vi "TopLevel_Process.vi"(7 "rendezvous ref":T11, 8 "error in":errorcluster, 9 "Str Refnum":refnum<vi>, 10 "LaunchData":refnum<user-event>, 11 "TopLevel in":refnum<class "TopLevel.lvclass">) -> (3 "TopLevel out":refnum<class "TopLevel.lvclass">)   [LabVIEW 2022 SP3, in "TopLevel.lvclass"]
uses:
  TopLevel.lvclass
  DAQWFE/LV_Source/DataTypes/TD LaunchData--cluster.ctl
  DAQWFE/LV_Source/DataTypes/TD LaunchState--enum.ctl
  Common/Controls/TD MasterConfiguration DLPC2--cluster.ctl
  Common/Controls/DLPC2_Path--Cluster.ctl
  Common/Controls/TD HeadColorPaneMappingAll--cluster.ctl
  Common/Controls/TD HeadColorPaneMapping--cluster.ctl
  Typedefs/SpitVoltages--Cluster.ctl
  Typedefs/PrimingMode APIData.ctl
  Typedefs/PurgeMode--Enum.ctl
  Typedefs/PrinterHeads--Enum.ctl
  Common/Controls/DLP_MaterialToHeadMapping--Cluster.ctl
  DLP2/DataTypes/DLP2_PrinterMaterialProperties.ctl
  Typedefs/API Event Data.ctl
  Typedefs/API Task State.ctl
  Typedefs/API Command Cluster.ctl
  Typedefs/API Command Enum.ctl
  Typedefs/Digilens Config Cluster.ctl
  Typedefs/Motor Controller Config Data.ctl
  IO/Typedefs/IO Config Data.ctl
  IO/Typedefs/DCON_DeviceConfig--Cluster.ctl
  IO/Typedefs/Channel Data.ctl
  GIS Printer/Typedefs/PrinterConfiguration--Cluster.ctl
  DAQWFE/LV_Source/Subsystems/DAQ/DataTypes/TD DAQ Settings--cluster.ctl
  DAQWFE/LV_Source/Subsystems/DAQ/DataTypes/TD DI Instrument Settings--cluster.ctl
  DAQWFE/LV_Source/Subsystems/DAQ/DataTypes/TD AI Instrument Settings--cluster.ctl
  DAQWFE/LV_Source/Subsystems/DAQ/DataTypes/TD AI InstSettings--cluster.ctl
  DAQWFE/LV_Source/Subsystems/DAQ/Process/ProcessSupport/TD SimAI Ranges--cluster.ctl
  IO/IO.lvclass
  GIS Printer/GIS Printer.lvclass
  Motor Controller/Motor Controller.lvclass
  Typedefs/Pre Purge API Data.ctl
  IO/Typedefs/ICP1-D0 Channel Names.ctl
  Typedefs/PrepurgeScanTracking--Cluster.ctl
  Database/Database.lvclass
  DLP2/DLP2.lvclass
  DAQWFE/LV_Source/Subsystems/DAQ/DataTypes/TD IO Node Definition--cluster.ctl
  DAQWFE/LV_Source/Subsystems/DAQ/DataTypes/TD DI Config--cluster.ctl
  DAQWFE/LV_Source/Subsystems/DAQ/DataTypes/TD DI Task--cluster.ctl
  DAQWFE/LV_Source/Subsystems/DAQ/DataTypes/TD DI Channel--cluster.ctl
  DAQWFE/LV_Source/Subsystems/DAQ/DataTypes/TD DO Config--cluster.ctl
  DAQWFE/LV_Source/Subsystems/DAQ/DataTypes/TD DO Channel--cluster.ctl
  DAQWFE/LV_Source/Subsystems/DAQ/DataTypes/TD AI Config--cluster.ctl
  DAQWFE/LV_Source/Subsystems/DAQ/DataTypes/TD AI Task--cluster.ctl
  DAQWFE/LV_Source/Subsystems/DAQ/DataTypes/TD AI Channel--cluster.ctl
  DAQWFE/LV_Source/Subsystems/DAQ/DataTypes/TD DataValueConversion--cluster.ctl
  DAQWFE/LV_Source/Subsystems/DAQ/DataTypes/TD AI DAQ Type--enum.ctl
  DAQWFE/LV_Source/Subsystems/DAQ/DataTypes/TD AI Force Bridge--cluster.ctl
  DAQWFE/LV_Source/Subsystems/DAQ/DataTypes/TD AO Config--cluster.ctl
  DAQWFE/LV_Source/Subsystems/DAQ/DataTypes/TD AO Channel--cluster.ctl
  DAQWFE/LV_Source/Subsystems/DAQ/DAQ.lvclass
  Common/Controls/DLPConfig_Initialization.ctl
  DLP2/DataTypes/DLP2_PrinterCompensationProperties.ctl
  DLP2/DataTypes/DLP2_PrinterHeadProperties.ctl
  Common/Controls/DLPConfig)Init_HeadPropertyAttr--Cluster.ctl
  Common/Controls/HeadHeaterTemperatureSet--Cluster.ctl
  Common/Controls/HeadHeaterTemperatureEnable--Cluster.ctl
  GIS Printer/Typedefs/PrintCmdParameters--Cluster.ctl
  GIS Printer/Typedefs/IdlePrintCmdParameters--Cluster.ctl
  Typedefs/HeadPrintData--Cluster.ctl
  IO/Typedefs/ICP2-DO Channel Names.ctl
  IO/Typedefs/ICP1-AO Channel Names.ctl
  DAQWFE/LV_Source/Support/DataQueues/DataQueues.lvclass
  <vilib>/Utility/error.llb/Trim Whitespace One-Sided.vi
  <vilib>/Utility/config.llb/Read Key (Path).vi
  Digilens DLP Gen2 UI .vi
  <userlib>/_OpenG.lib/array/array.llb/Filter 1D Array with Scalar (String)__ogtk.vi
  <vilib>/Utility/config.llb/NI_LVConfig.lvlib
panel:
  out "InkType Directory":T1[](array[typedef])
  out "data":T3={"Paths"={"DigiBit WG Design Folder"=path "", "Compensated GS Image Folder"=path "", "Nozzle GS Files Head 1"=path "", "Nozzle GS Files Head 2"=path "", "Nozzle GS Files Head 3"=path "", "Nozzle GS Files Head 4"=path "", "Nozzle GS Files Head 5"=path "", "Nozzle GS Files Head 6"=path ""}, "ColorPaneMapping"={"Head 1"={"Material"="", "ColorPane"=""}, "Head 2"={"Material"="", "ColorPane"=""}, "Head 3"={"Material"="", "ColorPane"=""}, "Head 4"={"Material"="", "ColorPane"=""}, "Head 5"={"Material"="", "ColorPane"=""}, "Head 6"={"Material"="", "ColorPane"=""}}, "Materials"=[], "ColorPlanes"=[], "SpitVoltages_Half"={"1"=0.0, "2"=0.0, "3"=0.0, "4"=0.0, "5"=0.0, "6"=0.0}, "SpitVoltages_Full"={"1"=0.0, "2"=0.0, "3"=0.0, "4"=0.0, "5"=0.0, "6"=0.0}, "SystemMode"=[], "PrimeModeConfig"=[], "Running Average Duration_s"=5.0}
  out "TO 3":bool[](array[boolean])
  out "TO 2":bool[](array[boolean])
  out "appended array":bool[](array[boolean])
  out "TO":bool[](array[boolean])
  out "error out":errorcluster
  in  "OK":bool
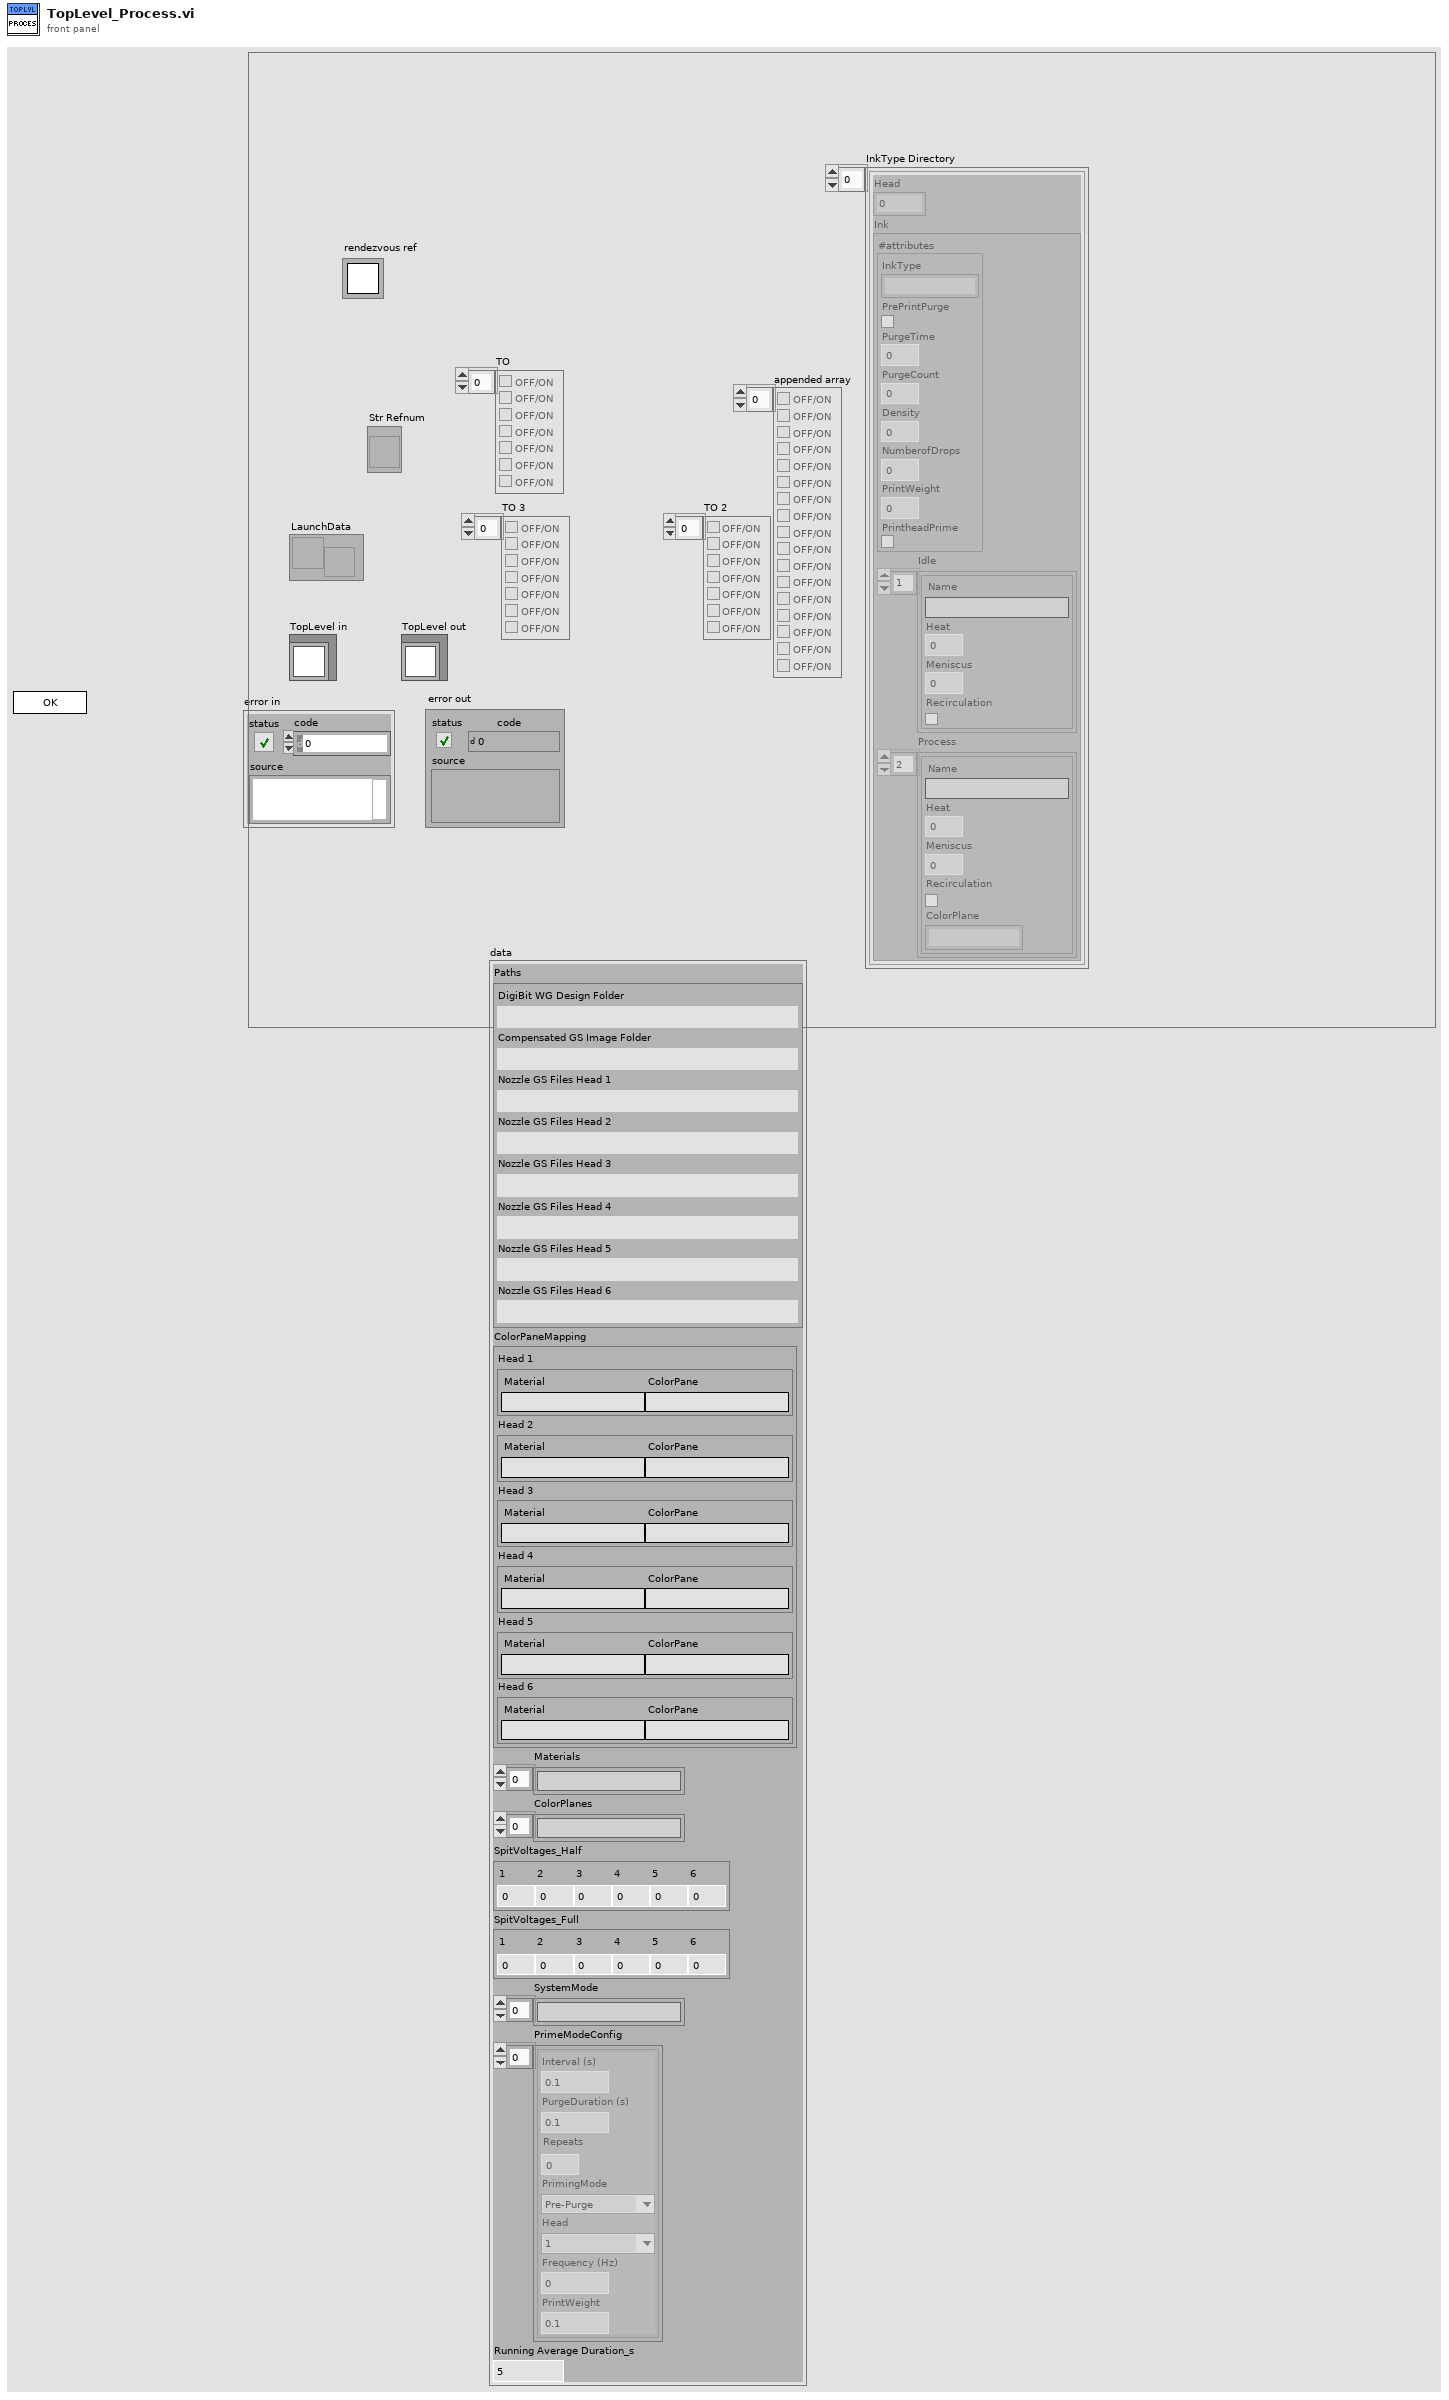
[diagram p1: front panel]
types:
  T1 = typedef "DLP_MaterialToHeadMapping--Cluster.ctl" = cluster{"Head":u8, "Ink":T2}
  T2 = typedef "DLP2_PrinterMaterialProperties.ctl" = cluster{"#attributes":cluster{"InkType":string, "PrePrintPurge":bool, "PurgeTime":dbl, "PurgeCount":i32, "Density":dbl, "NumberofDrops":i32, "PrintWeight":dbl, "PrintheadPrime":bool}, "Idle":cluster{"Name":string, "Heat":dbl, "Meniscus":dbl, "Recirculation":bool}[], "Process":cluster{"Name":string, "Heat":dbl, "Meniscus":dbl, "Recirculation":bool, "ColorPlane":string}[]}
  T3 = typedef "TD MasterConfiguration DLPC2--cluster.ctl" = cluster{"Paths":T4, "ColorPaneMapping":T5, "Materials":string[], "ColorPlanes":string[], "SpitVoltages_Half":T7, "SpitVoltages_Full":T7, "SystemMode":string[], "PrimeModeConfig":T8[], "Running Average Duration_s":dbl}
  T4 = typedef "DLPC2_Path--Cluster.ctl" = cluster{"DigiBit WG Design Folder":path, "Compensated GS Image Folder":path, "Nozzle GS Files Head 1":path, "Nozzle GS Files Head 2":path, "Nozzle GS Files Head 3":path, "Nozzle GS Files Head 4":path, "Nozzle GS Files Head 5":path, "Nozzle GS Files Head 6":path}
  T5 = typedef "TD HeadColorPaneMappingAll--cluster.ctl" = cluster{"Head 1":T6, "Head 2":T6, "Head 3":T6, "Head 4":T6, "Head 5":T6, "Head 6":T6}
  T6 = typedef "TD HeadColorPaneMapping--cluster.ctl" = cluster{"Material":string, "ColorPane":string}
  T7 = typedef "SpitVoltages--Cluster.ctl" = cluster{"1":dbl, "2":dbl, "3":dbl, "4":dbl, "5":dbl, "6":dbl}
  T8 = typedef "TopLevel.lvclass/PrimingMode APIData.ctl" = cluster{"Interval (s)":dbl, "PurgeDuration (s)":dbl, "Repeats":u8, "PrimingMode":T9, "Head":T10, "Frequency (Hz)":i32, "PrintWeight":dbl}
  T9 = typedef "PurgeMode--Enum.ctl" = enum16{"Pre-Purge", "Purge", "Spit", "Shake"}
  T10 = typedef "PrinterHeads--Enum.ctl" = enum16{"-1", "1", "2", "3", "4", "5", "6"}
  T11 = typedef "Rendezvous RefNum" = refnum<k1>
  T12 = cluster{"Initialized":bool, "LogFileFolder":path, "LogFile":path}
  T13 = typedef "TopLevel.lvclass/API Command Cluster.ctl" = cluster{"Command":T14, "Arguments":string, "Data":variant}
  T14 = typedef "TopLevel.lvclass/API Command Enum.ctl" = enum16{"Execute Printer Commands", "Pre Purge", "Enable Ink Ch-1", "Enable Ink Ch-2", "Enable Ink Ch-3", "Enable Ink Ch-4", "Enable Ink Ch-5", "Enable Ink Ch-6", "Disable Ink Ch-1", "Disable Ink Ch-2", "Disable Ink Ch-3", "Disable Ink Ch-4", "Disable Ink Ch-5", "Disable Ink Ch-6", "ExecuteIdlePrintCycle", "StopIdlePrintCycle", "Abort", "LoadDLP2GUIConfig", "SaveDLP2GUIConfig", "PrimingMode", "SetHeadTemperature", "EnableHead", "EnableHeadHeat", "SetSystemMode", "HeadPrint", "AbortAll", "Send Printer String", "WriteInitXML"}
  T15 = typedef "TopLevel.lvclass/API Event Data.ctl" = cluster{"Task":cluster{"Time Stamp":timestamp, "Timeout (ms)":u32, "Task State":T16, "Task Error":errorcluster, "Task ID":string}, "Command":variant, "Return Value":variant}
  T16 = typedef "TopLevel.lvclass/API Task State.ctl" = enum16{"Completed", "Errored", "Pending"}
  T17 = enum32{"invalid app kind", "Development System", "Run Time System", "Student Edition", "Embedded LabVIEW", "Evaluation", "Custom"}
  T18 = typedef "DLPConfig_Initialization.ctl" = cluster{"PrinterInitialization":cluster{"Printer":cluster{"#attributes":cluster{"Name":string}}, "VacPumpSet":cluster{"#attributes":cluster{"VacPumpEnable":bool, "VacPumpSpeed":dbl}}, "HIBEnable":cluster{"#attributes":cluster{"HIB1Enable":bool, "HIB2Enable":bool, "HIB3Enable":bool, "HIB4Enable":bool, "HIB5Enable":bool, "HIB6Enable":bool}}, "PrinterCompensation":T19}, "HeadSet":cluster{"HeadProperties":T20[]}, "InkSet":cluster{"Ink":T2[]}, "Troubleshooting":cluster{"PMBLogging":cluster{"#attributes":cluster{"PMBMonitorDuringPrint":bool, "PMBMonitorDuringIdle":bool, "LogSwatheInputData":bool, "LogSwatheOutputData":bool, "LogPrintheadColourPlanes":bool, "LogPMBCommunication":bool, "LogSimulatedOutput":bool, "LogAllPMBCommunicationData":bool, "LogPMBSpace":bool, "ExtendedPMBSpaceLogging":bool, "LogPMBWriteSpeed":bool, "LogUsbRetries":bool}}, "HIBLogging":cluster{"#attributes":cluster{"HIBMonitoringDuringPrint":bool, "HIBMonitoringLog":bool}}}}
  T19 = typedef "DLP2_PrinterCompensationProperties.ctl" = cluster{"#attributes":cluster{"AppName":string, "PrintWeightMultiplier":dbl, "Rotation":bool, "Driver":string, "Server":string, "Database":string, "User":string, "Password":string}}
  T20 = typedef "DLP2_PrinterHeadProperties.ctl" = cluster{"#attributes":T21}
  T21 = typedef "DLPConfig)Init_HeadPropertyAttr--Cluster.ctl" = cluster{"HeadNumber":u8, "Material":string, "HeadLocalX":dbl, "HeadLocalY":dbl, "HeadRotationAngle":dbl, "VH2L_Hi":dbl, "VH2R_Hi":dbl, "VH1LA_Hi":dbl, "VH1LB_Hi":dbl, "VH1RA_Hi":dbl, "VH1RB_Hi":dbl, "VH2L_Lo":dbl, "VH2R_Lo":dbl, "VH1LA_Lo":dbl, "VH1LB_Lo":dbl, "VH1RA_Lo":dbl, "VH1RB_Lo":dbl}
  T22 = typedef "DAQ.lvclass/TD IO Node Definition--cluster.ctl" = cluster{"DI Config":T23, "DO Config":T26, "AI Config":T28, "AO Config":T34}
  T23 = typedef "DAQ.lvclass/TD DI Config--cluster.ctl" = cluster{"DI Tasks":T24[]}
  T24 = typedef "DAQ.lvclass/TD DI Task--cluster.ctl" = cluster{"DI TaskName":string, "DI Channels":T25[]}
  T25 = typedef "DAQ.lvclass/TD DI Channel--cluster.ctl" = cluster{"DevName":string, "IOName":string, "IOPath":string, "SchemName":string, "logic":enum16{"Lo", "Hi"}, "Index":i32}
  T26 = typedef "DAQ.lvclass/TD DO Config--cluster.ctl" = cluster{"DO Channels":T27[]}
  T27 = typedef "DAQ.lvclass/TD DO Channel--cluster.ctl" = cluster{"DevName":string, "IOName":string, "IOPath":string, "SchemName":string, "logic":enum16{"Lo", "Hi"}, "DAQmx Task":refnum<k21>}
  T28 = typedef "DAQ.lvclass/TD AI Config--cluster.ctl" = cluster{"AI Tasks":T29[]}
  T29 = typedef "DAQ.lvclass/TD AI Task--cluster.ctl" = cluster{"AI TaskName":string, "AI Channels":T30[]}
  T30 = typedef "DAQ.lvclass/TD AI Channel--cluster.ctl" = cluster{"DevName":string, "IOName":string, "IOPath":string, "SchemName":string, "MinValue":dbl, "MaxValue":dbl, "Terminal Configuration":i32, "Index":i32, "Conversion":T31, "AIType":T32, "Force Bridge":T33}
  T31 = typedef "DAQ.lvclass/TD DataValueConversion--cluster.ctl" = cluster{"MaxSignal":dbl, "MinSignal":dbl, "MaxEngUnit":dbl, "MinEngUnit":dbl, "ScaleOffset":dbl, "negate":bool}
  T32 = typedef "DAQ.lvclass/TD AI DAQ Type--enum.ctl" = enum16{"Voltage", "Current", "Strain Gage", "Force Bridge"}
  T33 = typedef "DAQ.lvclass/TD AI Force Bridge--cluster.ctl" = cluster{"bridge information":cluster{"bridge configuration":i32, "voltage excitation source":i32, "voltage excitation value":dbl, "nominal bridge resistance":dbl}, "scaling information":cluster{"first electrical value":dbl, "second electrical value":dbl, "electrical units":i32, "first physical value":dbl, "second physical value":dbl, "physical units":i32}}
  T34 = typedef "DAQ.lvclass/TD AO Config--cluster.ctl" = cluster{"AO Channels":T35[]}
  T35 = typedef "DAQ.lvclass/TD AO Channel--cluster.ctl" = cluster{"DevName":string, "IOName":string, "IOPath":string, "SchemName":string, "Vmin":dbl, "Vmax":dbl, "Conversion":T31, "DAQmx Task":refnum<k21>}
  T36 = typedef "TopLevel.lvclass/Pre Purge API Data.ctl" = cluster{"Purge Channel Name":T37, "GIS File Path":path, "Duration (s)":dbl, "PurgeDuration (s)":dbl, "Repeats":u8}
  T37 = typedef "IO.lvclass/ICP1-D0 Channel Names.ctl" = enum16{"None", "Meniscus Pressure Reg PWR - R1", "Meniscus Pressure Reg PWR - R2", "Meniscus Pressure Reg PWR - R3", "Meniscus Pressure Reg PWR - R4", "Meniscus Pressure Reg PWR - R5", "Meniscus Pressure Reg PWR - R6", "Clear Stage Alarm", "Servo ON", "Purge Valve Open - R1", "Purge Valve Open - R2", "Purge Valve Open - R3", "Purge Valve Open - R4", "Purge Valve Open - R5", "Purge Valve Open - R6"}
  T38 = typedef "TopLevel.lvclass/Digilens Config Cluster.ctl" = cluster{"Motion Controller":T39, "IO Config":T40, "PrinterConfiguration":T43, "DAQ Settings":T44}
  T39 = typedef "Motor Controller.lvclass/Motor Controller Config Data.ctl" = cluster{"Motor IP Addresss":string, "Current Position":i32, "Pulse_Per_mm":i32, "PrePrint":dbl[], "Load Position_mm":i32, "Laminate Position_mm":i32}
  T40 = typedef "IO.lvclass/IO Config Data.ctl" = cluster{"DAQDevices":T41[], "DI Channels":T42[], "DO Channels":T42[], "Material Names":string[], "AI Channels":T42[], "AO Channels":T42[]}
  T41 = typedef "IO.lvclass/DCON_DeviceConfig--Cluster.ctl" = cluster{"COM":string, "DeviceName":string, "BaudRate":u32, "Number of Channels":i32, "DeviceAddress":i32, "Enable":bool}
  T42 = typedef "IO.lvclass/Channel Data.ctl" = cluster{"Channel Name":string, "Device Name":string, "Channel No":string}
  T43 = typedef "GIS Printer.lvclass/PrinterConfiguration--Cluster.ctl" = cluster{"IPAddress":string, "Move Stage on RTP Command?":bool, "Stage Move Position":string, "PH1-Prime Path":path, "PH2-Prime Path":path, "PH3-Prime Path":path, "PH4-Prime Path":path, "PH5-Prime Path":path, "PH6-Prime Path":path, "PrintScriptsFolder":path, "PurgeScriptsFolder":path, "StageScriptsFolder":path, "PH1-HeatOn Path":path, "PH2-HeatOn Path":path, "PH3-HeatOn Path":path, "PH4-HeatOn Path":path, "PH5-HeatOn Path":path, "PH6-HeatOn Path":path, "PH1-HeatOff Path":path, "PH2-HeatOff Path":path, "PH3-HeatOff Path":path, "PH4-HeatOff Path":path, "PH5-HeatOff Path":path, "PH6-HeatOff Path":path}
  T44 = typedef "DAQ.lvclass/TD DAQ Settings--cluster.ctl" = cluster{"Simulate DAQ":bool, "DI Settings":T45[], "AI Settings":T46[], "Relay IONames":string[], "AO IONames":string[], "AO NChan SingleTask":bool}
  T45 = typedef "DAQ.lvclass/TD DI Instrument Settings--cluster.ctl" = cluster{"Disable":bool, "DI TaskName":string, "DI RefreshIntv":i32}
  T46 = typedef "DAQ.lvclass/TD AI Instrument Settings--cluster.ctl" = cluster{"Disable":bool, "AI TaskName":string, "AI InstSettings":T47, "SimAI Ranges":T48}
  T47 = typedef "DAQ.lvclass/TD AI InstSettings--cluster.ctl" = cluster{"DaqRate":dbl, "NumSamples":i32}
  T48 = typedef "DAQ.lvclass/TD SimAI Ranges--cluster.ctl" = cluster{"lo":dbl, "hi":dbl}
  T49 = enum32{"Invalid", "Standard", "Closed", "Hidden", "Minimized", "Maximized"}
  T50 = typedef "HeadHeaterTemperatureSet--Cluster.ctl" = cluster{"Head":T10, "SetPoint":dbl}
  T51 = typedef "HeadHeaterTemperatureEnable--Cluster.ctl" = cluster{"Head":T10, "Enable":bool}
  T52 = typedef "PrintCmdParameters--Cluster.ctl" = cluster{"Command File Path":path, "No. of Print Repeats":i32, "HomeOnComplete":bool}
  T53 = typedef "IdlePrintCmdParameters--Cluster.ctl" = cluster{"Command File Path":path, "IdleMode":bool, "IdleCycleInterval(s)":dbl}
  T54 = typedef "TopLevel.lvclass/HeadPrintData--Cluster.ctl" = cluster{"PrintImageFile":string, "PrintPass":u8, "EncoderSource":string, "PrintGoSource":string, "Head":T10}
  T55 = typedef "IO.lvclass/ICP1-AO Channel Names.ctl" = enum16{"None", "Meniscus Pressure Set - R1", "Meniscus Pressure Set - R2", "Meniscus Pressure Set - R3", "Meniscus Pressure Set - R4", "Meniscus Pressure Set - R5", "Meniscus Pressure Set - R6", "Meniscus Vac Pump Speed"}
  T56 = typedef "IO.lvclass/ICP2-DO Channel Names.ctl" = enum16{"None", "Meniscus Valve Open - R1", "Meniscus Valve Open - R2", "Meniscus Valve Open - R3", "Meniscus Valve Open - R4", "Meniscus Valve Open - R5", "Meniscus Valve Open - R6", "Ink Flow Valve Open - R1", "Ink Flow Valve Open - R2", "Ink Flow Valve Open - R3", "Ink Flow Valve Open - R4", "Ink Flow Valve Open - R5", "Ink Flow Valve Open - R6", "SW_LED - Ink Valve - R1", "SW_LED - Ink Valve - R2", "SW_LED - Ink Valve - R3", "Recirc Pump On - R1", "Recirc Pump On - R2", "Recirc Pump On - R3", "Recirc Pump On - R4", "Recirc Pump On - R5", "Recirc Pump On - R6", "SW_LED - Ink Valve - R4", "SW_LED - Ink Valve - R5", "SW_LED - Ink Valve - R6"}
  T57 = typedef "TD LaunchData--cluster.ctl" = cluster{"Time Stamp":timestamp, "LaunchState":T58, "Error":errorcluster}
  T58 = typedef "TD LaunchState--enum.ctl" = enum16{"Started", "Stopped"}
  T59 = cluster{"Time Stamp":timestamp, "Timeout (ms)":u32, "Task State":T16, "Task Error":errorcluster, "Task ID":string}
  T60 = typedef "PrepurgeScanTracking--Cluster.ctl" = cluster{"TotalRepeats":i32, "CurrentScan":i32}
  T61 = cluster{"Core":cluster{"Current VI Reference":refnum<vi>, "Close Panel on Exit?":bool}, "TopLevel in":refnum<class "TopLevel.lvclass">, "Tasks":T15[], "TO":i32, "API Executed Event":refnum<user-event>, "API Return Event":refnum<user-event>, "Task Start ms":u32, "Current Task. Return Value":variant, "StartupPath":path, "Digilens IPLC Config":T38, "Current Task":T13, "IO":refnum<class "IO.lvclass">, "GIS Printer":refnum<class "GIS Printer.lvclass">, "Motor Controller":refnum<class "Motor Controller.lvclass">, "Printer Command File Path":path, "Pre Purge API Data":T36, "PPScanTrk":T60, "PrintScanTrk":T60, "IdleTimer":dbl, "Idle Mode":bool, "HomeOnComplete":bool, "Database":refnum<class "Database.lvclass">, "DLP2":refnum<class "DLP2.lvclass">, "MasterConfigurationDLPC2":T3, "Digilens Config File Path":path, "DLP2 ConfigPath":path, "GIS Commands":string[], "PrinterModeAPI Data":T8, "LaunchData":refnum<user-event>, "DAQConfigPath":path, "IO Nodes":T22, "DAQ":refnum<class "DAQ.lvclass">, "PMScanTrk":T60, "DLP":T18, "Str Refnum":refnum<vi>}
  T62 = typedef "NI_LVConfig.lvlib/Config Data RefNum.ctl" = refnum<k1>
  T63 = cluster{"Current VI Reference":refnum<vi>, "Close Panel on Exit?":bool}
  T64 = typedef "TD Pathnames--cluster.ctl" = cluster{"RunTimeSys?":bool, "AppFolder":path, "ExecutablePath":path, "ConfigFolder":path, "DataLogFolder":path, "SystemLogFolder":path, "SeqFolder":path, "MainStartupPathname":path, "MainUIPathname":path, "SystemEventsFile":path, "SeqEventsFile":path, "Config SettingsFile":path, "DAQ IOConfigFile":path, "SystemSimulation":bool, "DLPUIConfigFile":path, "PrinterInitXMLFile":path, "PersistentXMLFile":path, "Error Log Folder":path, "RecipeXMLFolder":path, "CalibrationRecipeXMLFolder":path}
  T65 = typedef "PersistentData--Cluster.ctl" = cluster{"ToolIdle":bool, "Meniscus Vac Pump Speed":dbl, "InkChEnable":cluster{"Enable Ink Ch-1":bool, "Enable Ink Ch-2":bool, "Enable Ink Ch-3":bool, "Enable Ink Ch-4":bool, "Enable Ink Ch-5":bool, "Enable Ink Ch-6":bool}, "HeatEnable":cluster{"Heater-1 Off":bool, "Heater-2 Off":bool, "Heater-3 Off":bool, "Heater-4 Off":bool, "Heater-5 Off":bool, "Heater-6 Off":bool}, "MiniscusPressure":cluster{"Meniscus Pressure Set - R1":dbl, "Meniscus Pressure Set - R2":dbl, "Meniscus Pressure Set - R3":dbl, "Meniscus Pressure Set - R4":dbl, "Meniscus Pressure Set - R5":dbl, "Meniscus Pressure Set - R6":dbl}, "RecircPumpFlow":cluster{"Recirc Pump Flow Set - R1":dbl, "Recirc Pump Flow Set - R2":dbl, "Recirc Pump Flow Set - R3":dbl, "Recirc Pump Flow Set - R4":dbl, "Recirc Pump Flow Set - R5":dbl, "Recirc Pump Flow Set - R6":dbl}}
  T66 = typedef "DAQ.lvclass/TD PublicEvents--cluster.ctl" = cluster{"DaqOutputCmd Ev":refnum<user-event>, "stop process":refnum<user-event>, "DAQ.AsyncCmd Event":refnum<user-event>, "DAQStateChanged Event":refnum<user-event>, "DAQ.AsyncMsg Event":refnum<user-event>, "DAQ_DO_StatusEvent":refnum<user-event>, "DIStateChangeEv":refnum<user-event>, "UI StateChanged":refnum<user-event>, "PurgeTimerEvent":refnum<user-event>}
  T67 = typedef "TopLevel.lvclass/UserEvents.ctl" = cluster{"API Incoming Event":refnum<user-event>, "API Executed Event":refnum<user-event>, "API Return Event":refnum<user-event>, "Exit Event":refnum<user-event>, "StatusChanged":refnum<user-event>, "DLP GUI Config Changed":refnum<user-event>, "AppEvent":refnum<user-event>, "Login Event":refnum<user-event>, "HeadPrimeStatusEvent":refnum<user-event>}
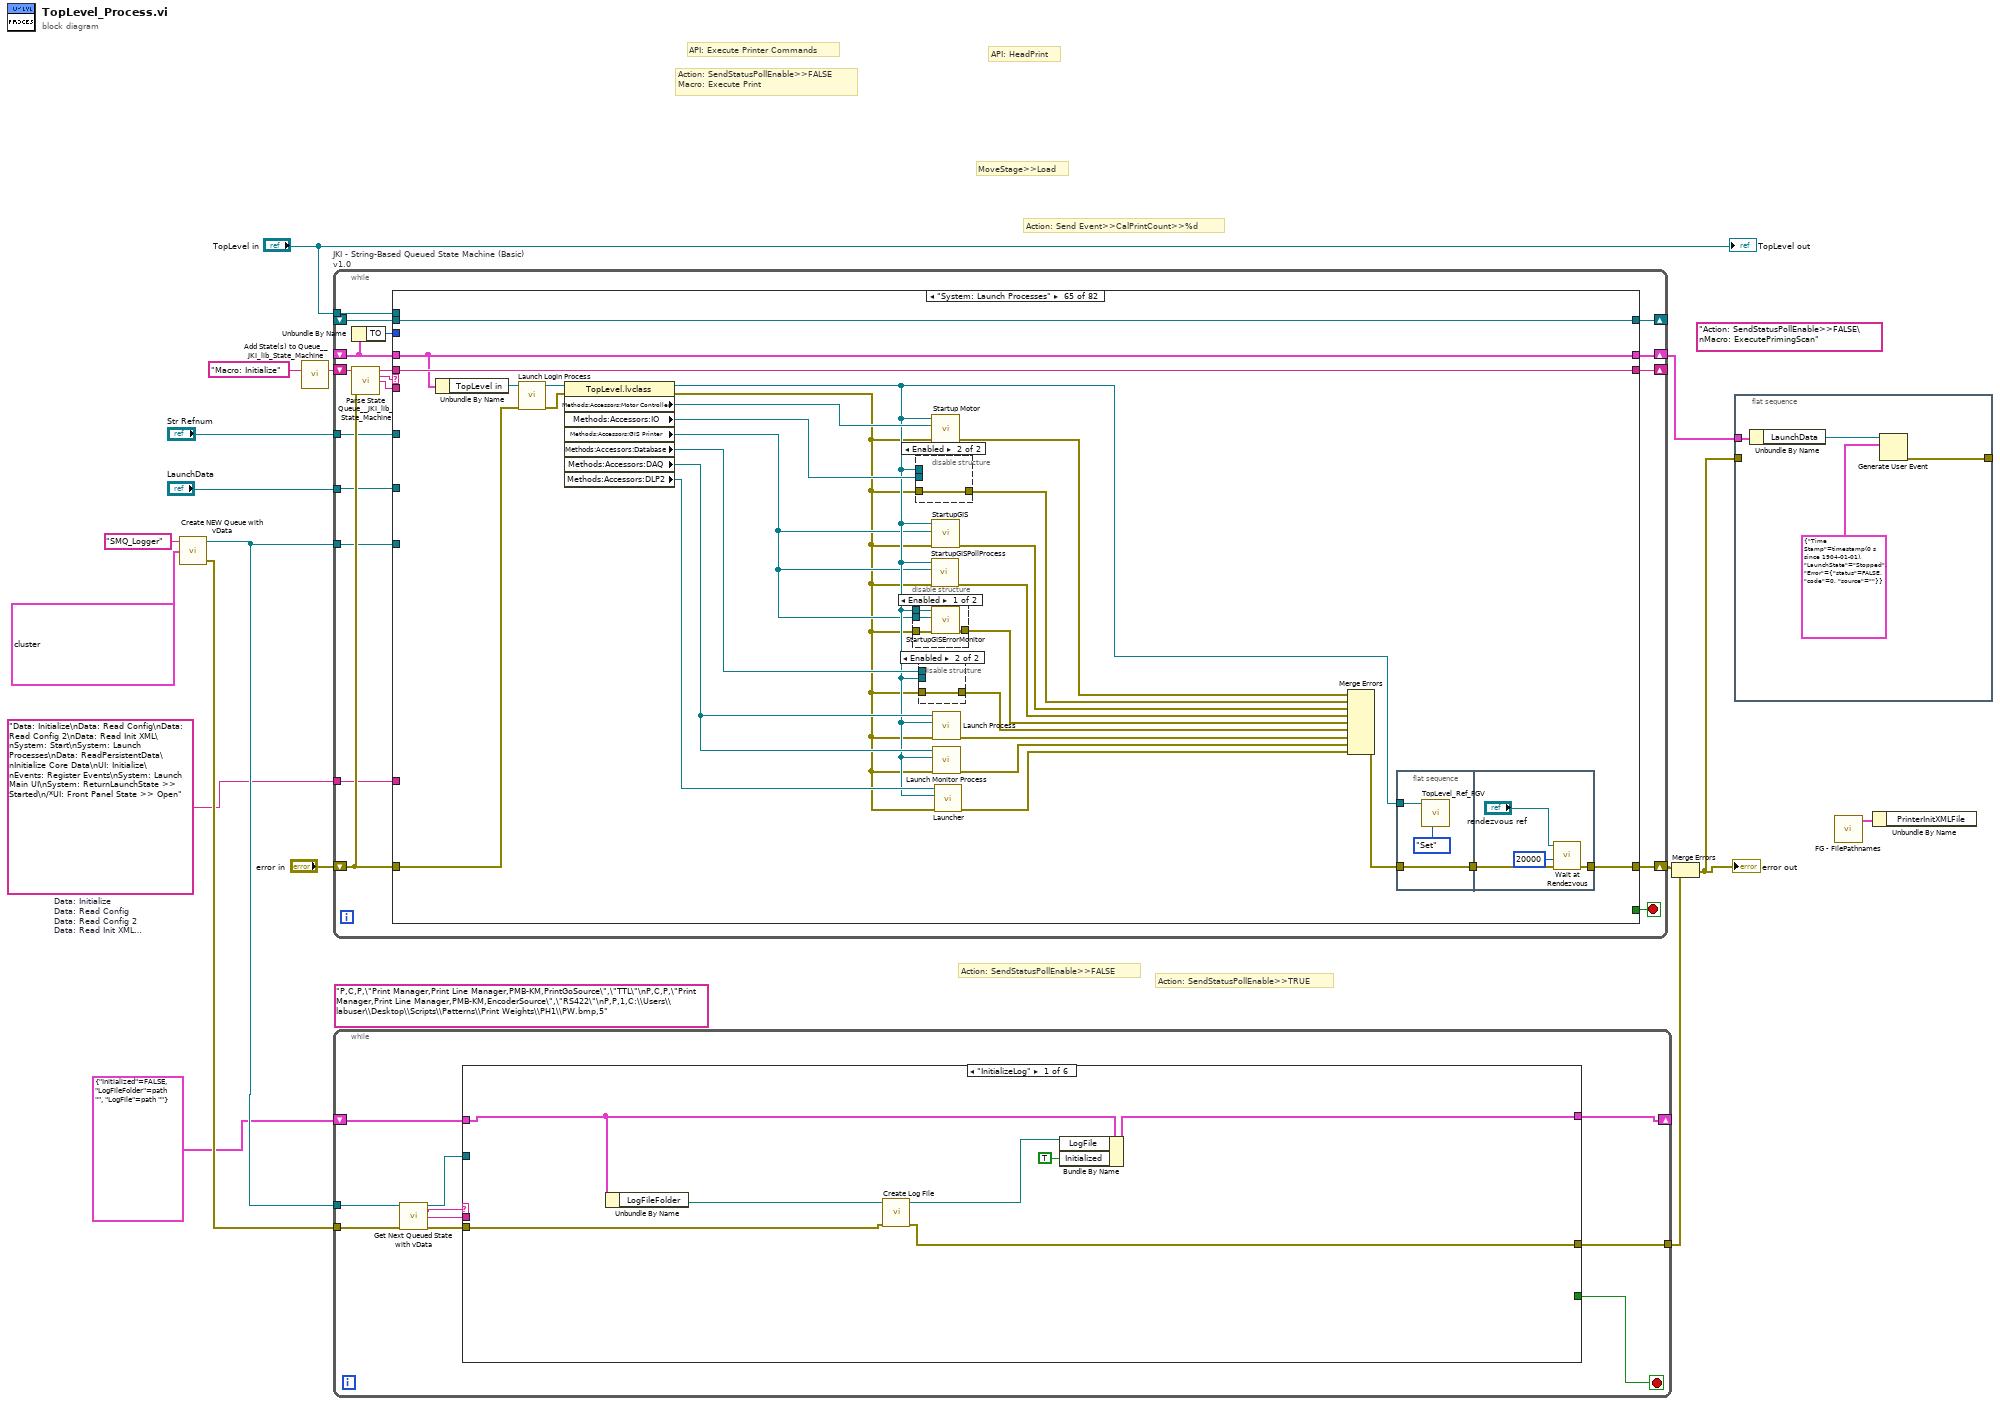
[diagram p0: block diagram]
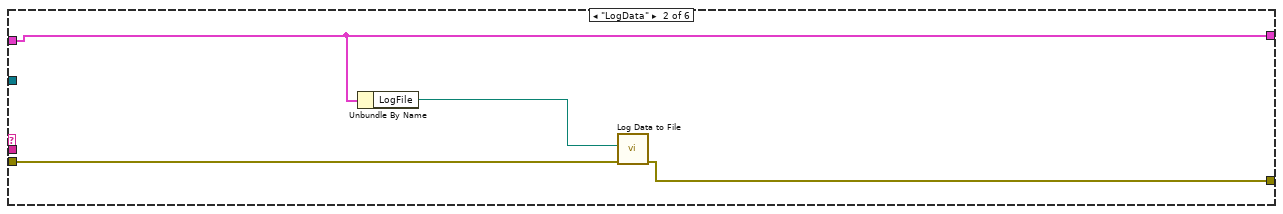
[diagram p2: hidden frame]
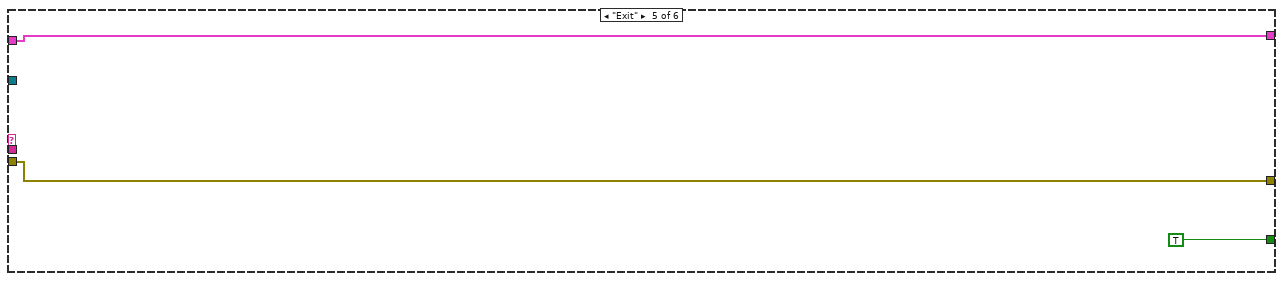
[diagram p5: hidden frame]
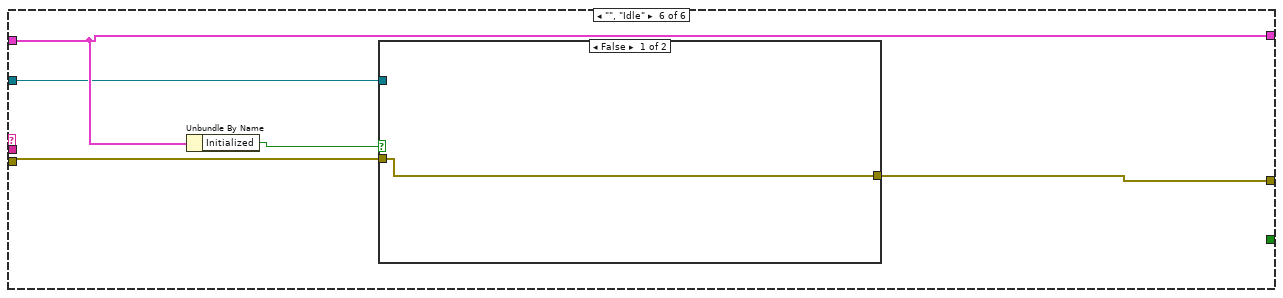
[diagram p6: hidden frame]
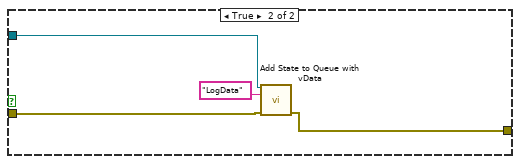
[diagram p7: hidden frame]
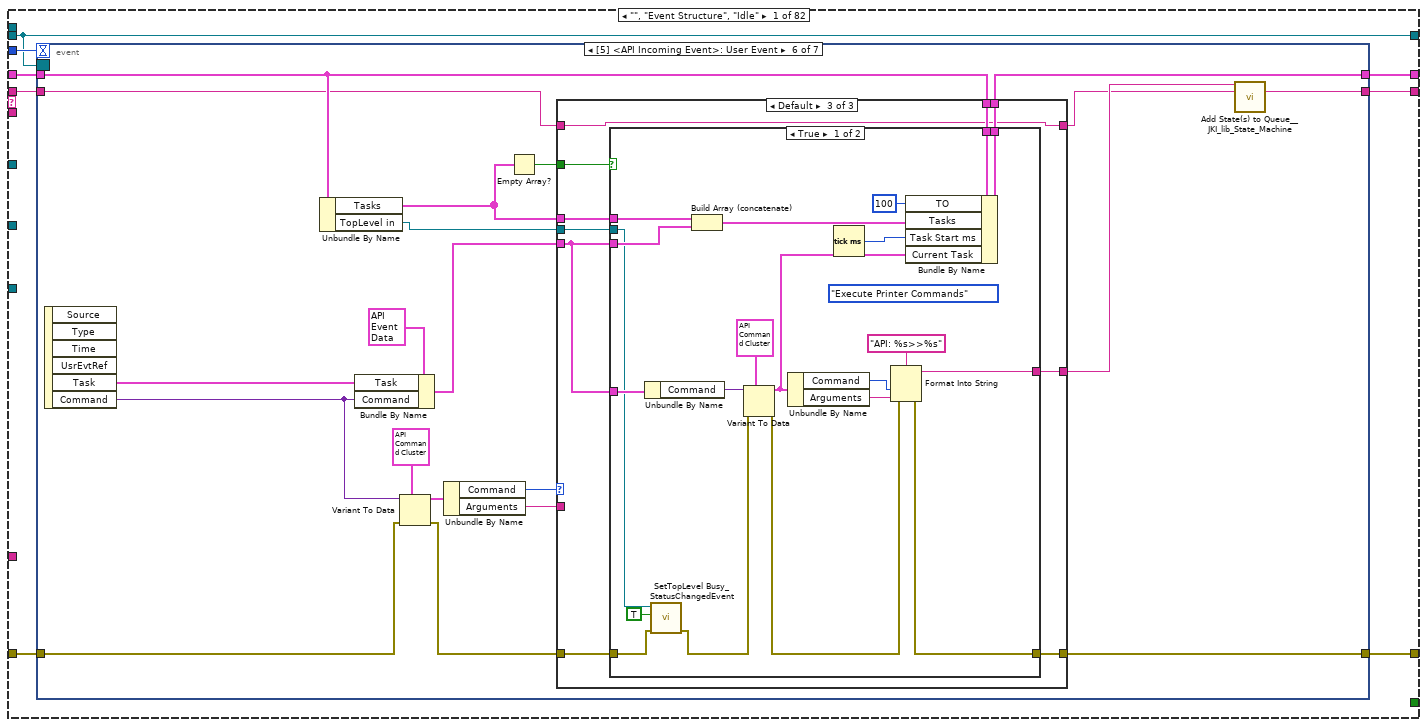
[diagram p8: hidden frame]
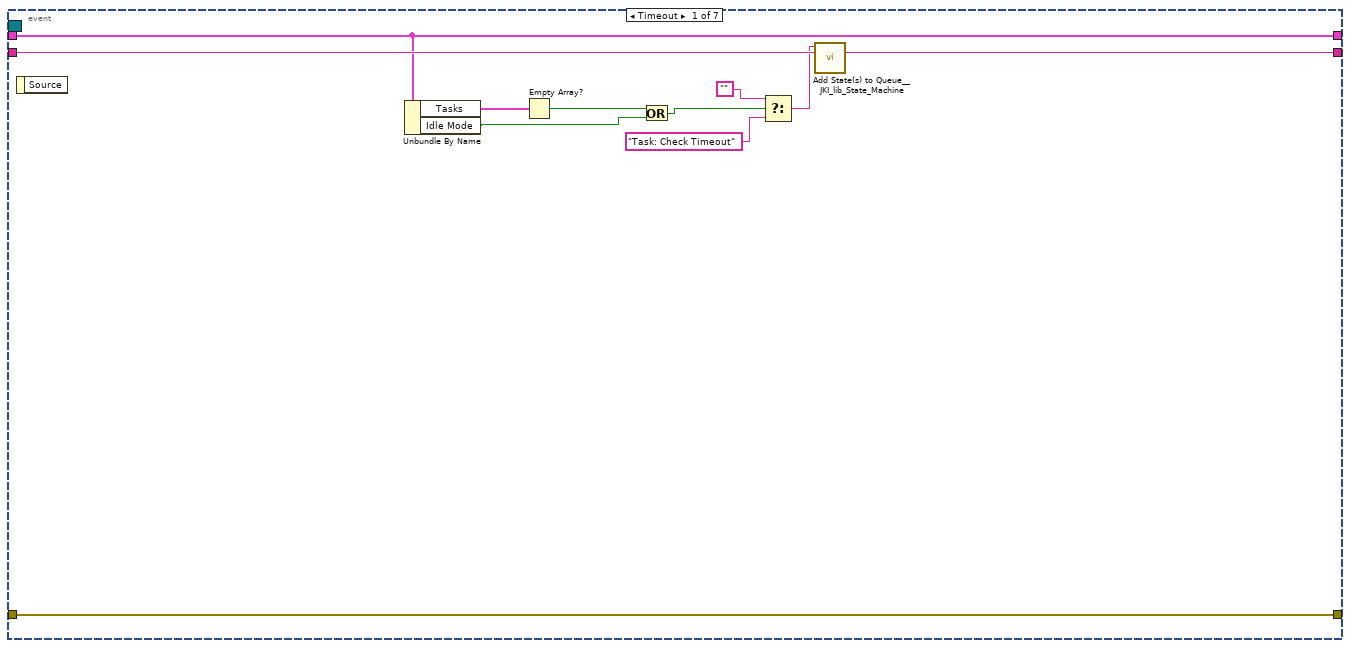
[diagram p9: hidden frame]
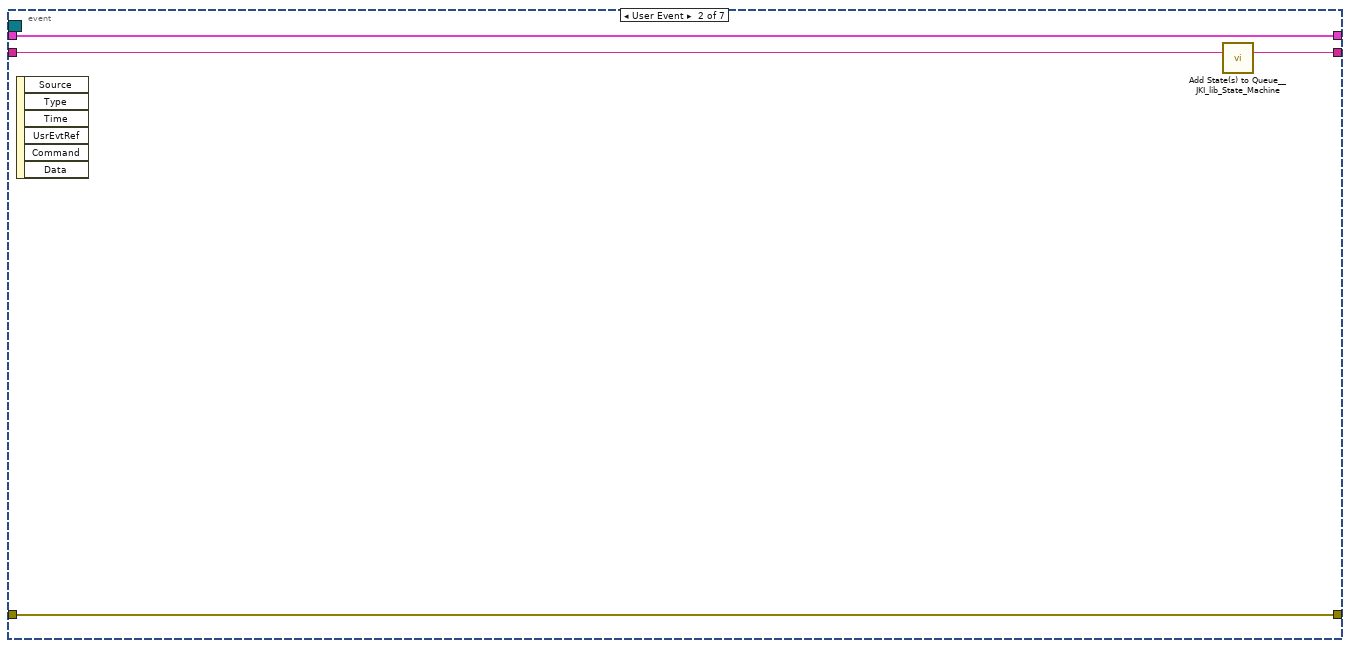
[diagram p10: hidden frame]
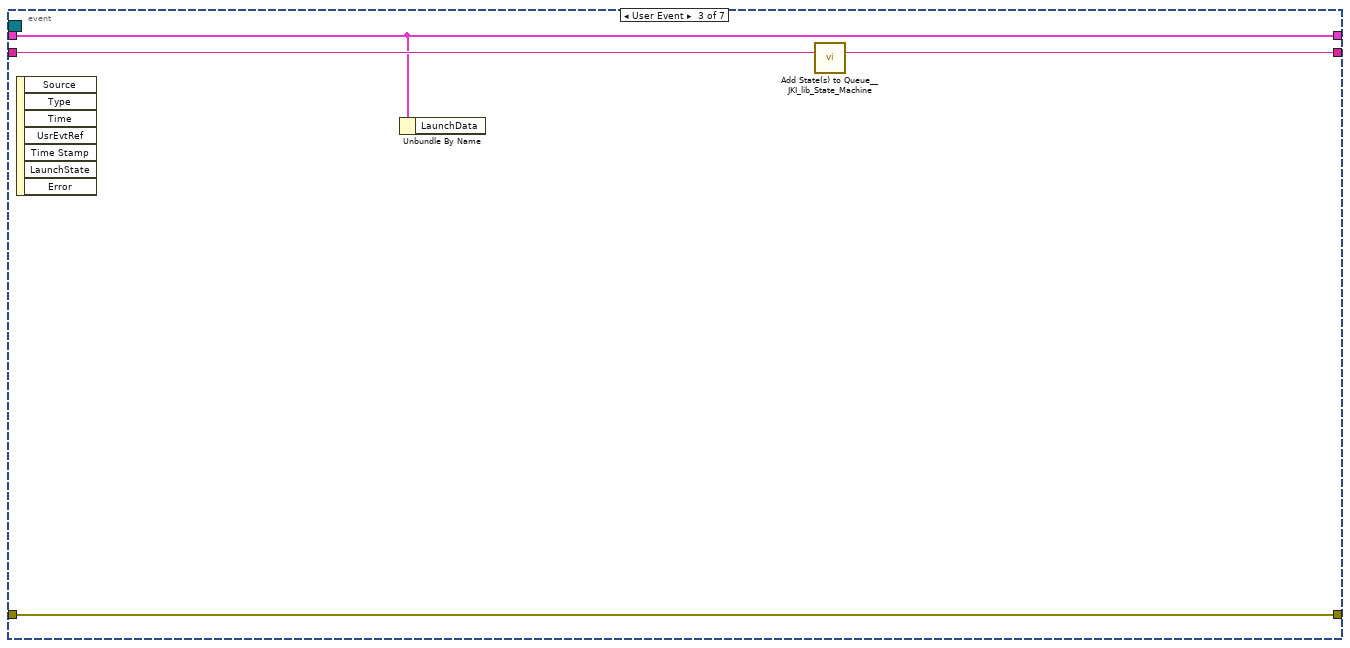
[diagram p11: hidden frame]
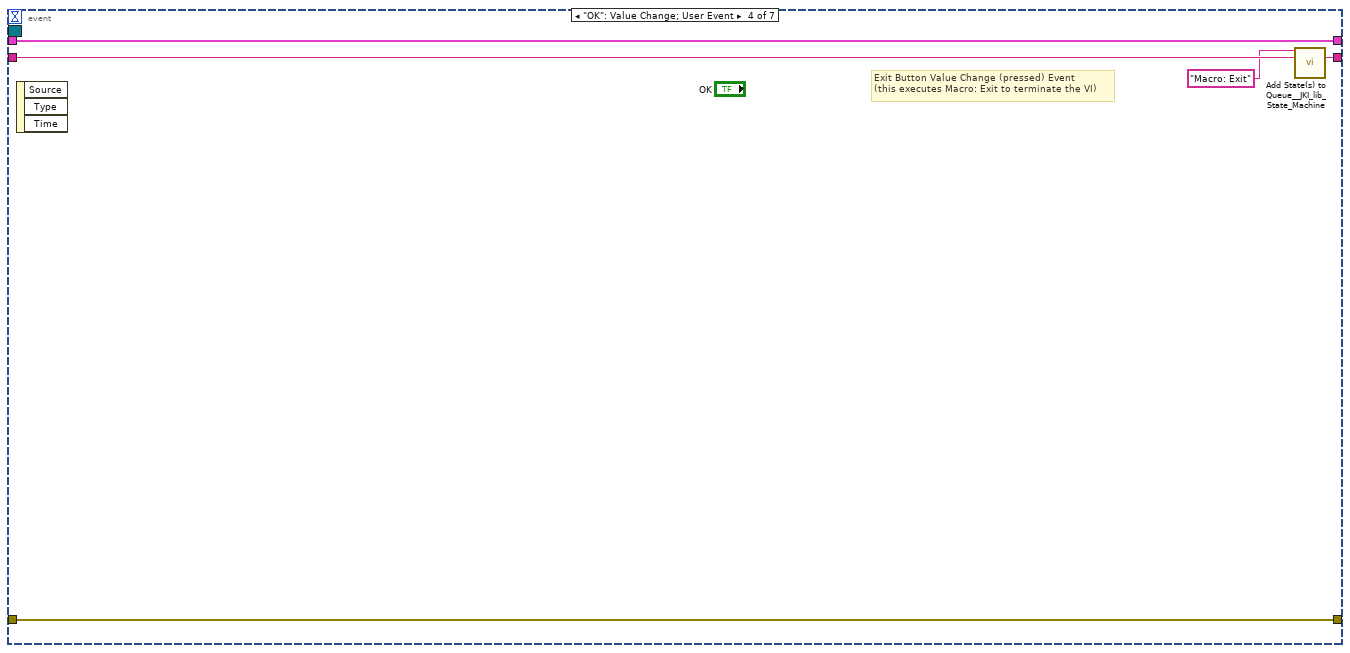
[diagram p12: hidden frame]
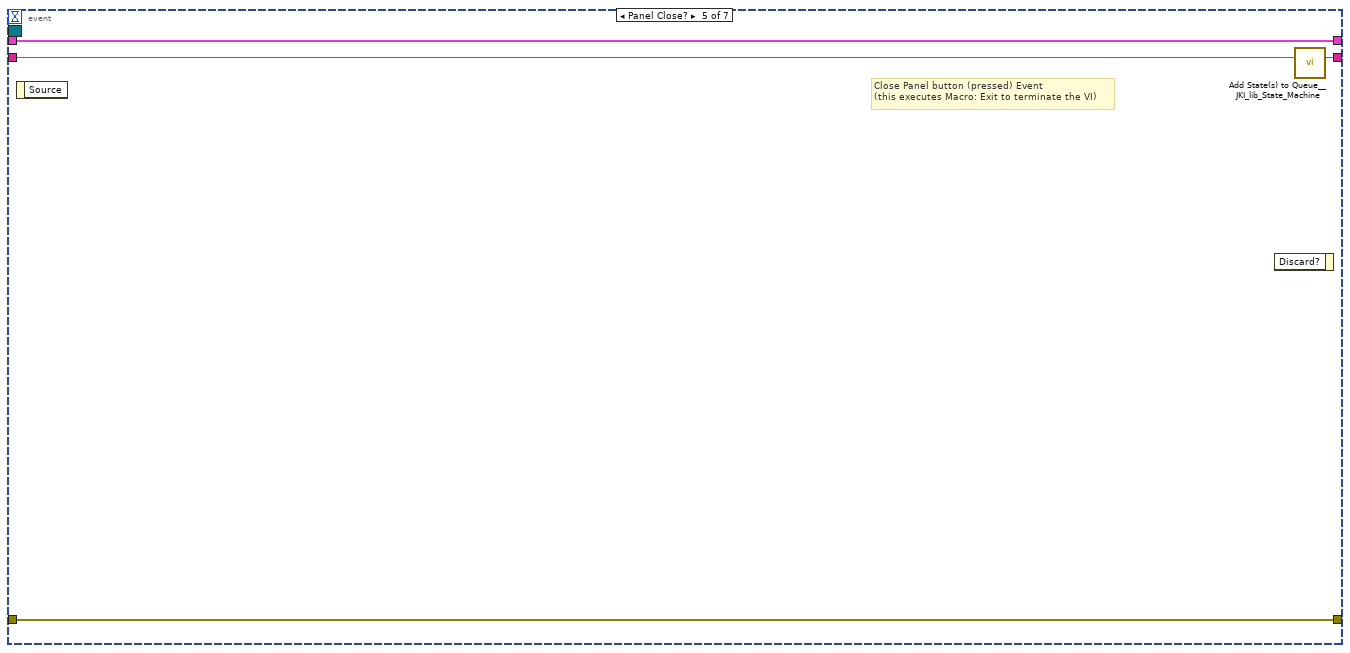
[diagram p13: hidden frame]
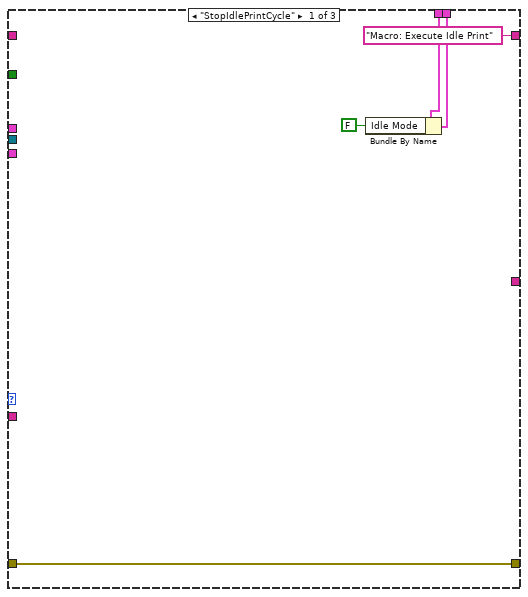
[diagram p14: hidden frame]
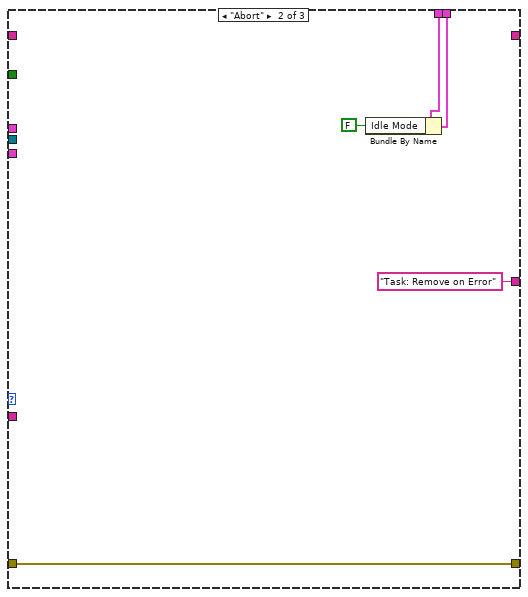
[diagram p15: hidden frame]
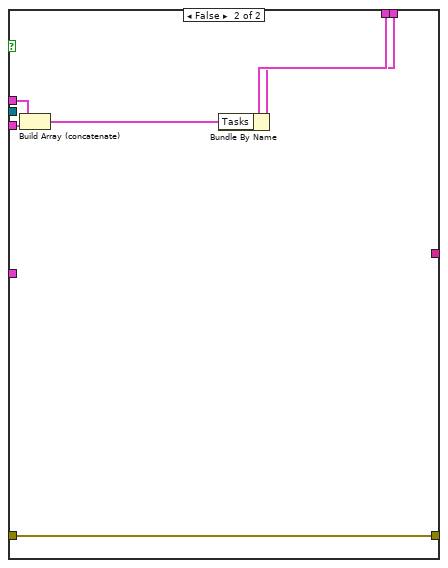
[diagram p16: hidden frame]
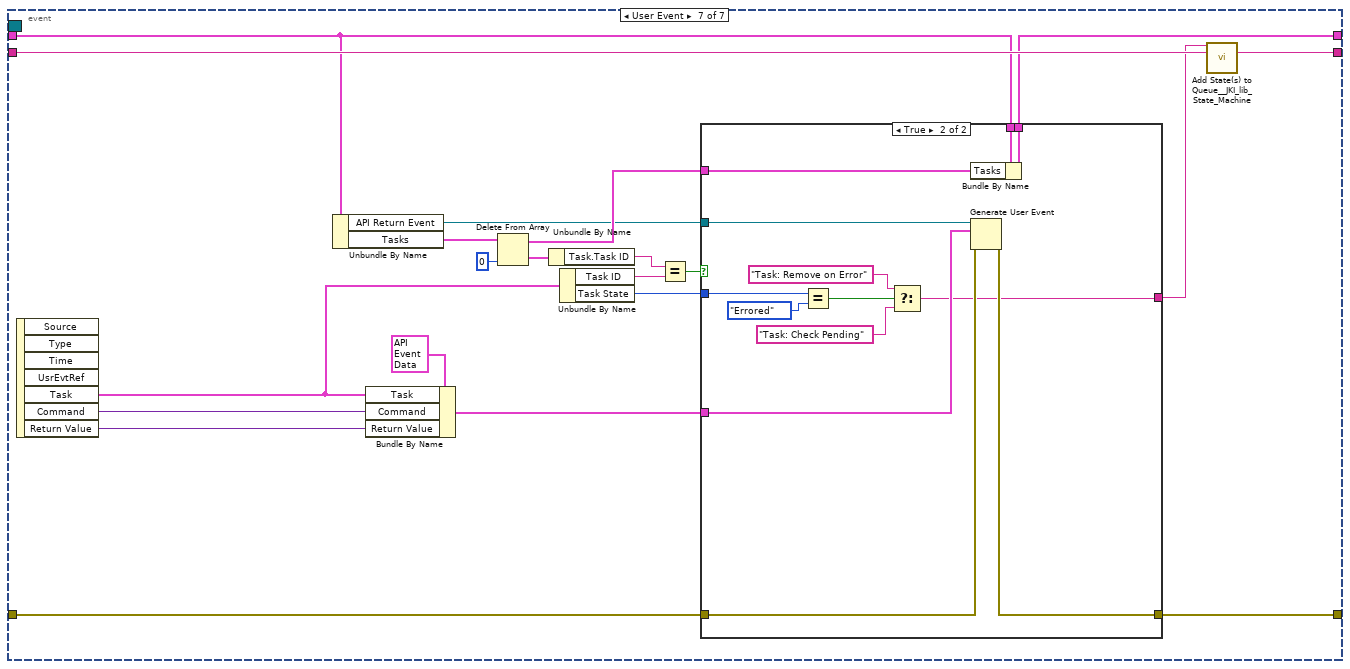
[diagram p17: hidden frame]
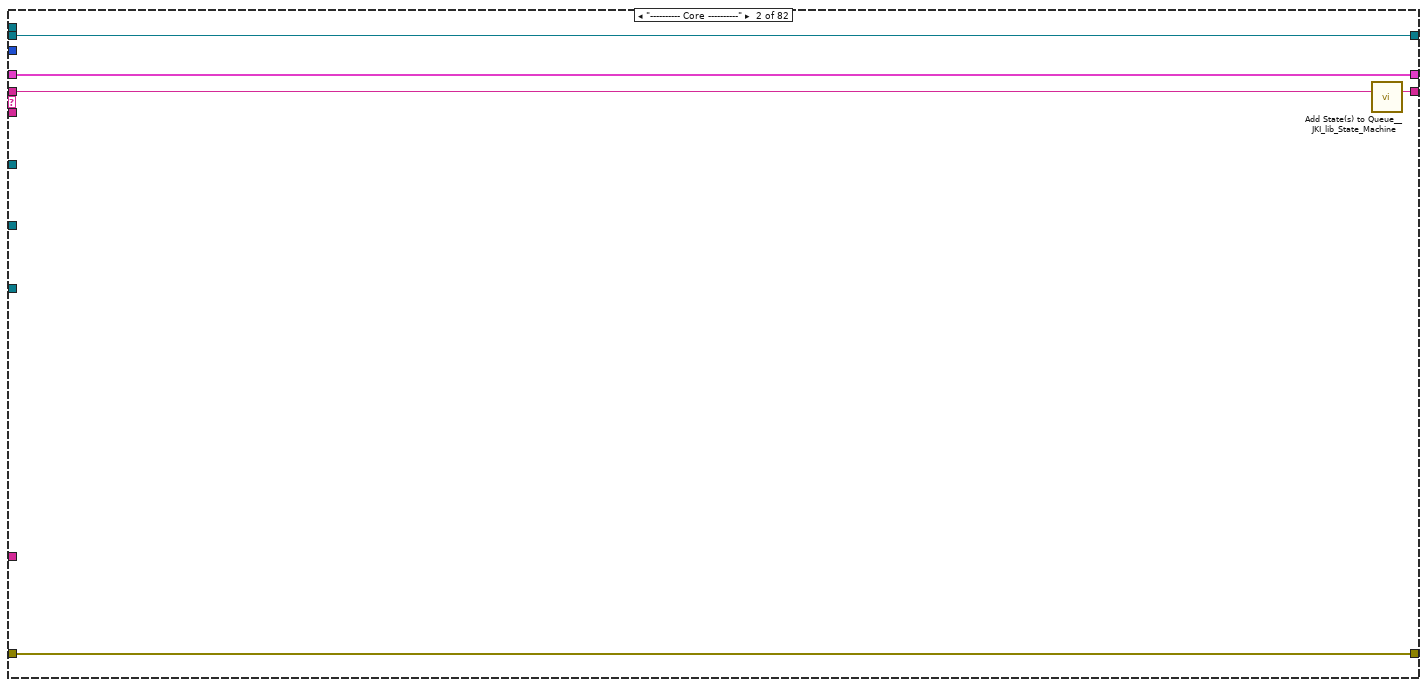
[diagram p19: hidden frame]
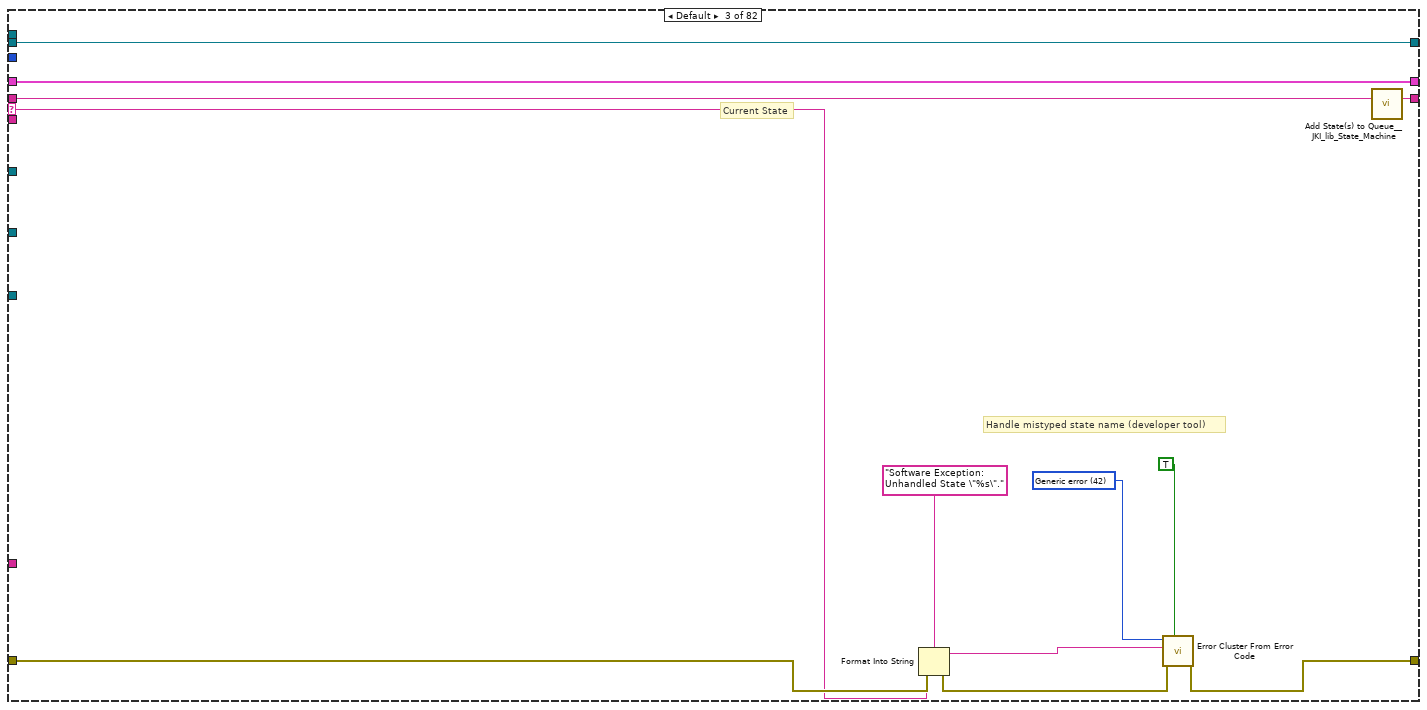
[diagram p20: hidden frame]
diagram:
  (unwired) "P,C,P,\"Print Manager,Print Line Manager,PMB-KM,PrintGoSource\",\"TTL\"\nP,C,P,\"Print Manager,Print Line Manager,PMB-KM,EncoderSource\",\"RS422\"\nP,P,1,C:\\Users\\labuser\\Desktop\\Scripts\\Patterns\\Print Weights\\PH1\\PW.bmp,5"
  (unwired) "Action: SendStatusPollEnable>>FALSE\nMacro: ExecutePrimingScan" ("State(s) in Front (\"\")")
  w3 = "Data: Initialize\nData: Read Config\nData: Read Config 2\nData: Read Init XML\nSystem: Start\nSystem: Launch Processes\nData: ReadPersistentData\nInitialize Core Data\nUI: Initialize\nEvents: Register Events\nSystem: Launch Main UI\nSystem: ReturnLaunchState >> Started\n/*UI: Front Panel State >> Open"  # Data: Initialize Data: Read Config Data: Read Config 2 Data: Read Init XML System: Start System: Launch Processes Data: ReadPersistentData Initialize Core Data UI: Initialize Events: Register Events System: Launch Main UI System: ReturnLaunchState >> Started /*UI: Front Panel State >> Open
  # "Action: Send Event>>CalPrintCount>>%d"
  # "MoveStage>>Load"
  # "Action: SendStatusPollEnable>>FALSE\nMacro: Execute Print"
  # "API: HeadPrint"
  # "API: Execute Printer Commands"
  # "Action: SendStatusPollEnable>>TRUE"
  # "Action: SendStatusPollEnable>>FALSE"
  n1 = call <vilib>:"Create NEW Queue with vData.vi"("Initial States"=cluster{"state":string, "vData":variant}[] [{"state"="Initialize", "vData"=variant}, {"state"="Idle", "vData"=variant}], "Name (SMQ)"="SMQ_Logger") -> ("error out"=w11:errorcluster, "queue out"=w12:refnum<queue>)  [unwired: 2 in]
  n2 = call <vilib>:"Add State(s) to Queue__JKI_lib_State_Machine.vi"("State(s) in (\"\")"="Macro: Initialize") -> ("States Out"=w17:string)  [unwired: 14 in]
  n3 = while "JKI - String-Based Queued State Machine (Basic) v1.0" {
    shift-right: [w28] -> w7
    shift-left: _ -> [w22]
    shift-right: [w31] -> w6
    shift-left: "error in" -> [w27]
    shift-right: [w30] -> _
    shift-left: w17 -> [w32]
    tunnel: "TopLevel in" -> [w26]
    shift-right: [w25] -> _
    shift-left: _ -> [w24]
    tunnel: w12 -> [w21]
    tunnel: "LaunchData" -> [w20]
    tunnel: w3 -> [w19]
    tunnel: "Str Refnum" -> [w18]
    stop <- w29 stop-if-true
    n4 = Unbundle By Name(w22) -> ("TO"=w23:i32)
    n5 = call <vilib>:"Parse State Queue__JKI_lib_State_Machine.vi"("State Queue"=w32, "Error In (no error)"=w27) -> ("Remaining States"=w34:string, "Current State"=w35:string, "Arguments"=w33:string)  [unwired: 11 in]
    n6 = case shown="\"System: Launch Processes\"" w35 {
      selector: w35 -> [_ _ w181 _ _ _ _ _ _ _ _ _ _ _ _ _ _ _ _ _ _ _ _ _ _ _ _ _ _ _ _ _ _ _ _ _ _ _ _ _ _ _ _ _ _ _ _ _ _ _ _ _ _ _ _ _ _ _ _ _ _ _ _ _ _ _ _ _ _ _ _ _ _ _ _ _ _ _ _ _ _ _]
      tunnel: w34 -> [w43 w179 w185 w204 w211 w217 w222 w247 w290 w303 w309 w334 w347 w359 w366 w371 w377 w384 w396 w423 w438 w460 w503 w520 _ w539 w543 w562 w565 w568 w582 w586 w606 w614 w633 w648 w666 w695 w710 w724 w739 w772 w833 w908 w985 w1062 w1139 w1216 w1260 w1338 w1416 w1494 w1572 w1650 w1718 w1730 w1752 w1773 w1811 w1823 w1837 w1845 w1862 w1907 w1936 w1961 w1972 w1994 w2032 w2068 w2101 w2116 w2127 w2134 w2143 w2151 w2155 w2165 w2180 w2195 w2217 w2231]
      tunnel: w33 -> [_ _ _ _ _ _ _ _ _ _ _ _ _ _ _ _ _ w379 w390 _ _ _ _ _ _ _ _ _ _ _ _ _ _ _ _ _ _ _ _ _ _ _ _ _ _ _ _ _ _ _ _ _ _ _ _ _ _ _ _ _ _ w1838 _ _ _ _ w1975 w1990 _ w2048 w2081 _ _ _ w2137 _ _ w2162 w2178 w2181 _ _]
      tunnel: w22 -> [w41 w176 w183 w195 w208 w215 w219 w244 _ w297 w306 w327 w341 w353 w361 w368 w375 w382 w392 w420 w435 w457 w500 w516 w523 w537 w541 w560 w564 w569 w580 w595 w611 w624 w639 w656 w664 w699 w714 w728 w743 w776 w827 w903 w979 w1055 w1133 w1210 w1253 w1330 w1409 w1488 w1566 w1644 w1719 w1728 w1750 w1770 w1808 w1822 w1835 w1841 w1851 w1891 w1934 w1960 w1968 w1992 w2019 w2057 w2090 w2115 w2125 w2131 w2140 w2148 w2154 w2160 w2173 w2193 w2202 w2230]
      tunnel: [w40 w177 w187 w201 errorcluster {"status"=FALSE, "code"=0, "source"=""} ("error out") w214 w220 w234 w268 w293 w304 w324 w339 w348 w362 w369 w372 w380 w393 w421 w425 w449 w479 w518 w525 w527 w542 w558 w566 w567 w571 w597 w601 w625 w640 w657 w662 w694 w709 w722 w731 w753 w825 w901 w978 w1058 w1131 w1209 w1255 w1333 w1412 w1487 w1565 w1643 w1717 w1724 w1747 w1778 w1801 w1824 w1832 w1846 w1852 w1878 w1926 w1962 w1978 w1989 w2020 w2058 w2091 w2117 w2121 w2132 w2141 w2149 w2156 w2158 w2175 w2182 w2204 w2226] -> w31
      tunnel: w27 -> [w39 w177 w186 w201 w207 w214 w220 w233 w268 w298 w307 w328 w338 w354 w363 w369 w373 w381 w394 w421 w424 w448 w479 w518 w525 w526 w542 w545 w566 w567 w579 w590 w610 w619 w637 w653 w663 w697 w712 w726 w741 w774 w831 w907 w983 w1061 w1138 w1215 w1259 w1336 w1415 w1493 w1571 w1649 w1717 w1723 w1746 w1777 w1807 w1824 w1826 w1846 w1852 w1895 w1913 w1962 w1978 w1988 w2012 w2052 w2085 w2117 w2120 w2135 w2144 w2152 w2156 w2157 w2174 w2190 w2203 w2225]
      tunnel: [w42 w178 w184 w203 w210 w216 w221 w246 w290 w303 w309 w334 w347 w359 w365 w370 w376 w383 w395 w422 w437 w459 w502 w519 w524 w538 w543 w561 w565 w568 w582 w587 w607 w615 w634 w649 w667 w696 w711 w725 w740 w773 w834 w909 w986 w1063 w1140 w1217 w1261 w1339 w1417 w1495 w1573 w1651 w1718 w1730 w1752 w1774 w1812 w1823 w1837 w1845 w1862 w1907 w1936 w1961 w1976 w1994 w2032 w2068 w2101 w2116 w2127 w2134 w2143 w2151 w2155 w2165 w2180 w2195 w2217 w2231] -> w30
      tunnel: [_ _ _ _ _ TRUE _ _ _ _ _ _ _ _ _ _ _ _ _ _ _ _ _ _ _ _ _ _ _ _ _ _ _ _ _ _ _ _ _ _ _ _ _ _ _ _ _ _ _ _ _ _ _ _ _ _ _ _ _ _ _ _ _ _ _ _ _ _ _ _ _ _ _ _ _ _ _ _ _ _ _ _] -> w29
      tunnel: [w38 w176 w183 w202 w208 w215 w219 w232 w289 w295 w305 w326 w337 w356 w361 w368 w375 w382 w392 w420 w432 w455 w499 w515 w523 w537 w541 w555 w564 w569 w580 w600 w612 w628 w643 w660 w665 w693 w708 w721 w737 w771 w828 w904 w980 w1056 w1134 w1211 w1254 w1331 w1410 w1489 w1567 w1645 w1719 w1728 w1750 w1771 w1806 w1822 w1835 w1841 w1851 w1904 w1934 w1960 w1968 w1992 w2019 w2057 w2090 w2115 w2125 w2131 w2140 w2148 w2154 w2160 w2173 w2193 w2202 w2230] -> w28
      tunnel: w23 -> [w37 _ _ _ _ _ _ _ _ _ _ _ _ _ _ _ _ _ _ _ _ _ _ _ _ _ _ _ _ _ _ _ _ _ _ _ _ _ _ _ _ _ _ _ _ _ _ _ _ _ _ _ _ _ _ _ _ _ _ _ _ _ _ _ _ _ _ _ _ _ _ _ _ _ _ _ _ _ _ _ _ _]
      tunnel: w26 -> [_ _ _ _ _ _ _ _ w274 _ _ _ _ _ _ _ _ _ _ _ _ _ _ _ _ _ _ _ _ _ _ _ _ _ _ _ _ _ _ _ _ _ _ _ _ _ _ _ _ _ _ _ _ _ _ _ _ _ _ _ _ _ _ _ _ _ _ _ _ _ _ _ _ _ _ _ _ _ _ _ _ _]
      tunnel: [w36 w175 w180 w192 w205 w212 w218 w245 w287 w302 w308 w333 w346 w358 w360 w367 w374 w378 w389 w419 w436 w458 w501 w517 w522 w530 w540 w550 w563 w570 w583 w585 w605 w629 w644 w661 w669 w700 w715 w729 w744 w777 w835 w910 w987 w1064 w1141 w1218 w1262 w1340 w1418 w1496 w1574 w1652 w1720 w1729 w1751 w1781 w1813 w1821 w1836 w1844 w1861 w1906 w1935 w1959 w1977 w1993 w2031 w2067 w2100 w2114 w2126 w2133 w2142 w2150 w2153 w2164 w2179 w2194 w2216 w2229] -> w25
      tunnel: w24 -> [w36 w175 w180 w192 w205 w212 w218 w245 w287 w302 w308 w333 w346 w358 w360 w367 w374 w378 w389 w419 w436 w458 w501 w517 w522 w530 w540 _ w563 w570 w583 w585 w605 w629 w644 w661 w669 w700 w715 w729 w744 w777 w835 w910 w987 w1064 w1141 w1218 w1262 w1340 w1418 w1496 w1574 w1652 w1720 w1729 w1751 w1781 w1813 w1821 w1836 w1844 w1861 w1906 w1935 w1959 w1977 w1993 w2031 w2067 w2100 w2114 w2126 w2133 w2142 w2150 w2153 w2164 w2179 w2194 w2216 w2229]
      tunnel: w21 -> [_ _ _ _ _ _ _ _ _ _ _ _ _ _ _ _ _ _ _ _ _ _ _ _ _ w529 _ _ _ _ _ _ _ _ _ _ _ _ _ _ _ _ _ _ _ _ _ _ _ _ _ _ _ _ _ _ _ _ _ _ _ _ _ _ _ _ _ _ _ _ _ _ _ _ _ _ _ _ _ _ _ w2228]
      tunnel: w20 -> [_ _ _ _ _ _ _ _ w255 _ _ _ _ _ _ _ _ _ _ _ _ _ _ _ _ _ _ _ _ _ _ _ _ _ _ _ _ _ _ _ _ _ _ _ _ _ _ _ _ _ _ _ _ _ _ _ _ _ _ _ _ _ _ _ _ _ _ _ _ _ _ _ _ _ _ _ _ _ _ _ _ _]
      tunnel: w19 -> [_ _ _ _ _ _ _ _ _ _ _ _ _ _ _ _ _ _ _ _ _ _ _ _ w521 _ _ _ _ _ _ _ _ _ _ _ _ _ _ _ _ _ _ _ _ _ _ _ _ _ _ _ _ _ _ _ _ _ _ _ _ _ _ _ _ _ _ _ _ _ _ _ _ _ _ _ _ _ _ _ _ _]
      tunnel: w18 -> [_ _ _ _ _ _ _ _ w248 _ _ _ _ _ _ _ _ _ _ _ _ _ _ _ _ _ _ _ _ _ _ _ _ _ _ _ _ _ _ _ _ _ _ _ _ _ _ _ _ _ _ _ _ _ _ _ _ _ _ _ _ _ _ _ _ _ _ _ _ _ _ _ _ _ _ _ _ _ _ _ _ _]
      frame "", "Event Structure", "Idle" {
        n7 = event shown="[5] <API Incoming Event>: User Event" {
          selector: w36 -> [_ _ _ _ _ _ _]
          dyn-events: _ -> [_ _ _ _ _ _ _]
          timeout: w37 -> [_ _ _ _ _ _ _]
          tunnel: w43 -> [w54 w58 w62 w67 w71 w74 w158]
          tunnel: [w53 w57 w61 w66 w70 w83 w159] -> w42
          tunnel: w41 -> [w51 w55 w59 w64 w68 w86 w157]
          tunnel: [w52 w56 w60 w65 w69 w84 w151] -> w40
          tunnel: w39 -> [w52 w56 w60 w65 w69 w75 w152]
          tunnel: [w51 w55 w59 w64 w68 w87 w154] -> w38
          event Timeout {
            n8 = event-data() -> ()  [unwired: 1 in, 1 out]
            n9 = Unbundle By Name(w51) -> ("Tasks"=w50:T15[], "Idle Mode"=w44:bool)
            n10 = Empty Array?(array=w50) -> (empty?=w49:bool)
            n11 = Or(x=w49, y=w44) -> (x .or. y?=w45:bool)
            n12 = Select(t="", s=w45, f="Task: Check Timeout") -> (s? t:f=w46:string)
            n13 = call <vilib>:"Add State(s) to Queue__JKI_lib_State_Machine.vi"("State(s) in Front (\"\")"=w46, "State(s) in (\"\")"=w54) -> ("States Out"=w53:string)  [unwired: 13 in]
          }
          event User Event {
            n14 = event-data() -> ()  [unwired: 1 in, 6 out]
            n15 = call <vilib>:"Add State(s) to Queue__JKI_lib_State_Machine.vi"("State(s) in (\"\")"=w58) -> ("States Out"=w57:string)  [unwired: 14 in]
          }
          event User Event {
            n16 = event-data() -> ()  [unwired: 1 in, 7 out]
            n17 = Unbundle By Name(w59) -> ()  [unwired: 1 out]
            n18 = call <vilib>:"Add State(s) to Queue__JKI_lib_State_Machine.vi"("State(s) in (\"\")"=w62) -> ("States Out"=w61:string)  [unwired: 14 in]
          }
          event "OK": Value Change; User Event {
            # "Exit Button Value Change (pressed) Event\n(this executes Macro: Exit to terminate the VI)"
            n19 = event-data() -> ()  [unwired: 1 in, 3 out]
            n20 = call <vilib>:"Add State(s) to Queue__JKI_lib_State_Machine.vi"("State(s) in Front (\"\")"="Macro: Exit", "State(s) in (\"\")"=w67) -> ("States Out"=w66:string)  [unwired: 13 in]
          }
          event Panel Close? {
            # "Close Panel button (pressed) Event\n(this executes Macro: Exit to terminate the VI)"
            n21 = event-data() -> ()  [unwired: 1 in, 1 out]
            n22 = event-data() -> ()  [unwired: 2 in, 1 out]
            n23 = call <vilib>:"Add State(s) to Queue__JKI_lib_State_Machine.vi"("State(s) in (\"\")"=w71) -> ("States Out"=w70:string)  [unwired: 14 in]
          }
          event User Event {
            n24 = event-data() -> ("Task"=w90:T59, "Command"=w79:variant)  [unwired: 1 in, 4 out]
            n25 = Unbundle By Name(w86) -> ("Tasks"=w88:T15[], "TopLevel in"=w72:refnum<class "TopLevel.lvclass">)
            n26 = Bundle By Name(cluster=T15 {"Task"={"Time Stamp"=timestamp(0 s since 1904-01-01), "Timeout (ms)"=0, "Task State"=enum."Completed", "Task Error"={"status"=FALSE, "code"=0, "source"=""}, "Task ID"=""}, "Command"=variant, "Return Value"=variant} ("API Event Data"), "Task"=w90, "Command"=w79) -> (w85:T15)
            n27 = Variant To Data(error in=w75, type=T13 {"Command"=enum."Execute Printer Commands", "Arguments"="", "Data"=variant} ("API Command Cluster"), Variant=w79) -> (data=w81:T13, error out=w76:errorcluster)
            n28 = Unbundle By Name(w81) -> ("Command"=w78:T14, "Arguments"=w77:string)
            n29 = Empty Array?(array=w88) -> (empty?=w89:bool)
            n30 = case shown="Default" w78 {
              tunnel: w89 -> [_ _ w111]
              tunnel: w88 -> [_ _ w110]
              tunnel: [w94 w99 w109] -> w87
              tunnel: w86 -> [w95 w100 w108]
              tunnel: w85 -> [_ _ w107]
              tunnel: [w93 w98 w106] -> w84
              tunnel: w76 -> [w93 w98 w105]
              tunnel: [_ "Task: Remove on Error" w104] -> w82
              tunnel: w77 -> [_ _ _]
              tunnel: w74 -> [_ _ w103]
              tunnel: ["Macro: Execute Idle Print" ("Remaining States") _ w103] -> w73
              tunnel: w72 -> [_ _ w102]
              frame "StopIdlePrintCycle" {
                n31 = Bundle By Name(cluster=w95, "Idle Mode"=FALSE) -> (w94:T61)
              }
              frame "Abort" {
                n32 = Bundle By Name(cluster=w100, "Idle Mode"=FALSE) -> (w99:T61)
              }
              frame Default {
                n33 = case shown="True" w111 {
                  tunnel: w110 -> [w132 w138]
                  tunnel: w107 -> [w131 w137]
                  tunnel: w108 -> [w130 w136]
                  tunnel: [w129 w134] -> w109
                  tunnel: w107 -> [w128 _]
                  tunnel: w105 -> [w113 w133]
                  tunnel: [w124 w133] -> w106
                  tunnel: [w122 _] -> w104
                  tunnel: w102 -> [w115 _]
                  frame True {
                    (unwired) API_Command_Enum."Execute Printer Commands" ("Command")
                    n34 = Unbundle By Name(w128) -> ("Command"=w127:variant)
                    n35 = call-dynamic "SetTopLevel Busy_StatusChangedEvent.vi"("error in (no error)"=w113, "Status.Busy"=TRUE, "TopLevel in"=w115) -> ("error out"=w114:errorcluster)  [unwired: 7 in, 1 out]
                    n36 = Build Array (concatenate)(w132, w131) -> (w119:T15[])
                    n37 = Variant To Data(error in=w114, type=T13 {"Command"=enum."Execute Printer Commands", "Arguments"="", "Data"=variant} ("API Command Cluster"), Variant=w127) -> (data=w120:T13, error out=w125:errorcluster)
                    n38 = Unbundle By Name(w120) -> ("Command"=w123:T14, "Arguments"=w121:string)
                    n39 = Tick Count (ms)() -> (millisecond timer value=w117:u32)
                    n40 = Format Into String(format string="API: %s>>%s", error in=w125, w123, w121) -> (resulting string=w122:string, error out=w124:errorcluster)  [unwired: 1 in]
                    n41 = Bundle By Name(cluster=w130, "TO"=100, "Tasks"=w119, "Task Start ms"=w117, "Current Task"=w120) -> (w129:T61)
                  }
                  frame False {
                    n42 = Build Array (concatenate)(w138, w137) -> (w135:T15[])
                    n43 = Bundle By Name(cluster=w136, "Tasks"=w135) -> (w134:T61)
                  }
                }
              }
            }
            n44 = call <vilib>:"Add State(s) to Queue__JKI_lib_State_Machine.vi"("State(s) in Front (\"\")"=w82, "State(s) in (\"\")"=w73) -> ("States Out"=w83:string)  [unwired: 13 in]
          }
          event User Event {
            n45 = event-data() -> ("Task"=w145:T59, "Command"=w149:variant, "Return Value"=w148:variant)  [unwired: 1 in, 4 out]
            n46 = Unbundle By Name(w157) -> ("API Return Event"=w142:refnum<user-event>, "Tasks"=w156:T15[])
            n47 = Bundle By Name(cluster=T15 {"Task"={"Time Stamp"=timestamp(0 s since 1904-01-01), "Timeout (ms)"=0, "Task State"=enum."Completed", "Task Error"={"status"=FALSE, "code"=0, "source"=""}, "Task ID"=""}, "Command"=variant, "Return Value"=variant} ("API Event Data"), "Task"=w145, "Command"=w149, "Return Value"=w148) -> (w147:T15)
            n48 = Delete From Array(array=w156, index=0) -> (deleted portion=w146:T15, array with subset deleted=w153:T15[])  [unwired: 1 in]
            n49 = Unbundle By Name(w146) -> ("Task.Task ID"=w144:string)
            n50 = Unbundle By Name(w145) -> ("Task ID"=w143:string, "Task State"=w140:T16)
            n51 = Equal?(x=w144, y=w143) -> (x = y?=w141:bool)
            n52 = case shown="True" w141 {
              tunnel: w157 -> [w161 w174]
              tunnel: [w161 w173] -> w154
              tunnel: w153 -> [_ w172]
              tunnel: w142 -> [_ w171]
              tunnel: w152 -> [w160 w168]
              tunnel: [w160 w169] -> w151
              tunnel: w147 -> [_ w170]
              tunnel: w140 -> [_ w167]
              tunnel: [_ w162] -> w139
              frame False {
              }
              frame True {
                n53 = Equal?(x=w167, y=API_Task_State."Errored") -> (x = y?=w165:bool)
                n54 = Select(t="Task: Remove on Error", s=w165, f="Task: Check Pending") -> (s? t:f=w162:string)
                n55 = Bundle By Name(cluster=w174, "Tasks"=w172) -> (w173:T61)
                n56 = Generate User Event(user event=w171, event data cluster=w170, error in=w168) -> (error out=w169:errorcluster)  [unwired: 1 in, 1 out]
              }
            }
            n57 = call <vilib>:"Add State(s) to Queue__JKI_lib_State_Machine.vi"("State(s) in Front (\"\")"=w139, "State(s) in (\"\")"=w158) -> ("States Out"=w159:string)  [unwired: 13 in]
          }
        }
      }
      frame "---------- Core ----------" {
        n58 = call <vilib>:"Add State(s) to Queue__JKI_lib_State_Machine.vi"("State(s) in (\"\")"=w179) -> ("States Out"=w178:string)  [unwired: 14 in]
      }
      frame Default {
        w190 = 42 items=["No error", "Argument error", "Memory is full", "Out of zone", "End of file", "File already open", "Generic file I/O error", "File not found", "File permission error", "Disk is full", "Duplicate path", "Too many files open", "System feature not enabled", "Resource file not found", "Cannot add resource", "Resource not found", "Image not found", "Image memory error", "Pen does not exist", "Config type invalid", "Config token not found", "Config parse error", "Config memory error", "Bad external code format", "Bad external code offset", "External code not present", "Null window", "Destroy window error", "Null menu", "Print aborted", "Bad print record", "Print driver error", "Windows error during printing", "Memory error during printing", "Print dialog error", "Generic print error", "Invalid device refnum", "Device not found", "Device parameter error", "Device unit error", "Cannot open device", "Device call aborted", "Generic error", "Cancelled by user", "Object ID too low", "Object ID too high", "Object not in heap", "Unknown heap", "Unknown object (invalid DefProc)", "Unknown object (DefProc not in table)", "Message out of range", "Invalid (null) method", "Unknown message", "Manager call not supported", "Bad address", "Network operation in progress", "Network operation timed out", "Connection is busy", "Network attribute not supported", "Network error", "Address in use", "System out of memory", "Connection aborted", "Connection refused", "Not connected", "Already connected", "Connection closed", "Initialization error (interapplication manager)", "Bad occurrence", "Wait on unbound occurrence handler", "Occurrence queue overflow", "Datalog type conflict", "Unused", "Unrecognized type (interapplication manager)", "Memory corrupt", "Failed to make temporary DLL", "Old CIN version", "Drag socket not found", "Failed to load drop-object", "Failed to register OLE object", "Failed to release OLE object", "Format specifier type mismatch", "Unknown format specifier", "Too few format specifiers", "Too many format specifiers", "Scan failed", "Newer CIN version", "Error converting to variant", "Runtime menu error", "Password tampered", "Variant attribute not found", "Incompatible variant data type", "Event data is not available", "Event Store is not present", "Occurrence is not found", "Event Queue is not created", "Event info is not available", "Refnum passed is NULL", "Error retrieving Class GUID", "Error retrieving CoClass GUID", "Error retrieving TypeLib GUID.", "Bad built application magic bytes.", "Specific driver is different from the specific driver associated with the Logical Name.", "There is no session opened to the class driver.", "Max Error", "MAX - Error with config objects", "MAX - Error loading configuration", "MAX - Group not supported"]
        # "Current State"
        # "Handle mistyped state name (developer tool)"
        n59 = Format Into String(format string="Software Exception: Unhandled State \"%s\"." ("message"), error in=w186, w181) -> (resulting string=w189:string, error out=w188:errorcluster)  [unwired: 1 in]
        n60 = call <vilib>:"Error Cluster From Error Code.vi"("show call chain? (False)"=TRUE, "error in (no error)"=w188, "error message (\"\")"=w189, "error code (0)"=w190) -> ("error out"=w187:errorcluster)  [unwired: 5 in]
        n61 = call <vilib>:"Add State(s) to Queue__JKI_lib_State_Machine.vi"("State(s) in (\"\")"=w185) -> ("States Out"=w184:string)  [unwired: 14 in]
      }
      frame "Initialize Core Data" {
        # "originally closed?"
        # "exe?"
        # "If panel starts closed or is an EXE, then close it when we exit"
        n62 = property class="VI"() -> ("Front Panel.Open"=w200:bool)  [unwired: 2 in, 2 out]
        n63 = property class="App"() -> ("App.Kind"=w199:T17)  [unwired: 2 in, 2 out]
        n64 = control-ref of="Current VI Reference"() -> (w193:refnum<vi>)
        n65 = Not(x=w200) -> (.not. x?=w197:bool)
        n66 = Equal?(x=w199, y=T17."Run Time System" ("Application:Kind")) -> (x = y?=w196:bool)
        n67 = Or(x=w197, y=w196) -> (x .or. y?=w194:bool)
        n68 = Bundle By Name(cluster=w195, "Core.Current VI Reference"=w193, "Core.Close Panel on Exit?"=w194) -> (w202:T61)
        n69 = call <vilib>:"Add State(s) to Queue__JKI_lib_State_Machine.vi"("State(s) in (\"\")"=w204) -> ("States Out"=w203:string)  [unwired: 14 in]
      }
      frame "Error Handler" {
        # "#TODO handle errors"
        # "Unhandled Error -- Display it"
        # "Clear error"
        n70 = call <vilib>:"General Error Handler.vi"("error in (no error)"=w207) -> ()  [unwired: 10 in, 5 out]
        n71 = call <vilib>:"Add State(s) to Queue__JKI_lib_State_Machine.vi"("State(s) in Front (\"\")"="/* Post Error States", "State(s) in (\"\")"=w211) -> ("States Out"=w210:string)  [unwired: 13 in]
      }
      frame "Exit" {
        n72 = call <vilib>:"Add State(s) to Queue__JKI_lib_State_Machine.vi"("State(s) in (\"\")"=w217) -> ("States Out"=w216:string)  [unwired: 14 in]
      }
      frame "---------- Data ----------" {
        n73 = call <vilib>:"Add State(s) to Queue__JKI_lib_State_Machine.vi"("State(s) in (\"\")"=w222) -> ("States Out"=w221:string)  [unwired: 14 in]
      }
      frame "Data: ReadStartup" {
        n74 = Unbundle By Name(w244) -> ("StartupPath"=w243:path)
        n75 = call <vilib>:"Open Config Data.vi"("error in (no error)"=w233, "configuration file path"=w243) -> ("error out"=w235:errorcluster, "refnum"=w242:T62)  [unwired: 7 in, 1 out]
        n76 = call-poly <vilib>:"Read Key.vi"("section"="General", "error in (no error)"=w235, "key"="MasterConfiguration", "refnum"=w242) -> ("error out"=w236:errorcluster, "value"=w231:path, "refnum out"=w237:T62)  [unwired: 4 in, 1 out]
        n77 = call-poly <vilib>:"Read Key.vi"("section"="General", "error in (no error)"=w236, "key"="DLP2Config", "refnum"=w237) -> ("error out"=w225:errorcluster, "value"=w230:path, "refnum out"=w227:T62)  [unwired: 4 in, 1 out]
        n78 = call-poly <vilib>:"Read Key.vi"("section"="General", "error in (no error)"=w225, "key"="DAQConfig", "refnum"=w227) -> ("error out"=w224:errorcluster, "value"=w223:path, "refnum out"=w226:T62)  [unwired: 4 in, 1 out]
        n79 = Bundle By Name(cluster=w244, "Digilens Config File Path"=w231, "DLP2 ConfigPath"=w230, "DAQConfigPath"=w223) -> (w232:T61)
        n80 = call <vilib>:"Close Config Data.vi"("error in (no error)"=w224, "refnum"=w226) -> ("error out"=w234:errorcluster)  [unwired: 8 in, 1 out]
        n81 = call <vilib>:"Add State(s) to Queue__JKI_lib_State_Machine.vi"("State(s) in (\"\")"=w247) -> ("States Out"=w246:string)  [unwired: 14 in]
      }
      frame "Data: Initialize" {
        w250 = string[] []  # GIS Commands
        w251 = T60 {"TotalRepeats"=0, "CurrentScan"=0}  # PMScanTrk
        w252 = refnum<class "DAQ.lvclass"> refnum  # DAQ
        w254 = path ""  # DAQConfigPath
        w256 = T8 {"Interval (s)"=0.1, "PurgeDuration (s)"=0.1, "Repeats"=0, "PrimingMode"=enum."Pre-Purge", "Head"=enum."1", "Frequency (Hz)"=0, "PrintWeight"=0.1}  # PrinterModeAPI Data
        w257 = path ""  # DLP2 ConfigPath
        w258 = path ""  # Digilens Config File Path
        w262 = refnum<class "DLP2.lvclass"> refnum  # DLP2
        w263 = refnum<class "Database.lvclass"> refnum  # Database
        w264 = FALSE  # HomeOnComplete
        w267 = FALSE  # Idle Mode
        w269 = 0.0  # IdleTimer
        w270 = T60 {"TotalRepeats"=0, "CurrentScan"=0}  # PrintScanTrk
        w271 = T60 {"TotalRepeats"=0, "CurrentScan"=0}  # PPScanTrk
        w273 = path ""  # Printer Command File Path
        w265 = refnum<class "Motor Controller.lvclass"> refnum  # Motor Controller
        w266 = refnum<class "GIS Printer.lvclass"> refnum  # GIS Printer
        w261 = refnum<class "IO.lvclass"> refnum  # IO
        w275 = T13 {"Command"=enum."Execute Printer Commands", "Arguments"="", "Data"=variant}  # Current Task
        w276 = T38 {"Motion Controller"={"Motor IP Addresss"="", "Current Position"=0, "Pulse_Per_mm"=0, "PrePrint"=[], "Load Position_mm"=0, "Laminate Position_mm"=0}, "IO Config"={"DAQDevices"=[], "DI Channels"=[], "DO Channels"=[], "Material Names"=[], "AI Channels"=[], "AO Channels"=[]}, "PrinterConfiguration"={"IPAddress"="", "Move Stage on RTP Command?"=FALSE, "Stage Move Position"="", "PH1-Prime Path"=path "", "PH2-Prime Path"=path "", "PH3-Prime Path"=path "", "PH4-Prime Path"=path "", "PH5-Prime Path"=path "", "PH6-Prime Path"=path "", "PrintScriptsFolder"=path "", "PurgeScriptsFolder"=path "", "StageScriptsFolder"=path "", "PH1-HeatOn Path"=path "", "PH2-HeatOn Path"=path "", "PH3-HeatOn Path"=path "", "PH4-HeatOn Path"=path "", "PH5-HeatOn Path"=path "", "PH6-HeatOn Path"=path "", "PH1-HeatOff Path"=path "", "PH2-HeatOff Path"=path "", "PH3-HeatOff Path"=path "", "PH4-HeatOff Path"=path "", "PH5-HeatOff Path"=path "", "PH6-HeatOff Path"=path ""}, "DAQ Settings"={"Simulate DAQ"=FALSE, "DI Settings"=[], "AI Settings"=[], "Relay IONames"=[], "AO IONames"=[], "AO NChan SingleTask"=FALSE}}  # Digilens IPLC Config
        w278 = path ""  # StartupPath
        w281 = variant  # Current Task. Return Value
        w282 = refnum<user-event> refnum  # API Return Event
        w283 = refnum<user-event> refnum  # API Executed Event
        w284 = u32 0  # Task Start ms
        w285 = -1  # TO
        w286 = T15[] []  # Tasks
        w288 = T63 {"Current VI Reference"=refnum, "Close Panel on Exit?"=FALSE}  # Core
        n82 = call <vilib>:"Application Directory.vi"() -> ("Application Directory"=w259:path)
        n83 = Build Path(base path=w259, name or relative path="Startup.ini") -> (appended path=w279:path)
        n84 = Coerce To Type(0:w279, 1:w278) -> (2:w277:path)
        n85 = Bundle("Core"=w288, "TopLevel in"=w274, "Tasks"=w286, "TO"=w285, "API Executed Event"=w283, "API Return Event"=w282, "Task Start ms"=w284, "Current Task. Return Value"=w281, "StartupPath"=w277, "Digilens IPLC Config"=w276, "Current Task"=w275, "IO"=w261, "GIS Printer"=w266, "Motor Controller"=w265, "Printer Command File Path"=w273, "Pre Purge API Data"=T36 {"Purge Channel Name"=enum."Purge Valve Open - R1", "GIS File Path"=path "", "Duration (s)"=0.1, "PurgeDuration (s)"=0.1, "Repeats"=0}, "PPScanTrk"=w271, "PrintScanTrk"=w270, "IdleTimer"=w269, "Idle Mode"=w267, "HomeOnComplete"=w264, "Database"=w263, "DLP2"=w262, "MasterConfigurationDLPC2"=T3 {"Paths"={"DigiBit WG Design Folder"=path "", "Compensated GS Image Folder"=path "", "Nozzle GS Files Head 1"=path "", "Nozzle GS Files Head 2"=path "", "Nozzle GS Files Head 3"=path "", "Nozzle GS Files Head 4"=path "", "Nozzle GS Files Head 5"=path "", "Nozzle GS Files Head 6"=path ""}, "ColorPaneMapping"={"Head 1"={"Material"="", "ColorPane"=""}, "Head 2"={"Material"="", "ColorPane"=""}, "Head 3"={"Material"="", "ColorPane"=""}, "Head 4"={"Material"="", "ColorPane"=""}, "Head 5"={"Material"="", "ColorPane"=""}, "Head 6"={"Material"="", "ColorPane"=""}}, "Materials"=[], "ColorPlanes"=[], "SpitVoltages_Half"={"1"=0.0, "2"=0.0, "3"=0.0, "4"=0.0, "5"=0.0, "6"=0.0}, "SpitVoltages_Full"={"1"=0.0, "2"=0.0, "3"=0.0, "4"=0.0, "5"=0.0, "6"=0.0}, "SystemMode"=[], "PrimeModeConfig"=[], "Running Average Duration_s"=5.0}, "Digilens Config File Path"=w258, "DLP2 ConfigPath"=w257, "GIS Commands"=w250, "PrinterModeAPI Data"=w256, "LaunchData"=w255, "DAQConfigPath"=w254, "IO Nodes"=T22 {"DI Config"={"DI Tasks"=[]}, "DO Config"={"DO Channels"=[]}, "AI Config"={"AI Tasks"=[]}, "AO Config"={"AO Channels"=[]}}, "DAQ"=w252, "PMScanTrk"=w251, "DLP"=T18 {"PrinterInitialization"={"Printer"={"#attributes"={"Name"=""}}, "VacPumpSet"={"#attributes"={"VacPumpEnable"=FALSE, "VacPumpSpeed"=0.0}}, "HIBEnable"={"#attributes"={"HIB1Enable"=FALSE, "HIB2Enable"=FALSE, "HIB3Enable"=FALSE, "HIB4Enable"=FALSE, "HIB5Enable"=FALSE, "HIB6Enable"=FALSE}}, "PrinterCompensation"={"#attributes"={"AppName"="", "PrintWeightMultiplier"=0.0, "Rotation"=FALSE, "Driver"="", "Server"="", "Database"="", "User"="", "Password"=""}}}, "HeadSet"={"HeadProperties"=[]}, "InkSet"={"Ink"=[]}, "Troubleshooting"={"PMBLogging"={"#attributes"={"PMBMonitorDuringPrint"=FALSE, "PMBMonitorDuringIdle"=FALSE, "LogSwatheInputData"=FALSE, "LogSwatheOutputData"=FALSE, "LogPrintheadColourPlanes"=FALSE, "LogPMBCommunication"=FALSE, "LogSimulatedOutput"=FALSE, "LogAllPMBCommunicationData"=FALSE, "LogPMBSpace"=FALSE, "ExtendedPMBSpaceLogging"=FALSE, "LogPMBWriteSpeed"=FALSE, "LogUsbRetries"=FALSE}}, "HIBLogging"={"#attributes"={"HIBMonitoringDuringPrint"=FALSE, "HIBMonitoringLog"=FALSE}}}}, "Str Refnum"=w248) -> (w289:T61)  [unwired: 1 in]
      }
      frame "Data: Read Config" {
        n86 = call "FG - FilePathnames.vi"() -> ("FilePaths out"=w292:T64)  [unwired: 4 in, 1 out]
        n87 = Unbundle By Name(w297) -> ("Digilens IPLC Config"=w301:T38)
        n88 = Unbundle By Name(w292) -> ("Config SettingsFile"=w291:path)
        n89 = call <vilib>:"Easy Read XML File__JKI EasyXML.vi"("error in (no error)"=w298, "LabVIEW Data (Type)"=w301, "XML File Path"=w291) -> ("error out"=w299:errorcluster, "LabVIEW Data"=w300:variant)  [unwired: 6 in, 1 out]
        n90 = Variant To Data(error in=w299, type=T38 {"Motion Controller"={"Motor IP Addresss"="", "Current Position"=0, "Pulse_Per_mm"=0, "PrePrint"=[], "Load Position_mm"=0, "Laminate Position_mm"=0}, "IO Config"={"DAQDevices"=[], "DI Channels"=[], "DO Channels"=[], "Material Names"=[], "AI Channels"=[], "AO Channels"=[]}, "PrinterConfiguration"={"IPAddress"="", "Move Stage on RTP Command?"=FALSE, "Stage Move Position"="", "PH1-Prime Path"=path "", "PH2-Prime Path"=path "", "PH3-Prime Path"=path "", "PH4-Prime Path"=path "", "PH5-Prime Path"=path "", "PH6-Prime Path"=path "", "PrintScriptsFolder"=path "", "PurgeScriptsFolder"=path "", "StageScriptsFolder"=path "", "PH1-HeatOn Path"=path "", "PH2-HeatOn Path"=path "", "PH3-HeatOn Path"=path "", "PH4-HeatOn Path"=path "", "PH5-HeatOn Path"=path "", "PH6-HeatOn Path"=path "", "PH1-HeatOff Path"=path "", "PH2-HeatOff Path"=path "", "PH3-HeatOff Path"=path "", "PH4-HeatOff Path"=path "", "PH5-HeatOff Path"=path "", "PH6-HeatOff Path"=path ""}, "DAQ Settings"={"Simulate DAQ"=FALSE, "DI Settings"=[], "AI Settings"=[], "Relay IONames"=[], "AO IONames"=[], "AO NChan SingleTask"=FALSE}} ("Digilens IPLC Config"), Variant=w300) -> (data=w294:T38, error out=w293:errorcluster)
        n91 = Bundle By Name(cluster=w297, "Digilens IPLC Config"=w294) -> (w295:T61)
      }
      frame "Data: Read Config 2" {
        n92 = disable-structure shown="Enabled" {
          disable-tunnel: w307 -> [w317 w321]
          disable-tunnel: w306 -> [w316 w322]
          disable-tunnel: [w315 w322] -> w305
          disable-tunnel: [w310 w321] -> w304
          frame Enabled {
            n93 = Unbundle By Name(w316) -> ("MasterConfigurationDLPC2"=w320:T3)
            n94 = call "FG - FilePathnames.vi"() -> ("FilePaths out"=w313:T64)  [unwired: 4 in, 1 out]
            n95 = Unbundle By Name(w313) -> ("DLPUIConfigFile"=w312:path)
            n96 = call <vilib>:"Easy Read XML File__JKI EasyXML.vi"("error in (no error)"=w317, "LabVIEW Data (Type)"=w320, "XML File Path"=w312) -> ("error out"=w318:errorcluster, "LabVIEW Data"=w319:variant)  [unwired: 6 in, 1 out]
            n97 = Variant To Data(error in=w318, type=T3 {"Paths"={"DigiBit WG Design Folder"=path "", "Compensated GS Image Folder"=path "", "Nozzle GS Files Head 1"=path "", "Nozzle GS Files Head 2"=path "", "Nozzle GS Files Head 3"=path "", "Nozzle GS Files Head 4"=path "", "Nozzle GS Files Head 5"=path "", "Nozzle GS Files Head 6"=path ""}, "ColorPaneMapping"={"Head 1"={"Material"="", "ColorPane"=""}, "Head 2"={"Material"="", "ColorPane"=""}, "Head 3"={"Material"="", "ColorPane"=""}, "Head 4"={"Material"="", "ColorPane"=""}, "Head 5"={"Material"="", "ColorPane"=""}, "Head 6"={"Material"="", "ColorPane"=""}}, "Materials"=[], "ColorPlanes"=[], "SpitVoltages_Half"={"1"=0.0, "2"=0.0, "3"=0.0, "4"=0.0, "5"=0.0, "6"=0.0}, "SpitVoltages_Full"={"1"=0.0, "2"=0.0, "3"=0.0, "4"=0.0, "5"=0.0, "6"=0.0}, "SystemMode"=[], "PrimeModeConfig"=[], "Running Average Duration_s"=5.0} ("MasterConfigurationDLPC2"), Variant=w319) -> (data=w311:T3, error out=w310:errorcluster)
            "data" <- w311
            n98 = Bundle By Name(cluster=w316, "MasterConfigurationDLPC2"=w311) -> (w315:T61)
          }
          frame Disabled {
          }
        }
      }
      frame "Data: Read DAQ Config" {
        n99 = Unbundle By Name(w327) -> ("DAQConfigPath"=w332:path, "IO Nodes"=w331:T22)
        n100 = call <vilib>:"Easy Read XML File__JKI EasyXML.vi"("error in (no error)"=w328, "LabVIEW Data (Type)"=w331, "XML File Path"=w332) -> ("error out"=w329:errorcluster, "LabVIEW Data"=w330:variant)  [unwired: 6 in, 1 out]
        n101 = Variant To Data(error in=w329, type=T22 {"DI Config"={"DI Tasks"=[]}, "DO Config"={"DO Channels"=[]}, "AI Config"={"AI Tasks"=[]}, "AO Config"={"AO Channels"=[]}} ("IO Nodes"), Variant=w330) -> (data=w325:T22, error out=w324:errorcluster)
        n102 = Bundle By Name(cluster=w327, "IO Nodes"=w325) -> (w326:T61)
      }
      frame "Data: Read Init XML" {
        # "Init XML File"
        n103 = call "FG - FilePathnames.vi"() -> ("FilePaths out"=w343:T64)  [unwired: 4 in, 1 out]
        n104 = Unbundle By Name(w343) -> ("PrinterInitXMLFile"=w342:path)
        n105 = Unbundle By Name(w341) -> ("DLP"=w345:T18)
        n106 = call <vilib>:"Easy Read XML File__JKI EasyXML.vi"("error in (no error)"=w338, "LabVIEW Data (Type)"=w345, "XML File Path"=w342) -> ("error out"=w340:errorcluster, "LabVIEW Data"=w344:variant)  [unwired: 6 in, 1 out]
        n107 = Variant To Data(error in=w340, type=T18 {"PrinterInitialization"={"Printer"={"#attributes"={"Name"=""}}, "VacPumpSet"={"#attributes"={"VacPumpEnable"=FALSE, "VacPumpSpeed"=0.0}}, "HIBEnable"={"#attributes"={"HIB1Enable"=FALSE, "HIB2Enable"=FALSE, "HIB3Enable"=FALSE, "HIB4Enable"=FALSE, "HIB5Enable"=FALSE, "HIB6Enable"=FALSE}}, "PrinterCompensation"={"#attributes"={"AppName"="", "PrintWeightMultiplier"=0.0, "Rotation"=FALSE, "Driver"="", "Server"="", "Database"="", "User"="", "Password"=""}}}, "HeadSet"={"HeadProperties"=[]}, "InkSet"={"Ink"=[]}, "Troubleshooting"={"PMBLogging"={"#attributes"={"PMBMonitorDuringPrint"=FALSE, "PMBMonitorDuringIdle"=FALSE, "LogSwatheInputData"=FALSE, "LogSwatheOutputData"=FALSE, "LogPrintheadColourPlanes"=FALSE, "LogPMBCommunication"=FALSE, "LogSimulatedOutput"=FALSE, "LogAllPMBCommunicationData"=FALSE, "LogPMBSpace"=FALSE, "ExtendedPMBSpaceLogging"=FALSE, "LogPMBWriteSpeed"=FALSE, "LogUsbRetries"=FALSE}}, "HIBLogging"={"#attributes"={"HIBMonitoringDuringPrint"=FALSE, "HIBMonitoringLog"=FALSE}}}} ("DLP"), Variant=w344) -> (data=w336:T18, error out=w339:errorcluster)
        n108 = Bundle By Name(cluster=w341, "DLP"=w336) -> (w337:T61)
      }
      frame "Data: ReadPersistentData" {
        n109 = call "FG - FilePathnames.vi"() -> ("FilePaths out"=w357:T64)  [unwired: 4 in, 1 out]
        n110 = Unbundle By Name(w357) -> ("PersistentXMLFile"=w355:path)
        n111 = Unbundle By Name(w353) -> ("TopLevel in"=w350:refnum<class "TopLevel.lvclass">)
        n112 = call "Persistent_XML_Read.vi"("error in (no error)"=w354, "Persistent XML File Path"=w355) -> ("error out"=w349:errorcluster, "PersistentData"=w351:T65)  [unwired: 8 in]
        n113 = call-dynamic "Write PersistentXML.vi"("error in (no error)"=w349, "PersistentData"=w351, "TopLevel in"=w350) -> ("error out"=w348:errorcluster, "TopLevel out"=w352:refnum<class "TopLevel.lvclass">)  [unwired: 7 in]
        n114 = Bundle By Name(cluster=w353, "TopLevel in"=w352) -> (w356:T61)
      }
      frame "Data: Cleanup" {
        n115 = Unbundle By Name(w361) -> ("Core.Current VI Reference"=w364:refnum<vi>)
        n116 = Close Reference(reference=w364, error in (no error)=w363) -> (error out=w362:errorcluster)
        n117 = call <vilib>:"Add State(s) to Queue__JKI_lib_State_Machine.vi"("State(s) in (\"\")"=w366) -> ("States Out"=w365:string)  [unwired: 14 in]
      }
      frame "---------- UI ----------" {
        n118 = call <vilib>:"Add State(s) to Queue__JKI_lib_State_Machine.vi"("State(s) in (\"\")"=w371) -> ("States Out"=w370:string)  [unwired: 14 in]
      }
      frame "UI: Initialize" {
        n119 = call <userlib>:"Fit VI window to Largest Dec__ogtk.vi"("error in (no error)"=w373) -> ("error out"=w372:errorcluster)  [unwired: 5 in, 1 out]
        n120 = call <vilib>:"Add State(s) to Queue__JKI_lib_State_Machine.vi"("State(s) in (\"\")"=w377) -> ("States Out"=w376:string)  [unwired: 14 in]
      }
      frame "UI: Cursor Set" {
        # "Argument"
        n121 = case shown="\"Idle\", Default" w379 {
          tunnel: w381 -> [w386 w388]
          tunnel: [w385 w387] -> w380
          frame "Idle", Default {
            n122 = call <vilib>:"Unset Busy.vi"("error in (no error)"=w386) -> ("error out"=w385:errorcluster)  [unwired: 10 in]
          }
          frame "Busy" {
            n123 = call <vilib>:"Set Busy.vi"("error in (no error)"=w388) -> ("error out"=w387:errorcluster)  [unwired: 9 in, 1 out]
          }
        }
        n124 = call <vilib>:"Add State(s) to Queue__JKI_lib_State_Machine.vi"("State(s) in (\"\")"=w384) -> ("States Out"=w383:string)  [unwired: 14 in]
      }
      frame "UI: Front Panel State" {
        # "Argument"
        n125 = Unbundle By Name(w392) -> ("Core.Current VI Reference"=w391:refnum<vi>)
        n126 = case shown="\"Open\", Default" w390 {
          tunnel: w394 -> [w400 w413]
          tunnel: [w402 w414] -> w393
          tunnel: w391 -> [w401 w411]
          frame "Open", Default {
            n127 = property class="VI"(reference=w401, error in=w400) -> (reference out=w398:refnum<vi>, error out=w399:errorcluster, "Front Panel.Open"=w397:bool)
            n128 = case shown="False" w397 {
              tunnel: [w405 w408] -> w402
              tunnel: w399 -> [w404 w408]
              tunnel: w398 -> [w403 _]
              frame False {
                n129 = invoke class="VI" method="FP.Open"(reference=w403, error in=w404, "Activate"=TRUE, "State"=T49."Standard") -> (error out=w405:errorcluster)  [unwired: 1 in, 4 out]
              }
              frame True {
              }
            }
          }
          frame "Close" {
            n130 = property class="VI"(reference=w411, error in=w413) -> (reference out=w410:refnum<vi>, error out=w412:errorcluster, "Front Panel.Open"=w409:bool)
            n131 = case shown="True" w409 {
              tunnel: [w415 w418] -> w414
              tunnel: w412 -> [w415 w417]
              tunnel: w410 -> [_ w416]
              frame False {
              }
              frame True {
                n132 = invoke class="VI" method="FP.Close"(reference=w416, error in=w417) -> (error out=w418:errorcluster)  [unwired: 1 in, 2 out]
              }
            }
          }
        }
        n133 = call <vilib>:"Add State(s) to Queue__JKI_lib_State_Machine.vi"("State(s) in (\"\")"=w396) -> ("States Out"=w395:string)  [unwired: 14 in]
      }
      frame "---------- Macro ----------" {
        n134 = call <vilib>:"Add State(s) to Queue__JKI_lib_State_Machine.vi"("State(s) in (\"\")"=w423) -> ("States Out"=w422:string)  [unwired: 14 in]
      }
      frame "Macro: Execute PrePurgeGIS" {
        # "GIS: Execute Command\nPre Purge: Wait\nCheckIfPrePurgeRepeatsDone\nTask: Completed"
        n135 = Unbundle By Name(w435) -> ("PPScanTrk.TotalRepeats"=w433:i32, "PPScanTrk.CurrentScan"=w434:i32, "TopLevel in"=w428:refnum<class "TopLevel.lvclass">)
        n136 = Increment(x=w434) -> (x+1=w427:i32)
        n137 = Greater?(x=w427, y=w433) -> (0:w426:bool)
        n138 = Bundle By Name(cluster=w435, "PPScanTrk.CurrentScan"=w427) -> (w432:T61)
        n139 = case shown="False" w426 {
          tunnel: w428 -> [w442 _]
          tunnel: w427 -> [w441 _]
          tunnel: w424 -> [w440 w443]
          tunnel: [w439 w443] -> w425
          frame False {
            n140 = call-dynamic "Set PrePurgePrintCount_StatusChangedEvent.vi"("error in (no error)"=w440, "Status.PrePurgePrintNo"=w441, "TopLevel in"=w442) -> ("error out"=w439:errorcluster)  [unwired: 7 in, 1 out]
          }
          frame True {
          }
        }
        n141 = Select(t="Task: Completed" ("State(s) in Front (\"\")"), s=w426, f="GIS: Execute Command\nPre Purge: Wait\nMacro: Execute PrePurgeGIS" ("State(s) in Front (\"\")")) -> (s? t:f=w429:string)
        n142 = call <vilib>:"Add State(s) to Queue__JKI_lib_State_Machine.vi"("State(s) in Front (\"\")"=w429, "State(s) in (\"\")"=w438) -> ("States Out"=w437:string)  [unwired: 13 in]
      }
      frame "Macro: ExecutePrimingScan" {
        # "Prime Wait is actually theinterval. the duration is sent through a command"
        # "#TODO rename pre purge:wait frame"
        # "GIS: Execute Command\nPre Purge: Wait\nCheckIfPrePurgeRepeatsDone\nTask: Completed"
        n143 = Unbundle By Name(w457) -> ("PMScanTrk.CurrentScan"=w456:i32, "PMScanTrk.TotalRepeats"=w446:i32, "TopLevel in"=w452:refnum<class "TopLevel.lvclass">, "PrinterModeAPI Data.PrimingMode"=w445:T9, "PrinterModeAPI Data"=w444:T8)
        n144 = Increment(x=w456) -> (x+1=w451:i32)
        n145 = Bundle By Name(cluster=w457, "PMScanTrk.CurrentScan"=w451) -> (w455:T61)
        n146 = Greater?(x=w451, y=w446) -> (0:w450:bool)
        n147 = case shown="False" w450 {
          tunnel: w452 -> [w477 _]
          tunnel: w451 -> [w476 _]
          tunnel: w448 -> [w475 w478]
          tunnel: [w474 w478] -> w449
          frame False {
            n148 = call-dynamic "Set PrePurgePrintCount_StatusChangedEvent.vi"("error in (no error)"=w475, "Status.PrePurgePrintNo"=w476, "TopLevel in"=w477) -> ("error out"=w474:errorcluster)  [unwired: 7 in, 1 out]
          }
          frame True {
          }
        }
        n149 = case shown="\"Purge\"" w445 {
          tunnel: ["GIS: Send and Execute Command\nPrime: Wait\nMacro: ExecutePrimingScan" ("State(s) in Front (\"\")") w462 "Action: Purge\nPrime: Wait\nMacro: ExecutePrimingScan" ("State(s) in Front (\"\")")] -> w447
          tunnel: w444 -> [_ w466 _]
          frame "Spit", "Shake", Default {
          }
          frame "Pre-Purge" {
            n150 = Unbundle By Name(w466) -> ("Head"=w465:T10)
            n151 = case shown="\"6\"" w465 {
              tunnel: [ICP1-D0_Channel_Names."Purge Valve Open - R1" ("Purge Channel Name") ICP1-D0_Channel_Names."Purge Valve Open - R2" ("Purge Channel Name") ICP1-D0_Channel_Names."Purge Valve Open - R3" ("Purge Channel Name") ICP1-D0_Channel_Names."Purge Valve Open - R4" ("Purge Channel Name") ICP1-D0_Channel_Names."Purge Valve Open - R5" ("Purge Channel Name") ICP1-D0_Channel_Names."Purge Valve Open - R6" ("Purge Channel Name")] -> w464
              frame "1", Default {
              }
              frame "2" {
              }
              frame "3" {
              }
              frame "4" {
              }
              frame "5" {
              }
              frame "6" {
              }
            }
            n152 = Format Into String(format string="GIS: Send and Execute Command>>0\nAction: SyncWait>>2\nPurge: Set DOChannel>>%s\nGIS: Send and Execute Command>>1\nPrime: Wait\nMacro: ExecutePrimingScan", w464) -> (resulting string=w462:string)  [unwired: 2 in, 1 out]
          }
          frame "Purge" {
          }
        }
        n153 = Select(t="Action: SendStatusPollEnable>>TRUE\nTask: Completed" ("State(s) in Front (\"\")"), s=w450, f=w447) -> (s? t:f=w453:string)
        n154 = call <vilib>:"Add State(s) to Queue__JKI_lib_State_Machine.vi"("State(s) in Front (\"\")"=w453, "State(s) in (\"\")"=w460) -> ("States Out"=w459:string)  [unwired: 13 in]
      }
      frame "Macro: Execute Print" {
        # "End Routine with Home"
        # "Start the routine with a Home Move\nAll subsequent moves are back to 0"
        n155 = Unbundle By Name(w500) -> ("HomeOnComplete"=w485:bool, "PrintScanTrk.TotalRepeats"=w495:i32, "PrintScanTrk.CurrentScan"=w492:i32)  [unwired: 1 out]
        n156 = Equal To 0?(x=w492) -> (x = 0?=w491:bool)
        n157 = Select(t="MoveStage>>Home" ("State(s) in Front (\"\")"), s=w491, f="MoveStage>>Load" ("State(s) in Front (\"\")")) -> (s? t:f=w488:string)
        n158 = Format Into String(format string="%s\nIdle\nGIS: Execute Command\nIdle\nMacro: Execute Print" ("State(s) in Front (\"\")"), w488) -> (resulting string=w486:string)  [unwired: 2 in, 1 out]
        n159 = Greater?(x=w495, y=1) -> (0:w496:bool)
        n160 = Select(t=w486, s=w496, f="GIS: Execute Command\nIdle\nMacro: Execute Print" ("State(s) in Front (\"\")")) -> (s? t:f=w493:string)
        n161 = Increment(x=w492) -> (x+1=w481:i32)
        n162 = Greater?(x=w481, y=w495) -> (0:w480:bool)
        n163 = Bundle By Name(cluster=w500, "PrintScanTrk.CurrentScan"=w481) -> (w499:T61)
        n164 = Select(t="Action: SendStatusPollEnable>>TRUE\nMoveStage>>Home\nTask: Completed" ("State(s) in Front (\"\")"), s=w485, f="Action: SendStatusPollEnable>>TRUE\n/*MoveStage>>Home\nTask: Completed" ("State(s) in Front (\"\")")) -> (s? t:f=w482:string)
        n165 = Select(t=w482, s=w480, f=w493) -> (s? t:f=w498:string)
        n166 = call <vilib>:"Add State(s) to Queue__JKI_lib_State_Machine.vi"("State(s) in Front (\"\")"=w498, "State(s) in (\"\")"=w503) -> ("States Out"=w502:string)  [unwired: 13 in]
      }
      frame "Macro: Execute Idle Print" {
        # "End Routine with Home"
        # "Start the routine with a Home Move\nAll subsequent moves are back to 0"
        n167 = Unbundle By Name(w516) -> ("Idle Mode"=w506:bool, "PrintScanTrk.CurrentScan"=w505:i32)
        n168 = Equal To 0?(x=w505) -> (x = 0?=w511:bool)
        n169 = Select(t="MoveStage>>Home" ("State(s) in Front (\"\")"), s=w511, f="MoveStage>>Load" ("State(s) in Front (\"\")")) -> (s? t:f=w508:string)
        n170 = Format Into String(format string="Idle\n%s\nIdle\nGIS: Execute Command\nIdle\nWaitAsync>>Initialize\nMacro: Execute Idle Print" ("State(s) in Front (\"\")"), w508) -> (resulting string=w504:string)  [unwired: 2 in, 1 out]
        n171 = Increment(x=w505) -> (x+1=w514:i32)
        n172 = Bundle By Name(cluster=w516, "PrintScanTrk.CurrentScan"=w514) -> (w515:T61)
        n173 = Select(t=w504, s=w506, f="MoveStage>>Home\nTask: Completed" ("State(s) in Front (\"\")")) -> (s? t:f=w512:string)
        n174 = call <vilib>:"Add State(s) to Queue__JKI_lib_State_Machine.vi"("State(s) in Front (\"\")"=w512, "State(s) in (\"\")"=w520) -> ("States Out"=w519:string)  [unwired: 13 in]
      }
      frame "Macro: Initialize" {
        n175 = call <vilib>:"Add State(s) to Queue__JKI_lib_State_Machine.vi"("State(s) in (\"\")"=w521) -> ("States Out"=w524:string)  [unwired: 14 in]
      }
      frame "Macro: Exit" {
        n176 = call <vilib>:"Add State to Queue with vData.vi"("queue in"=w529, "state in"="Exit", "error in"=w526) -> ("error out"=w527:errorcluster)  [unwired: 9 in, 3 out]
        n177 = Unbundle By Name(w537) -> ("Core.Close Panel on Exit?"=w536:bool)
        n178 = Select(t="UI: Front Panel State >> Close", s=w536, f="") -> (s? t:f=w533:string)
        n179 = call <vilib>:"Add State(s) to Queue__JKI_lib_State_Machine.vi"("State(s) in (\"\")"=w533, "State(s) at Back (\"\")"="System: Shutdown\nData: Cleanup\nEvents: Unregister Events\nExit") -> ("States Out"=w531:string)  [unwired: 13 in]
        n180 = call <vilib>:"Add State(s) to Queue__JKI_lib_State_Machine.vi"("State(s) in Front (\"\")"=w531, "State(s) in (\"\")"=w539) -> ("States Out"=w538:string)  [unwired: 13 in]
      }
      frame "---------- Events ----------" {
      }
      frame "Events: Register Events" {
        n181 = Unbundle By Name(w560) -> ("TopLevel in"=w559:refnum<class "TopLevel.lvclass">, "LaunchData"=w551:refnum<user-event>, "DAQ"=w549:refnum<class "DAQ.lvclass">)
        n182 = call "Get Public Events.vi"("error in (no error)"=w545, "DAQ"=w549) -> ("error out"=w546:errorcluster, "PublicEvents"=w548:T66)  [unwired: 7 in, 1 out]
        n183 = call-dynamic "GetEvents_TopLevel.vi"("error in (no error)"=w546, "TopLevel in"=w559) -> ("error out"=w558:errorcluster, "UserEvents"=w557:T67)  [unwired: 7 in, 1 out]
        n184 = Unbundle By Name(w548) -> ("DIStateChangeEv"=w547:refnum<user-event>)
        n185 = Unbundle By Name(w557) -> ("API Return Event"=w554:refnum<user-event>, "API Incoming Event"=w556:refnum<user-event>, "API Executed Event"=w553:refnum<user-event>, "Exit Event"=w552:refnum<user-event>, "HeadPrimeStatusEvent"=w544:refnum<user-event>)
        n186 = register-events(w556, w553, w552, w551, w547, w544) -> (reference out=w550:refnum<event-registration>)  [unwired: 2 in, 1 out]
        n187 = Bundle By Name(cluster=w560, "API Return Event"=w554, "API Executed Event"=w553) -> (w555:T61)
        n188 = call <vilib>:"Add State(s) to Queue__JKI_lib_State_Machine.vi"("State(s) in (\"\")"=w562) -> ("States Out"=w561:string)  [unwired: 14 in]
      }
      frame "Events: Unregister Events" {
      }
      frame "---------- API ----------" {
      }
      frame "API: WriteInitXML" {
        # "Init XML File"
        n189 = Unbundle By Name(w580) -> ("TopLevel in"=w573:refnum<class "TopLevel.lvclass">, "Current Task.Data"=w581:variant)
        n190 = Variant To Data(error in=w579, type=T18 {"PrinterInitialization"={"Printer"={"#attributes"={"Name"=""}}, "VacPumpSet"={"#attributes"={"VacPumpEnable"=FALSE, "VacPumpSpeed"=0.0}}, "HIBEnable"={"#attributes"={"HIB1Enable"=FALSE, "HIB2Enable"=FALSE, "HIB3Enable"=FALSE, "HIB4Enable"=FALSE, "HIB5Enable"=FALSE, "HIB6Enable"=FALSE}}, "PrinterCompensation"={"#attributes"={"AppName"="", "PrintWeightMultiplier"=0.0, "Rotation"=FALSE, "Driver"="", "Server"="", "Database"="", "User"="", "Password"=""}}}, "HeadSet"={"HeadProperties"=[]}, "InkSet"={"Ink"=[]}, "Troubleshooting"={"PMBLogging"={"#attributes"={"PMBMonitorDuringPrint"=FALSE, "PMBMonitorDuringIdle"=FALSE, "LogSwatheInputData"=FALSE, "LogSwatheOutputData"=FALSE, "LogPrintheadColourPlanes"=FALSE, "LogPMBCommunication"=FALSE, "LogSimulatedOutput"=FALSE, "LogAllPMBCommunicationData"=FALSE, "LogPMBSpace"=FALSE, "ExtendedPMBSpaceLogging"=FALSE, "LogPMBWriteSpeed"=FALSE, "LogUsbRetries"=FALSE}}, "HIBLogging"={"#attributes"={"HIBMonitoringDuringPrint"=FALSE, "HIBMonitoringLog"=FALSE}}}} ("InitXML"), Variant=w581) -> (data=w575:T18, error out=w574:errorcluster)
        n191 = call "FG - FilePathnames.vi"() -> ("FilePaths out"=w577:T64)  [unwired: 4 in, 1 out]
        n192 = Unbundle By Name(w577) -> ("PrinterInitXMLFile"=w576:path)
        n193 = call "DLPConfigInitialization_XML_Write.vi"("error in (no error)"=w574, "DLP"=w575, "Recipe XML File Path"=w576) -> ("error out"=w572:errorcluster)  [unwired: 8 in]
        n194 = call "PopulateHeadPropertiesInConfigDict.vi"("error in (no error)"=w572, "TopLevel in"=w573) -> ("error out"=w571:errorcluster)  [unwired: 7 in, 2 out]
      }
      frame "API: SetHeadTemperature" {
        # "P,C,P,PH%s_Enable"
        n195 = Unbundle By Name(w595) -> ("Current Task.Data"=w589:variant)
        n196 = Variant To Data(error in=w590, type=T50 {"Head"=enum."1", "SetPoint"=0.0}, Variant=w589) -> (data=w594:T50, error out=w591:errorcluster)
        n197 = Unbundle By Name(w594) -> ("Head"=w593:T10, "SetPoint"=w592:dbl)
        n198 = Format Into String(format string="P,C,P,PH%s_Temp_Set,%f", error in=w591, w593, w592) -> (resulting string=w598:string, error out=w597:errorcluster)  [unwired: 1 in]
        n199 = Build Array(w598) -> (w584:string[])
        n200 = Bundle By Name(cluster=w595, "GIS Commands"=w584) -> (w600:T61)
        n201 = call <vilib>:"Add State(s) to Queue__JKI_lib_State_Machine.vi"("State(s) in Front (\"\")"="GIS: Send and Execute Command>>0\nTask: Completed" ("State(s) in Front (\"\")"), "State(s) in (\"\")"=w586) -> ("States Out"=w587:string)  [unwired: 13 in]
      }
      frame "API: Send Printer String" {
        # "P,C,P,PH%s_Enable"
        n202 = Unbundle By Name(w611) -> ("Current Task.Data"=w609:variant)
        n203 = Variant To Data(error in=w610, type="", Variant=w609) -> (data=w602:string, error out=w601:errorcluster)
        n204 = Build Array(w602) -> (w604:string[])
        n205 = Bundle By Name(cluster=w611, "GIS Commands"=w604) -> (w612:T61)
        n206 = call <vilib>:"Add State(s) to Queue__JKI_lib_State_Machine.vi"("State(s) in Front (\"\")"="GIS: Send and Execute Command>>0\nTask: Completed" ("State(s) in Front (\"\")"), "State(s) in (\"\")"=w606) -> ("States Out"=w607:string)  [unwired: 13 in]
      }
      frame "API: EnableHead" {
        # "not used"
        n207 = Unbundle By Name(w624) -> ("Current Task.Data"=w618:variant)
        n208 = Variant To Data(error in=w619, type=T51 {"Head"=enum."1", "Enable"=FALSE} ("Cluster"), Variant=w618) -> (data=w623:T51, error out=w620:errorcluster)
        n209 = Unbundle By Name(w623) -> ("Head"=w622:T10, "Enable"=w621:bool)
        n210 = Format Into String(format string="P,C,P,PH%s_Enable,%s", error in=w620, w622, w621) -> (resulting string=w626:string, error out=w625:errorcluster)  [unwired: 1 in]
        n211 = Build Array(w626) -> (w613:string[])
        n212 = Bundle By Name(cluster=w624, "GIS Commands"=w613) -> (w628:T61)
        n213 = call <vilib>:"Add State(s) to Queue__JKI_lib_State_Machine.vi"("State(s) in Front (\"\")"="GIS: Send and Execute Command>>0\nTask: Completed" ("State(s) in Front (\"\")"), "State(s) in (\"\")"=w614) -> ("States Out"=w615:string)  [unwired: 13 in]
      }
      frame "API: SetSystemMode" {
        w632 = ""  # SystemMode
        n214 = Unbundle By Name(w639) -> ("Current Task.Data"=w636:variant)
        n215 = Variant To Data(error in=w637, type=w632, Variant=w636) -> (data=w631:string, error out=w638:errorcluster)
        n216 = Format Into String(format string="S,T,M,%s", error in=w638, w631) -> (resulting string=w641:string, error out=w640:errorcluster)  [unwired: 1 in]
        n217 = Build Array(w641) -> (w630:string[])
        n218 = Bundle By Name(cluster=w639, "GIS Commands"=w630) -> (w643:T61)
        n219 = call <vilib>:"Add State(s) to Queue__JKI_lib_State_Machine.vi"("State(s) in Front (\"\")"="GIS: Send and Execute Command>>0\nTask: Completed" ("State(s) in Front (\"\")"), "State(s) in (\"\")"=w633) -> ("States Out"=w634:string)  [unwired: 13 in]
      }
      frame "API: EnableHeadHeat" {
        (unwired) "P,C,P,PH%s_Heat,%s"
        # "P,C,P,HIB%s_Heat,%s\nP,C,P,PH%s_Heat,%s"
        # "Enable heater"
        n220 = Unbundle By Name(w656) -> ("Current Task.Data"=w652:variant)
        n221 = Variant To Data(error in=w653, type=T51 {"Head"=enum."1", "Enable"=FALSE} ("Cluster"), Variant=w652) -> (data=w655:T51, error out=w654:errorcluster)
        n222 = Unbundle By Name(w655) -> ("Head"=w646:T10, "Enable"=w645:bool)
        n223 = Format Into String(format string="P,C,P,HIB%d_Heat,%s\nP,C,P,PH%d_Heat,%s", error in=w654, w646, w645, w646, w645) -> (resulting string=w658:string, error out=w657:errorcluster)  [unwired: 1 in]
        n224 = Build Array(w658) -> (w647:string[])
        n225 = Bundle By Name(cluster=w656, "GIS Commands"=w647) -> (w660:T61)
        n226 = call <vilib>:"Add State(s) to Queue__JKI_lib_State_Machine.vi"("State(s) in Front (\"\")"="GIS: Send and Execute Command>>0\nTask: Completed" ("State(s) in Front (\"\")"), "State(s) in (\"\")"=w648) -> ("States Out"=w649:string)  [unwired: 13 in]
      }
      frame "API: LoadDLP2GUIConfig" {
        n227 = disable-structure shown="Enabled" {
          disable-tunnel: [w680 w685] -> w665
          disable-tunnel: w664 -> [w679 w685]
          disable-tunnel: w663 -> [w674 w684]
          disable-tunnel: [w670 w684] -> w662
          frame Enabled {
            # "fire event"
            n228 = Unbundle By Name(w679) -> ("Current Task.Data"=w678:variant, "MasterConfigurationDLPC2"=w683:T3, "TopLevel in"=w673:refnum<class "TopLevel.lvclass">)
            n229 = Variant To Data(error in=w674, type=path "", Variant=w678) -> (data=w676:path, error out=w675:errorcluster)
            n230 = call <vilib>:"Easy Read XML File__JKI EasyXML.vi"("LabVIEW Data (Type)"=w683, "XML File Path"=w676) -> ("LabVIEW Data"=w682:variant)  [unwired: 7 in, 2 out]
            n231 = Variant To Data(error in=w675, type=T3 {"Paths"={"DigiBit WG Design Folder"=path "", "Compensated GS Image Folder"=path "", "Nozzle GS Files Head 1"=path "", "Nozzle GS Files Head 2"=path "", "Nozzle GS Files Head 3"=path "", "Nozzle GS Files Head 4"=path "", "Nozzle GS Files Head 5"=path "", "Nozzle GS Files Head 6"=path ""}, "ColorPaneMapping"={"Head 1"={"Material"="", "ColorPane"=""}, "Head 2"={"Material"="", "ColorPane"=""}, "Head 3"={"Material"="", "ColorPane"=""}, "Head 4"={"Material"="", "ColorPane"=""}, "Head 5"={"Material"="", "ColorPane"=""}, "Head 6"={"Material"="", "ColorPane"=""}}, "Materials"=[], "ColorPlanes"=[], "SpitVoltages_Half"={"1"=0.0, "2"=0.0, "3"=0.0, "4"=0.0, "5"=0.0, "6"=0.0}, "SpitVoltages_Full"={"1"=0.0, "2"=0.0, "3"=0.0, "4"=0.0, "5"=0.0, "6"=0.0}, "SystemMode"=[], "PrimeModeConfig"=[], "Running Average Duration_s"=5.0} ("MasterConfigurationDLPC2"), Variant=w682) -> (data=w672:T3, error out=w671:errorcluster)
            n232 = Bundle By Name(cluster=w679, "MasterConfigurationDLPC2"=w672) -> (w680:T61)
            n233 = call-dynamic "TriggerDLP2GUIConfigLoadedEvent.vi"("error in (no error)"=w671, "MasterConfigurationDLPC2"=w672, "TopLevel in"=w673) -> ("error out"=w670:errorcluster)  [unwired: 7 in, 1 out]
          }
          frame Disabled {
          }
        }
        n234 = call <vilib>:"Add State(s) to Queue__JKI_lib_State_Machine.vi"("State(s) in Front (\"\")"="Task: Completed" ("State(s) in Front (\"\")"), "State(s) in (\"\")"=w666) -> ("States Out"=w667:string)  [unwired: 13 in]
      }
      frame "API: Execute Printer Commands" {
        n235 = Unbundle By Name(w699) -> ("Current Task.Data"=w698:variant)
        n236 = Variant To Data(error in=w697, type=T52 {"Command File Path"=path "", "No. of Print Repeats"=1, "HomeOnComplete"=FALSE}, Variant=w698) -> (data=w691:T52, error out=w694:errorcluster)
        n237 = Unbundle By Name(w691) -> ("Command File Path"=w690:path, "No. of Print Repeats"=w688:i32, "HomeOnComplete"=w686:bool)
        n238 = Bundle By Name(cluster=w699, "Printer Command File Path"=w690, "PrintScanTrk.TotalRepeats"=w688, "HomeOnComplete"=w686, "PrintScanTrk.CurrentScan"=0) -> (w693:T61)
        n239 = call <vilib>:"Add State(s) to Queue__JKI_lib_State_Machine.vi"("State(s) in Front (\"\")"="Action: SendStatusPollEnable>>FALSE\nMacro: Execute Print" ("State(s) in Front (\"\")"), "State(s) in (\"\")"=w695) -> ("States Out"=w696:string)  [unwired: 13 in]
      }
      frame "API: ExecuteIdlePrintCycle" {
        n240 = Unbundle By Name(w714) -> ("Current Task.Data"=w713:variant)
        n241 = Variant To Data(error in=w712, type=T53 {"Command File Path"=path "", "IdleMode"=FALSE, "IdleCycleInterval(s)"=0.0} ("Cluster"), Variant=w713) -> (data=w707:T53, error out=w709:errorcluster)
        n242 = Unbundle By Name(w707) -> ("Command File Path"=w706:path, "IdleMode"=w703:bool, "IdleCycleInterval(s)"=w702:dbl)
        n243 = Bundle By Name(cluster=w714, "Printer Command File Path"=w706, "Idle Mode"=w703, "IdleTimer"=w702, "PrintScanTrk.CurrentScan"=0) -> (w708:T61)
        n244 = call <vilib>:"Add State(s) to Queue__JKI_lib_State_Machine.vi"("State(s) in Front (\"\")"="Macro: Execute Idle Print" ("State(s) in Front (\"\")"), "State(s) in (\"\")"=w710) -> ("States Out"=w711:string)  [unwired: 13 in]
      }
      frame "API: Pre Purge" {
        n245 = Unbundle By Name(w728) -> ("Current Task.Data"=w727:variant)
        n246 = Variant To Data(error in=w726, type=T36 {"Purge Channel Name"=enum."Purge Valve Open - R1", "GIS File Path"=path "", "Duration (s)"=0.1, "PurgeDuration (s)"=0.1, "Repeats"=0} ("Pre Purge API Data"), Variant=w727) -> (data=w718:T36, error out=w722:errorcluster)
        n247 = Unbundle By Name(w718) -> ("Repeats"=w716:u8, "GIS File Path"=w719:path)
        n248 = Bundle By Name(cluster=w728, "PPScanTrk.CurrentScan"=0, "PPScanTrk.TotalRepeats"=w716, "Pre Purge API Data"=w718, "Printer Command File Path"=w719) -> (w721:T61)
        n249 = call <vilib>:"Add State(s) to Queue__JKI_lib_State_Machine.vi"("State(s) in Front (\"\")"="Purge: Send Command\nMacro: Execute PrePurgeGIS" ("State(s) in Front (\"\")"), "State(s) in (\"\")"=w724) -> ("States Out"=w725:string)  [unwired: 13 in]
      }
      frame "API: PrimingMode" {
        n250 = Unbundle By Name(w743) -> ("TopLevel in"=w730:refnum<class "TopLevel.lvclass">, "Current Task.Data"=w742:variant)
        n251 = Variant To Data(error in=w741, type=T8 {"Interval (s)"=0.1, "PurgeDuration (s)"=0.1, "Repeats"=0, "PrimingMode"=enum."Pre-Purge", "Head"=enum."1", "Frequency (Hz)"=0, "PrintWeight"=0.1} ("Pre Purge API Data"), Variant=w742) -> (data=w733:T8, error out=w732:errorcluster)
        n252 = call "Generate GIS Script.vi"("TopLevel in"=w730, "error in"=w732, "Priming API Data"=w733) -> ("error out"=w731:errorcluster, "GIS Script"=w734:string[], "PPScanTrk"=w735:T60)  [unwired: 5 in, 1 out]
        n253 = disable-structure shown="Enabled" {
          disable-tunnel: w743 -> [w750 _]
          disable-tunnel: ["Action: SendStatusPollEnable>>FALSE\nMacro: ExecutePrimingScan" ("State(s) in Front (\"\")") "Task: Completed" ("State(s) in Front (\"\")")] -> w738
          disable-tunnel: [w748 _] -> w737
          disable-tunnel: w735 -> [w747 _]
          disable-tunnel: w734 -> [w746 _]
          disable-tunnel: w733 -> [w745 _]
          frame Enabled {
            n254 = Bundle By Name(cluster=w750, "PrinterModeAPI Data"=w745, "PMScanTrk"=w747, "GIS Commands"=w746) -> (w748:T61)
          }
          frame Disabled {
          }
        }
        n255 = call <vilib>:"Add State(s) to Queue__JKI_lib_State_Machine.vi"("State(s) in Front (\"\")"=w738, "State(s) in (\"\")"=w739) -> ("States Out"=w740:string)  [unwired: 13 in]
      }
      frame "API: HeadPrint" {
        n256 = Unbundle By Name(w776) -> ("Current Task.Data"=w775:variant, "TopLevel in"=w755:refnum<class "TopLevel.lvclass">)
        n257 = Variant To Data(error in=w774, type=T54 {"PrintImageFile"="", "PrintPass"=1, "EncoderSource"="", "PrintGoSource"="", "Head"=enum."1"} ("HeadPrint Data"), Variant=w775) -> (data=w768:T54, error out=w754:errorcluster)
        n258 = Unbundle By Name(w768) -> ("PrintImageFile"=w767:string, "PrintPass"=w766:u8)
        n259 = Format Into String(format string="P,C,P,\"Print Manager,Print Line Manager,PMB,PrintGoSource\",\"TTL\"\nP,C,P,\"Print Manager,Print Line Manager,PMB,EncoderSource\",\"RS422\"\nP,P,1,%s,%d", w767, 1) -> (resulting string=w765:string)  [unwired: 2 in, 1 out]
        n260 = for {
          N: w766 -> [_]
          tunnel: w765 -> [w786]
          tunnel: [w786] -> w764 mode=indexing
          tunnel: "MoveStage>>Load\nIdle\nGIS: Send and Execute Command>>%d\nAction: Send Event>>CalPrintCount>>%d" -> [w785]
          tunnel: [w784] -> w762 mode=indexing
          i -> [w782]
          n261 = Increment(x=w782) -> (x+1=w783:i32)
          n262 = Format Into String(format string=w785, w782, w783) -> (resulting string=w784:string)  [unwired: 2 in, 1 out]
        }
        n263 = Bundle By Name(cluster=w776, "GIS Commands"=w764) -> (w771:T61)
        n264 = Array To Spreadsheet String(delimiter (Tab)="\n", array=w762, 3:"" ("format string")) -> (spreadsheet string=w759:string)
        n265 = call <vilib>:"Trim Whitespace.vi"("string"=w759) -> ("trimmed string"=w758:string)  [unwired: 1 in]
        n266 = call-dynamic "SetTopLevel Busy_StatusChangedEvent.vi"("error in (no error)"=w754, "Status.Busy"=TRUE, "TopLevel in"=w755) -> ("error out"=w753:errorcluster)  [unwired: 7 in, 1 out]
        n267 = disable-structure shown="Enabled" {
          disable-tunnel: w758 -> [w780 _]
          disable-tunnel: [w778 "Task: Completed" ("State(s) in Front (\"\")")] -> w757
          frame Enabled {
            n268 = Format Into String(format string="Action: Send Event>>CalPrintCount>>0\nAction: SendStatusPollEnable>>FALSE\n%s\nAction: SendStatusPollEnable>>TRUE\nTask: Completed", w780) -> (resulting string=w778:string)  [unwired: 2 in, 1 out]
          }
          frame Disabled {
          }
        }
        n269 = call <vilib>:"Add State(s) to Queue__JKI_lib_State_Machine.vi"("State(s) in Front (\"\")"=w757, "State(s) in (\"\")"=w772) -> ("States Out"=w773:string)  [unwired: 13 in]
      }
      frame "API: Enable Ink Ch-1" {
        w823 = TRUE
        w824 = PrinterHeads--Enum."1" ("Head")
        # "#todo ask If meniscus valve can be"
        # "enable head"
        n270 = Unbundle By Name(w827) -> ("TopLevel in"=w787:refnum<class "TopLevel.lvclass">, "DAQ"=w819:refnum<class "DAQ.lvclass">)
        n271 = Format Into String(format string="%s", error in=w831, ICP1-D0_Channel_Names."Meniscus Pressure Reg PWR - R1" ("DO Channel")) -> (resulting string=w820:string, error out=w815:errorcluster)  [unwired: 1 in]
        n272 = call "Set DO State (manual mode).vi"("error in (no error)"=w815, "State"=TRUE ("Value"), "DO IOName"=w820, "DAQ"=w819) -> ("error out"=w790:errorcluster, "DAQ"=w792:refnum<class "DAQ.lvclass">)  [unwired: 6 in]
        n273 = call-dynamic "Read PersistentXML.vi"("error in (no error)"=w790, "TopLevel in"=w787) -> ("error out"=w789:errorcluster, "PersistentData"=w821:T65)  [unwired: 7 in, 1 out]
        n274 = Unbundle By Name(w821) -> ("MiniscusPressure.Meniscus Pressure Set - R1"=w788:dbl)
        n275 = Format Into String(format string="%s", ICP1-AO_Channel_Names."Meniscus Pressure Set - R1" ("AO Channel")) -> (resulting string=w796:string)  [unwired: 2 in, 1 out]
        n276 = disable-structure shown="Enabled" {
          disable-tunnel: w796 -> [w850 _]
          disable-tunnel: [w849 w851] -> w793
          disable-tunnel: w792 -> [w848 w852]
          disable-tunnel: [w847 w852] -> w791
          disable-tunnel: w789 -> [w846 w851]
          disable-tunnel: w788 -> [w845 _]
          frame Disabled {
            n277 = call "Set AO Data Value (manual mode).vi"("error in (no error)"=w846, "Value"=w845, "AO IOName"=w850, "DAQ"=w848) -> ("error out"=w849:errorcluster, "DAQ"=w847:refnum<class "DAQ.lvclass">)  [unwired: 6 in]
          }
          frame Enabled {
          }
        }
        n278 = call <userlib>:"Wait (ms)__ogtk.vi"("error in (no error)"=w793, "milliseconds to wait"=u32 1000) -> ("error out"=w805:errorcluster)  [unwired: 8 in, 1 out]
        n279 = Format Into String(format string="%s", error in=w805, ICP2-DO_Channel_Names."Meniscus Valve Open - R1" ("DO Channel")) -> (resulting string=w810:string, error out=w813:errorcluster)  [unwired: 1 in]
        n280 = call "Set DO State (automation mode).vi"("error in (no error)"=w813, "State"=TRUE ("Value"), "DO IOName"=w810, "DAQ"=w791) -> ("error out"=w803:errorcluster, "DAQ"=w797:refnum<class "DAQ.lvclass">)  [unwired: 6 in]
        n281 = Format Into String(format string="%s", error in=w803, ICP2-DO_Channel_Names."Ink Flow Valve Open - R1" ("DO Channel")) -> (resulting string=w809:string, error out=w806:errorcluster)  [unwired: 1 in]
        n282 = call "Set DO State (automation mode).vi"("error in (no error)"=w806, "State"=TRUE ("Value"), "DO IOName"=w809, "DAQ"=w797) -> ("error out"=w801:errorcluster, "DAQ"=w799:refnum<class "DAQ.lvclass">)  [unwired: 6 in]
        n283 = disable-structure shown="Enabled" {
          disable-tunnel: w801 -> [w857 w862]
          disable-tunnel: [w856 w862] -> w800
          disable-tunnel: w799 -> [w854 w863]
          disable-tunnel: [w853 w863] -> w798
          frame Enabled {
            n284 = Format Into String(format string="%s", error in=w857, ICP2-DO_Channel_Names."SW_LED - Ink Valve - R1" ("DO Channel")) -> (resulting string=w858:string, error out=w861:errorcluster)  [unwired: 1 in]
            n285 = call "Set DO State (automation mode).vi"("error in (no error)"=w861, "State"=TRUE ("Value"), "DO IOName"=w858, "DAQ"=w854) -> ("error out"=w856:errorcluster, "DAQ"=w853:refnum<class "DAQ.lvclass">)  [unwired: 6 in]
          }
          frame Disabled {
          }
        }
        n286 = disable-structure shown="Disabled" {
          disable-tunnel: [w843 w844] -> w826
          disable-tunnel: w800 -> [w838 w844]
          disable-tunnel: w798 -> [w836 _]
          frame Disabled {
            n287 = Format Into String(format string="%s", error in=w838, ICP2-DO_Channel_Names."Recirc Pump On - R1" ("DO Channel")) -> (resulting string=w842:string, error out=w839:errorcluster)  [unwired: 1 in]
            n288 = call "Set DO State (automation mode).vi"("error in (no error)"=w839, "State"=TRUE ("Value"), "DO IOName"=w842, "DAQ"=w836) -> ("error out"=w843:errorcluster)  [unwired: 6 in, 1 out]
          }
          frame Enabled {
          }
        }
        n289 = Format Into String(format string="P,C,P,PH%s_Enable,%s\nP,C,P,HIB%s_Heat,%s\nP,C,P,PH%s_Heat,%s", error in=w826, w824, w823, w824, w823, w824, w823) -> (resulting string=w829:string, error out=w825:errorcluster)  [unwired: 1 in]
        n290 = Build Array(w829) -> (w822:string[])
        n291 = Bundle By Name(cluster=w827, "GIS Commands"=w822) -> (w828:T61)
        n292 = call <vilib>:"Add State(s) to Queue__JKI_lib_State_Machine.vi"("State(s) in Front (\"\")"="GIS: Send and Execute Command>>0\nTask: Completed" ("State(s) in Front (\"\")"), "State(s) in (\"\")"=w833) -> ("States Out"=w834:string)  [unwired: 13 in]
      }
      frame "API: Enable Ink Ch-2" {
        w898 = TRUE
        w899 = PrinterHeads--Enum."2" ("Head")
        # "#TODO add API to send GIS for enabling Head"
        n293 = Unbundle By Name(w903) -> ("TopLevel in"=w864:refnum<class "TopLevel.lvclass">, "DAQ"=w895:refnum<class "DAQ.lvclass">)
        n294 = Format Into String(format string="%s", error in=w907, ICP1-D0_Channel_Names."Meniscus Pressure Reg PWR - R2" ("DO Channel")) -> (resulting string=w896:string, error out=w891:errorcluster)  [unwired: 1 in]
        n295 = call "Set DO State (manual mode).vi"("error in (no error)"=w891, "State"=TRUE ("Value"), "DO IOName"=w896, "DAQ"=w895) -> ("error out"=w866:errorcluster, "DAQ"=w870:refnum<class "DAQ.lvclass">)  [unwired: 6 in]
        n296 = call-dynamic "Read PersistentXML.vi"("error in (no error)"=w866, "TopLevel in"=w864) -> ("error out"=w865:errorcluster, "PersistentData"=w868:T65)  [unwired: 7 in, 1 out]
        n297 = Unbundle By Name(w868) -> ("MiniscusPressure.Meniscus Pressure Set - R2"=w867:dbl)
        n298 = Format Into String(format string="%s", ICP1-AO_Channel_Names."Meniscus Pressure Set - R2" ("AO Channel")) -> (resulting string=w873:string)  [unwired: 2 in, 1 out]
        n299 = disable-structure shown="Enabled" {
          disable-tunnel: [w917 w919] -> w882
          disable-tunnel: w873 -> [w916 _]
          disable-tunnel: w870 -> [w915 w920]
          disable-tunnel: [w914 w920] -> w869
          disable-tunnel: w867 -> [w912 _]
          disable-tunnel: w865 -> [w911 w919]
          frame Disabled {
            n300 = call "Set AO Data Value (manual mode).vi"("error in (no error)"=w911, "Value"=w912, "AO IOName"=w916, "DAQ"=w915) -> ("error out"=w913:errorcluster, "DAQ"=w914:refnum<class "DAQ.lvclass">)  [unwired: 6 in]
            n301 = call <userlib>:"Wait (ms)__ogtk.vi"("error in (no error)"=w913, "milliseconds to wait"=u32 1000) -> ("error out"=w917:errorcluster)  [unwired: 8 in, 1 out]
          }
          frame Enabled {
          }
        }
        n302 = Format Into String(format string="%s", error in=w882, ICP2-DO_Channel_Names."Meniscus Valve Open - R2" ("DO Channel")) -> (resulting string=w887:string, error out=w890:errorcluster)  [unwired: 1 in]
        n303 = call "Set DO State (automation mode).vi"("error in (no error)"=w890, "State"=TRUE ("Value"), "DO IOName"=w887, "DAQ"=w869) -> ("error out"=w880:errorcluster, "DAQ"=w874:refnum<class "DAQ.lvclass">)  [unwired: 6 in]
        n304 = Format Into String(format string="%s", error in=w880, ICP2-DO_Channel_Names."Ink Flow Valve Open - R2" ("DO Channel")) -> (resulting string=w886:string, error out=w883:errorcluster)  [unwired: 1 in]
        n305 = call "Set DO State (automation mode).vi"("error in (no error)"=w883, "State"=TRUE ("Value"), "DO IOName"=w886, "DAQ"=w874) -> ("error out"=w878:errorcluster, "DAQ"=w876:refnum<class "DAQ.lvclass">)  [unwired: 6 in]
        n306 = disable-structure shown="Enabled" {
          disable-tunnel: w878 -> [w934 w939]
          disable-tunnel: [w933 w939] -> w877
          disable-tunnel: w876 -> [w931 w940]
          disable-tunnel: [w930 w940] -> w875
          frame Enabled {
            n307 = Format Into String(format string="%s", error in=w934, ICP2-DO_Channel_Names."SW_LED - Ink Valve - R2" ("DO Channel")) -> (resulting string=w935:string, error out=w938:errorcluster)  [unwired: 1 in]
            n308 = call "Set DO State (automation mode).vi"("error in (no error)"=w938, "State"=TRUE ("Value"), "DO IOName"=w935, "DAQ"=w931) -> ("error out"=w933:errorcluster, "DAQ"=w930:refnum<class "DAQ.lvclass">)  [unwired: 6 in]
          }
          frame Disabled {
          }
        }
        n309 = disable-structure shown="Enabled" {
          disable-tunnel: [w928 w929] -> w900
          disable-tunnel: w877 -> [w923 w929]
          disable-tunnel: w875 -> [w921 _]
          frame Disabled {
            n310 = Format Into String(format string="%s", error in=w923, ICP2-DO_Channel_Names."Recirc Pump On - R2" ("DO Channel")) -> (resulting string=w927:string, error out=w924:errorcluster)  [unwired: 1 in]
            n311 = call "Set DO State (automation mode).vi"("error in (no error)"=w924, "State"=TRUE ("Value"), "DO IOName"=w927, "DAQ"=w921) -> ("error out"=w928:errorcluster)  [unwired: 6 in, 1 out]
          }
          frame Enabled {
          }
        }
        n312 = Format Into String(format string="P,C,P,PH%s_Enable,%s\nP,C,P,HIB%s_Heat,%s\nP,C,P,PH%s_Heat,%s", error in=w900, w899, w898, w899, w898, w899, w898) -> (resulting string=w905:string, error out=w901:errorcluster)  [unwired: 1 in]
        n313 = Build Array(w905) -> (w897:string[])
        n314 = Bundle By Name(cluster=w903, "GIS Commands"=w897) -> (w904:T61)
        n315 = call <vilib>:"Add State(s) to Queue__JKI_lib_State_Machine.vi"("State(s) in Front (\"\")"="GIS: Send and Execute Command>>0\nTask: Completed" ("State(s) in Front (\"\")"), "State(s) in (\"\")"=w908) -> ("States Out"=w909:string)  [unwired: 13 in]
      }
      frame "API: Enable Ink Ch-3" {
        w975 = TRUE
        w976 = PrinterHeads--Enum."3" ("Head")
        # "#TODO add API to send GIS for enabling Head"
        n316 = Unbundle By Name(w979) -> ("TopLevel in"=w941:refnum<class "TopLevel.lvclass">, "DAQ"=w972:refnum<class "DAQ.lvclass">)
        n317 = Format Into String(format string="%s", error in=w983, ICP1-D0_Channel_Names."Meniscus Pressure Reg PWR - R3" ("DO Channel")) -> (resulting string=w973:string, error out=w968:errorcluster)  [unwired: 1 in]
        n318 = call "Set DO State (manual mode).vi"("error in (no error)"=w968, "State"=TRUE ("Value"), "DO IOName"=w973, "DAQ"=w972) -> ("error out"=w943:errorcluster, "DAQ"=w947:refnum<class "DAQ.lvclass">)  [unwired: 6 in]
        n319 = call-dynamic "Read PersistentXML.vi"("error in (no error)"=w943, "TopLevel in"=w941) -> ("error out"=w942:errorcluster, "PersistentData"=w945:T65)  [unwired: 7 in, 1 out]
        n320 = Unbundle By Name(w945) -> ("MiniscusPressure.Meniscus Pressure Set - R3"=w944:dbl)
        n321 = Format Into String(format string="%s", ICP1-AO_Channel_Names."Meniscus Pressure Set - R3" ("AO Channel")) -> (resulting string=w950:string)  [unwired: 2 in, 1 out]
        n322 = disable-structure shown="Enabled" {
          disable-tunnel: [w994 w996] -> w959
          disable-tunnel: w950 -> [w993 _]
          disable-tunnel: w947 -> [w992 w997]
          disable-tunnel: [w991 w997] -> w946
          disable-tunnel: w944 -> [w989 _]
          disable-tunnel: w942 -> [w988 w996]
          frame Disabled {
            n323 = call "Set AO Data Value (manual mode).vi"("error in (no error)"=w988, "Value"=w989, "AO IOName"=w993, "DAQ"=w992) -> ("error out"=w990:errorcluster, "DAQ"=w991:refnum<class "DAQ.lvclass">)  [unwired: 6 in]
            n324 = call <userlib>:"Wait (ms)__ogtk.vi"("error in (no error)"=w990, "milliseconds to wait"=u32 1000) -> ("error out"=w994:errorcluster)  [unwired: 8 in, 1 out]
          }
          frame Enabled {
          }
        }
        n325 = Format Into String(format string="%s", error in=w959, ICP2-DO_Channel_Names."Meniscus Valve Open - R3" ("DO Channel")) -> (resulting string=w964:string, error out=w967:errorcluster)  [unwired: 1 in]
        n326 = call "Set DO State (automation mode).vi"("error in (no error)"=w967, "State"=TRUE ("Value"), "DO IOName"=w964, "DAQ"=w946) -> ("error out"=w957:errorcluster, "DAQ"=w951:refnum<class "DAQ.lvclass">)  [unwired: 6 in]
        n327 = Format Into String(format string="%s", error in=w957, ICP2-DO_Channel_Names."Ink Flow Valve Open - R3" ("DO Channel")) -> (resulting string=w963:string, error out=w960:errorcluster)  [unwired: 1 in]
        n328 = call "Set DO State (automation mode).vi"("error in (no error)"=w960, "State"=TRUE ("Value"), "DO IOName"=w963, "DAQ"=w951) -> ("error out"=w955:errorcluster, "DAQ"=w953:refnum<class "DAQ.lvclass">)  [unwired: 6 in]
        n329 = disable-structure shown="Enabled" {
          disable-tunnel: w955 -> [w1011 w1016]
          disable-tunnel: [w1010 w1016] -> w954
          disable-tunnel: w953 -> [w1008 w1017]
          disable-tunnel: [w1007 w1017] -> w952
          frame Enabled {
            n330 = Format Into String(format string="%s", error in=w1011, ICP2-DO_Channel_Names."SW_LED - Ink Valve - R3" ("DO Channel")) -> (resulting string=w1012:string, error out=w1015:errorcluster)  [unwired: 1 in]
            n331 = call "Set DO State (automation mode).vi"("error in (no error)"=w1015, "State"=TRUE ("Value"), "DO IOName"=w1012, "DAQ"=w1008) -> ("error out"=w1010:errorcluster, "DAQ"=w1007:refnum<class "DAQ.lvclass">)  [unwired: 6 in]
          }
          frame Disabled {
          }
        }
        n332 = disable-structure shown="Enabled" {
          disable-tunnel: [w1005 w1006] -> w977
          disable-tunnel: w954 -> [w1000 w1006]
          disable-tunnel: w952 -> [w998 _]
          frame Disabled {
            n333 = Format Into String(format string="%s", error in=w1000, ICP2-DO_Channel_Names."Recirc Pump On - R3" ("DO Channel")) -> (resulting string=w1004:string, error out=w1001:errorcluster)  [unwired: 1 in]
            n334 = call "Set DO State (automation mode).vi"("error in (no error)"=w1001, "State"=TRUE ("Value"), "DO IOName"=w1004, "DAQ"=w998) -> ("error out"=w1005:errorcluster)  [unwired: 6 in, 1 out]
          }
          frame Enabled {
          }
        }
        n335 = Format Into String(format string="P,C,P,PH%s_Enable,%s\nP,C,P,HIB%s_Heat,%s\nP,C,P,PH%s_Heat,%s", error in=w977, w976, w975, w976, w975, w976, w975) -> (resulting string=w981:string, error out=w978:errorcluster)  [unwired: 1 in]
        n336 = Build Array(w981) -> (w974:string[])
        n337 = Bundle By Name(cluster=w979, "GIS Commands"=w974) -> (w980:T61)
        n338 = call <vilib>:"Add State(s) to Queue__JKI_lib_State_Machine.vi"("State(s) in Front (\"\")"="GIS: Send and Execute Command>>0\nTask: Completed" ("State(s) in Front (\"\")"), "State(s) in (\"\")"=w985) -> ("States Out"=w986:string)  [unwired: 13 in]
      }
      frame "API: Enable Ink Ch-4" {
        w1052 = TRUE
        w1053 = PrinterHeads--Enum."4" ("Head")
        # "#TODO add API to send GIS for enabling Head"
        n339 = Unbundle By Name(w1055) -> ("TopLevel in"=w1018:refnum<class "TopLevel.lvclass">, "DAQ"=w1049:refnum<class "DAQ.lvclass">)
        n340 = Format Into String(format string="%s", error in=w1061, ICP1-D0_Channel_Names."Meniscus Pressure Reg PWR - R4" ("DO Channel")) -> (resulting string=w1050:string, error out=w1045:errorcluster)  [unwired: 1 in]
        n341 = call "Set DO State (manual mode).vi"("error in (no error)"=w1045, "State"=TRUE ("Value"), "DO IOName"=w1050, "DAQ"=w1049) -> ("error out"=w1021:errorcluster, "DAQ"=w1024:refnum<class "DAQ.lvclass">)  [unwired: 6 in]
        n342 = call-dynamic "Read PersistentXML.vi"("error in (no error)"=w1021, "TopLevel in"=w1018) -> ("error out"=w1020:errorcluster, "PersistentData"=w1022:T65)  [unwired: 7 in, 1 out]
        n343 = Unbundle By Name(w1022) -> ("MiniscusPressure.Meniscus Pressure Set - R4"=w1019:dbl)
        n344 = Format Into String(format string="%s", ICP1-AO_Channel_Names."Meniscus Pressure Set - R4" ("AO Channel")) -> (resulting string=w1027:string)  [unwired: 2 in, 1 out]
        n345 = disable-structure shown="Enabled" {
          disable-tunnel: [w1071 w1073] -> w1036
          disable-tunnel: w1027 -> [w1070 _]
          disable-tunnel: w1024 -> [w1069 w1074]
          disable-tunnel: [w1068 w1074] -> w1023
          disable-tunnel: w1020 -> [w1066 w1073]
          disable-tunnel: w1019 -> [w1065 _]
          frame Disabled {
            n346 = call "Set AO Data Value (manual mode).vi"("error in (no error)"=w1066, "Value"=w1065, "AO IOName"=w1070, "DAQ"=w1069) -> ("error out"=w1067:errorcluster, "DAQ"=w1068:refnum<class "DAQ.lvclass">)  [unwired: 6 in]
            n347 = call <userlib>:"Wait (ms)__ogtk.vi"("error in (no error)"=w1067, "milliseconds to wait"=u32 1000) -> ("error out"=w1071:errorcluster)  [unwired: 8 in, 1 out]
          }
          frame Enabled {
          }
        }
        n348 = Format Into String(format string="%s", error in=w1036, ICP2-DO_Channel_Names."Meniscus Valve Open - R4" ("DO Channel")) -> (resulting string=w1041:string, error out=w1044:errorcluster)  [unwired: 1 in]
        n349 = call "Set DO State (automation mode).vi"("error in (no error)"=w1044, "State"=TRUE ("Value"), "DO IOName"=w1041, "DAQ"=w1023) -> ("error out"=w1034:errorcluster, "DAQ"=w1028:refnum<class "DAQ.lvclass">)  [unwired: 6 in]
        n350 = Format Into String(format string="%s", error in=w1034, ICP2-DO_Channel_Names."Ink Flow Valve Open - R4" ("DO Channel")) -> (resulting string=w1040:string, error out=w1037:errorcluster)  [unwired: 1 in]
        n351 = call "Set DO State (automation mode).vi"("error in (no error)"=w1037, "State"=TRUE ("Value"), "DO IOName"=w1040, "DAQ"=w1028) -> ("error out"=w1032:errorcluster, "DAQ"=w1030:refnum<class "DAQ.lvclass">)  [unwired: 6 in]
        n352 = disable-structure shown="Enabled" {
          disable-tunnel: w1032 -> [w1088 w1093]
          disable-tunnel: [w1087 w1093] -> w1031
          disable-tunnel: w1030 -> [w1085 w1094]
          disable-tunnel: [w1084 w1094] -> w1029
          frame Enabled {
            n353 = Format Into String(format string="%s", error in=w1088, ICP2-DO_Channel_Names."SW_LED - Ink Valve - R4" ("DO Channel")) -> (resulting string=w1089:string, error out=w1092:errorcluster)  [unwired: 1 in]
            n354 = call "Set DO State (automation mode).vi"("error in (no error)"=w1092, "State"=TRUE ("Value"), "DO IOName"=w1089, "DAQ"=w1085) -> ("error out"=w1087:errorcluster, "DAQ"=w1084:refnum<class "DAQ.lvclass">)  [unwired: 6 in]
          }
          frame Disabled {
          }
        }
        n355 = disable-structure shown="Enabled" {
          disable-tunnel: [w1082 w1083] -> w1057
          disable-tunnel: w1031 -> [w1077 w1083]
          disable-tunnel: w1029 -> [w1075 _]
          frame Disabled {
            n356 = Format Into String(format string="%s", error in=w1077, ICP2-DO_Channel_Names."Recirc Pump On - R4" ("DO Channel")) -> (resulting string=w1081:string, error out=w1078:errorcluster)  [unwired: 1 in]
            n357 = call "Set DO State (automation mode).vi"("error in (no error)"=w1078, "State"=TRUE ("Value"), "DO IOName"=w1081, "DAQ"=w1075) -> ("error out"=w1082:errorcluster)  [unwired: 6 in, 1 out]
          }
          frame Enabled {
          }
        }
        n358 = Format Into String(format string="P,C,P,PH%s_Enable,%s\nP,C,P,HIB%s_Heat,%s\nP,C,P,PH%s_Heat,%s", error in=w1057, w1053, w1052, w1053, w1052, w1053, w1052) -> (resulting string=w1059:string, error out=w1058:errorcluster)  [unwired: 1 in]
        n359 = Build Array(w1059) -> (w1051:string[])
        n360 = Bundle By Name(cluster=w1055, "GIS Commands"=w1051) -> (w1056:T61)
        n361 = call <vilib>:"Add State(s) to Queue__JKI_lib_State_Machine.vi"("State(s) in Front (\"\")"="GIS: Send and Execute Command>>0\nTask: Completed" ("State(s) in Front (\"\")"), "State(s) in (\"\")"=w1062) -> ("States Out"=w1063:string)  [unwired: 13 in]
      }
      frame "API: Enable Ink Ch-5" {
        w1129 = TRUE
        w1130 = PrinterHeads--Enum."5" ("Head")
        n362 = Unbundle By Name(w1133) -> ("TopLevel in"=w1095:refnum<class "TopLevel.lvclass">, "DAQ"=w1126:refnum<class "DAQ.lvclass">)
        n363 = Format Into String(format string="%s", error in=w1138, ICP1-D0_Channel_Names."Meniscus Pressure Reg PWR - R5" ("DO Channel")) -> (resulting string=w1127:string, error out=w1122:errorcluster)  [unwired: 1 in]
        n364 = call "Set DO State (manual mode).vi"("error in (no error)"=w1122, "State"=TRUE ("Value"), "DO IOName"=w1127, "DAQ"=w1126) -> ("error out"=w1097:errorcluster, "DAQ"=w1101:refnum<class "DAQ.lvclass">)  [unwired: 6 in]
        n365 = call-dynamic "Read PersistentXML.vi"("error in (no error)"=w1097, "TopLevel in"=w1095) -> ("error out"=w1096:errorcluster, "PersistentData"=w1099:T65)  [unwired: 7 in, 1 out]
        n366 = Unbundle By Name(w1099) -> ("MiniscusPressure.Meniscus Pressure Set - R5"=w1098:dbl)
        n367 = Format Into String(format string="%s", ICP1-AO_Channel_Names."Meniscus Pressure Set - R5" ("AO Channel")) -> (resulting string=w1104:string)  [unwired: 2 in, 1 out]
        n368 = disable-structure shown="Enabled" {
          disable-tunnel: [w1148 w1150] -> w1113
          disable-tunnel: w1104 -> [w1147 _]
          disable-tunnel: w1101 -> [w1146 w1151]
          disable-tunnel: [w1145 w1151] -> w1100
          disable-tunnel: w1098 -> [w1143 _]
          disable-tunnel: w1096 -> [w1142 w1150]
          frame Disabled {
            n369 = call "Set AO Data Value (manual mode).vi"("error in (no error)"=w1142, "Value"=w1143, "AO IOName"=w1147, "DAQ"=w1146) -> ("error out"=w1144:errorcluster, "DAQ"=w1145:refnum<class "DAQ.lvclass">)  [unwired: 6 in]
            n370 = call <userlib>:"Wait (ms)__ogtk.vi"("error in (no error)"=w1144, "milliseconds to wait"=u32 1000) -> ("error out"=w1148:errorcluster)  [unwired: 8 in, 1 out]
          }
          frame Enabled {
          }
        }
        n371 = Format Into String(format string="%s", error in=w1113, ICP2-DO_Channel_Names."Meniscus Valve Open - R5" ("DO Channel")) -> (resulting string=w1118:string, error out=w1121:errorcluster)  [unwired: 1 in]
        n372 = call "Set DO State (automation mode).vi"("error in (no error)"=w1121, "State"=TRUE ("Value"), "DO IOName"=w1118, "DAQ"=w1100) -> ("error out"=w1111:errorcluster, "DAQ"=w1105:refnum<class "DAQ.lvclass">)  [unwired: 6 in]
        n373 = Format Into String(format string="%s", error in=w1111, ICP2-DO_Channel_Names."Ink Flow Valve Open - R5" ("DO Channel")) -> (resulting string=w1117:string, error out=w1114:errorcluster)  [unwired: 1 in]
        n374 = call "Set DO State (automation mode).vi"("error in (no error)"=w1114, "State"=TRUE ("Value"), "DO IOName"=w1117, "DAQ"=w1105) -> ("error out"=w1109:errorcluster, "DAQ"=w1107:refnum<class "DAQ.lvclass">)  [unwired: 6 in]
        n375 = disable-structure shown="Enabled" {
          disable-tunnel: w1109 -> [w1165 w1170]
          disable-tunnel: [w1164 w1170] -> w1108
          disable-tunnel: w1107 -> [w1162 w1171]
          disable-tunnel: [w1161 w1171] -> w1106
          frame Enabled {
            n376 = Format Into String(format string="%s", error in=w1165, ICP2-DO_Channel_Names."SW_LED - Ink Valve - R5" ("DO Channel")) -> (resulting string=w1166:string, error out=w1169:errorcluster)  [unwired: 1 in]
            n377 = call "Set DO State (automation mode).vi"("error in (no error)"=w1169, "State"=TRUE ("Value"), "DO IOName"=w1166, "DAQ"=w1162) -> ("error out"=w1164:errorcluster, "DAQ"=w1161:refnum<class "DAQ.lvclass">)  [unwired: 6 in]
          }
          frame Disabled {
          }
        }
        n378 = disable-structure shown="Enabled" {
          disable-tunnel: [w1159 w1160] -> w1132
          disable-tunnel: w1108 -> [w1154 w1160]
          disable-tunnel: w1106 -> [w1152 _]
          frame Disabled {
            n379 = Format Into String(format string="%s", error in=w1154, ICP2-DO_Channel_Names."Recirc Pump On - R5" ("DO Channel")) -> (resulting string=w1158:string, error out=w1155:errorcluster)  [unwired: 1 in]
            n380 = call "Set DO State (automation mode).vi"("error in (no error)"=w1155, "State"=TRUE ("Value"), "DO IOName"=w1158, "DAQ"=w1152) -> ("error out"=w1159:errorcluster)  [unwired: 6 in, 1 out]
          }
          frame Enabled {
          }
        }
        n381 = Format Into String(format string="P,C,P,PH%s_Enable,%s\nP,C,P,HIB%s_Heat,%s\nP,C,P,PH%s_Heat,%s", error in=w1132, w1130, w1129, w1130, w1129, w1130, w1129) -> (resulting string=w1136:string, error out=w1131:errorcluster)  [unwired: 1 in]
        n382 = Build Array(w1136) -> (w1128:string[])
        n383 = Bundle By Name(cluster=w1133, "GIS Commands"=w1128) -> (w1134:T61)
        n384 = call <vilib>:"Add State(s) to Queue__JKI_lib_State_Machine.vi"("State(s) in Front (\"\")"="GIS: Send and Execute Command>>0\nTask: Completed" ("State(s) in Front (\"\")"), "State(s) in (\"\")"=w1139) -> ("States Out"=w1140:string)  [unwired: 13 in]
      }
      frame "API: Enable Ink Ch-6" {
        w1206 = TRUE
        w1207 = PrinterHeads--Enum."6" ("Head")
        # "#TODO add API to send GIS for enabling Head"
        n385 = Unbundle By Name(w1210) -> ("TopLevel in"=w1172:refnum<class "TopLevel.lvclass">, "DAQ"=w1203:refnum<class "DAQ.lvclass">)
        n386 = Format Into String(format string="%s", error in=w1215, ICP1-D0_Channel_Names."Meniscus Pressure Reg PWR - R6" ("DO Channel")) -> (resulting string=w1204:string, error out=w1199:errorcluster)  [unwired: 1 in]
        n387 = call "Set DO State (manual mode).vi"("error in (no error)"=w1199, "State"=TRUE ("Value"), "DO IOName"=w1204, "DAQ"=w1203) -> ("error out"=w1175:errorcluster, "DAQ"=w1178:refnum<class "DAQ.lvclass">)  [unwired: 6 in]
        n388 = call-dynamic "Read PersistentXML.vi"("error in (no error)"=w1175, "TopLevel in"=w1172) -> ("error out"=w1174:errorcluster, "PersistentData"=w1176:T65)  [unwired: 7 in, 1 out]
        n389 = Unbundle By Name(w1176) -> ("MiniscusPressure.Meniscus Pressure Set - R6"=w1173:dbl)
        n390 = Format Into String(format string="%s", ICP1-AO_Channel_Names."Meniscus Pressure Set - R6" ("AO Channel")) -> (resulting string=w1181:string)  [unwired: 2 in, 1 out]
        n391 = disable-structure shown="Enabled" {
          disable-tunnel: [w1225 w1227] -> w1190
          disable-tunnel: w1181 -> [w1224 _]
          disable-tunnel: w1178 -> [w1223 w1228]
          disable-tunnel: [w1222 w1228] -> w1177
          disable-tunnel: w1174 -> [w1220 w1227]
          disable-tunnel: w1173 -> [w1219 _]
          frame Disabled {
            n392 = call "Set AO Data Value (manual mode).vi"("error in (no error)"=w1220, "Value"=w1219, "AO IOName"=w1224, "DAQ"=w1223) -> ("error out"=w1221:errorcluster, "DAQ"=w1222:refnum<class "DAQ.lvclass">)  [unwired: 6 in]
            n393 = call <userlib>:"Wait (ms)__ogtk.vi"("error in (no error)"=w1221, "milliseconds to wait"=u32 1000) -> ("error out"=w1225:errorcluster)  [unwired: 8 in, 1 out]
          }
          frame Enabled {
          }
        }
        n394 = Format Into String(format string="%s", error in=w1190, ICP2-DO_Channel_Names."Meniscus Valve Open - R6" ("DO Channel")) -> (resulting string=w1195:string, error out=w1198:errorcluster)  [unwired: 1 in]
        n395 = call "Set DO State (automation mode).vi"("error in (no error)"=w1198, "State"=TRUE ("Value"), "DO IOName"=w1195, "DAQ"=w1177) -> ("error out"=w1188:errorcluster, "DAQ"=w1182:refnum<class "DAQ.lvclass">)  [unwired: 6 in]
        n396 = Format Into String(format string="%s", error in=w1188, ICP2-DO_Channel_Names."Ink Flow Valve Open - R6" ("DO Channel")) -> (resulting string=w1194:string, error out=w1191:errorcluster)  [unwired: 1 in]
        n397 = call "Set DO State (automation mode).vi"("error in (no error)"=w1191, "State"=TRUE ("Value"), "DO IOName"=w1194, "DAQ"=w1182) -> ("error out"=w1186:errorcluster, "DAQ"=w1184:refnum<class "DAQ.lvclass">)  [unwired: 6 in]
        n398 = disable-structure shown="Enabled" {
          disable-tunnel: w1186 -> [w1242 w1247]
          disable-tunnel: [w1241 w1247] -> w1185
          disable-tunnel: w1184 -> [w1239 w1248]
          disable-tunnel: [w1238 w1248] -> w1183
          frame Enabled {
            n399 = Format Into String(format string="%s", error in=w1242, ICP2-DO_Channel_Names."SW_LED - Ink Valve - R6" ("DO Channel")) -> (resulting string=w1243:string, error out=w1246:errorcluster)  [unwired: 1 in]
            n400 = call "Set DO State (automation mode).vi"("error in (no error)"=w1246, "State"=TRUE ("Value"), "DO IOName"=w1243, "DAQ"=w1239) -> ("error out"=w1241:errorcluster, "DAQ"=w1238:refnum<class "DAQ.lvclass">)  [unwired: 6 in]
          }
          frame Disabled {
          }
        }
        n401 = disable-structure shown="Enabled" {
          disable-tunnel: [w1236 w1237] -> w1208
          disable-tunnel: w1185 -> [w1231 w1237]
          disable-tunnel: w1183 -> [w1229 _]
          frame Disabled {
            n402 = Format Into String(format string="%s", error in=w1231, ICP2-DO_Channel_Names."Recirc Pump On - R6" ("DO Channel")) -> (resulting string=w1235:string, error out=w1232:errorcluster)  [unwired: 1 in]
            n403 = call "Set DO State (automation mode).vi"("error in (no error)"=w1232, "State"=TRUE ("Value"), "DO IOName"=w1235, "DAQ"=w1229) -> ("error out"=w1236:errorcluster)  [unwired: 6 in, 1 out]
          }
          frame Enabled {
          }
        }
        n404 = Format Into String(format string="P,C,P,PH%s_Enable,%s\nP,C,P,HIB%s_Heat,%s\nP,C,P,PH%s_Heat,%s", error in=w1208, w1207, w1206, w1207, w1206, w1207, w1206) -> (resulting string=w1213:string, error out=w1209:errorcluster)  [unwired: 1 in]
        n405 = Build Array(w1213) -> (w1205:string[])
        n406 = Bundle By Name(cluster=w1210, "GIS Commands"=w1205) -> (w1211:T61)
        n407 = call <vilib>:"Add State(s) to Queue__JKI_lib_State_Machine.vi"("State(s) in Front (\"\")"="GIS: Send and Execute Command>>0\nTask: Completed" ("State(s) in Front (\"\")"), "State(s) in (\"\")"=w1216) -> ("States Out"=w1217:string)  [unwired: 13 in]
      }
      frame "API: Disable Ink Ch-1" {
        w1250 = FALSE
        w1251 = PrinterHeads--Enum."1" ("Head")
        n408 = disable-structure shown="Enabled" {
          disable-tunnel: w1253 -> [w1281 w1287]
          disable-tunnel: w1259 -> [w1273 w1288]
          disable-tunnel: [w1263 w1286] -> w1256
          frame Disabled {
            w1264 = FALSE ("Value")
            w1275 = TRUE ("Wait (F)")
            n409 = Unbundle By Name(w1281) -> ("IO"=w1274:refnum<class "IO.lvclass">)
            n410 = call-dynamic "Set ICP2-DO Changed bit.vi"("Wait (F)"=w1275, "error in (no error)"=w1273, "Value"=w1264, "DO Channel"=ICP2-DO_Channel_Names."Ink Flow Valve Open - R1", "IO in"=w1274) -> ("error out"=w1271:errorcluster, "IO out"=w1272:refnum<class "IO.lvclass">)  [unwired: 5 in]
            n411 = call-dynamic "Set ICP2-DO Changed bit.vi"("Wait (F)"=w1275, "error in (no error)"=w1271, "Value"=w1264, "DO Channel"=ICP2-DO_Channel_Names."Recirc Pump On - R1", "IO in"=w1272) -> ("error out"=w1269:errorcluster, "IO out"=w1270:refnum<class "IO.lvclass">)  [unwired: 5 in]
            n412 = call-dynamic "Set ICP2-DO Changed bit.vi"("Wait (F)"=w1275, "error in (no error)"=w1269, "Value"=w1264, "DO Channel"=ICP2-DO_Channel_Names."Meniscus Valve Open - R1", "IO in"=w1270) -> ("error out"=w1267:errorcluster, "IO out"=w1268:refnum<class "IO.lvclass">)  [unwired: 5 in]
            n413 = call-dynamic "Set ICP2-DO Changed bit.vi"("Wait (F)"=w1275, "error in (no error)"=w1267, "Value"=w1264, "DO Channel"=ICP2-DO_Channel_Names."SW_LED - Ink Valve - R1", "IO in"=w1268) -> ("error out"=w1265:errorcluster, "IO out"=w1266:refnum<class "IO.lvclass">)  [unwired: 5 in]
            n414 = call-dynamic "Set ICP1-DO Changed bit.vi"("Wait (F)"=w1275, "error in (no error)"=w1265, "Value"=w1264, "DO Channel"=ICP1-D0_Channel_Names."Meniscus Pressure Reg PWR - R1", "IO in"=w1266) -> ("error out"=w1263:errorcluster)  [unwired: 5 in, 1 out]
          }
          frame Enabled {
            n415 = Unbundle By Name(w1287) -> ("DAQ"=w1314:refnum<class "DAQ.lvclass">)
            n416 = Format Into String(format string="%s", error in=w1288, ICP2-DO_Channel_Names."Ink Flow Valve Open - R1" ("DO Channel")) -> (resulting string=w1315:string, error out=w1311:errorcluster)  [unwired: 1 in]
            n417 = call "Set DO State (automation mode).vi"("error in (no error)"=w1311, "State"=FALSE ("Value"), "DO IOName"=w1315, "DAQ"=w1314) -> ("error out"=w1309:errorcluster, "DAQ"=w1295:refnum<class "DAQ.lvclass">)  [unwired: 6 in]
            n418 = call <userlib>:"Wait (ms)__ogtk.vi"("error in (no error)"=w1309, "milliseconds to wait"=u32 1000) -> ("error out"=w1296:errorcluster)  [unwired: 8 in, 1 out]
            n419 = Format Into String(format string="%s", error in=w1296, ICP2-DO_Channel_Names."Recirc Pump On - R1" ("DO Channel")) -> (resulting string=w1305:string, error out=w1308:errorcluster)  [unwired: 1 in]
            n420 = call "Set DO State (automation mode).vi"("error in (no error)"=w1308, "State"=FALSE ("Value"), "DO IOName"=w1305, "DAQ"=w1295) -> ("error out"=w1294:errorcluster, "DAQ"=w1289:refnum<class "DAQ.lvclass">)  [unwired: 6 in]
            n421 = Format Into String(format string="%s", error in=w1294, ICP2-DO_Channel_Names."Meniscus Valve Open - R1" ("DO Channel")) -> (resulting string=w1304:string, error out=w1301:errorcluster)  [unwired: 1 in]
            n422 = call "Set DO State (automation mode).vi"("error in (no error)"=w1301, "State"=FALSE ("Value"), "DO IOName"=w1304, "DAQ"=w1289) -> ("error out"=w1293:errorcluster, "DAQ"=w1291:refnum<class "DAQ.lvclass">)  [unwired: 6 in]
            n423 = disable-structure shown="Enabled" {
              disable-tunnel: w1293 -> [w1320 w1325]
              disable-tunnel: [w1319 w1325] -> w1292
              disable-tunnel: w1291 -> [w1318 w1326]
              disable-tunnel: [w1317 w1326] -> w1290
              frame Enabled {
                n424 = Format Into String(format string="%s", error in=w1320, ICP2-DO_Channel_Names."SW_LED - Ink Valve - R1" ("DO Channel")) -> (resulting string=w1321:string, error out=w1324:errorcluster)  [unwired: 1 in]
                n425 = call "Set DO State (automation mode).vi"("error in (no error)"=w1324, "State"=FALSE ("Value"), "DO IOName"=w1321, "DAQ"=w1318) -> ("error out"=w1319:errorcluster, "DAQ"=w1317:refnum<class "DAQ.lvclass">)  [unwired: 6 in]
              }
              frame Disabled {
              }
            }
            n426 = Format Into String(format string="%s", error in=w1292, ICP1-D0_Channel_Names."Meniscus Pressure Reg PWR - R1" ("DO Channel")) -> (resulting string=w1300:string, error out=w1297:errorcluster)  [unwired: 1 in]
            n427 = call "Set DO State (automation mode).vi"("error in (no error)"=w1297, "State"=FALSE ("Value"), "DO IOName"=w1300, "DAQ"=w1290) -> ("error out"=w1286:errorcluster)  [unwired: 6 in, 1 out]
          }
        }
        n428 = Format Into String(format string="P,C,P,PH%s_Enable,%s\nP,C,P,HIB%s_Heat,%s\nP,C,P,PH%s_Heat,%s", error in=w1256, w1251, w1250, w1251, w1250, w1251, w1250) -> (resulting string=w1257:string, error out=w1255:errorcluster)  [unwired: 1 in]
        n429 = Build Array(w1257) -> (w1249:string[])
        n430 = Bundle By Name(cluster=w1253, "GIS Commands"=w1249) -> (w1254:T61)
        n431 = call <vilib>:"Add State(s) to Queue__JKI_lib_State_Machine.vi"("State(s) in Front (\"\")"="GIS: Send and Execute Command>>0\nTask: Completed" ("State(s) in Front (\"\")"), "State(s) in (\"\")"=w1260) -> ("States Out"=w1261:string)  [unwired: 13 in]
      }
      frame "API: Disable Ink Ch-2" {
        w1328 = FALSE
        w1329 = PrinterHeads--Enum."2" ("Head")
        n432 = disable-structure shown="Enabled" {
          disable-tunnel: w1330 -> [w1359 w1361]
          disable-tunnel: w1336 -> [w1351 w1362]
          disable-tunnel: [w1341 w1360] -> w1332
          frame Disabled {
            w1342 = FALSE ("Value")
            w1353 = TRUE ("Wait (F)")
            n433 = Unbundle By Name(w1359) -> ("IO"=w1352:refnum<class "IO.lvclass">)
            n434 = call-dynamic "Set ICP2-DO Changed bit.vi"("Wait (F)"=w1353, "error in (no error)"=w1351, "Value"=w1342, "DO Channel"=ICP2-DO_Channel_Names."Ink Flow Valve Open - R2", "IO in"=w1352) -> ("error out"=w1349:errorcluster, "IO out"=w1350:refnum<class "IO.lvclass">)  [unwired: 5 in]
            n435 = call-dynamic "Set ICP2-DO Changed bit.vi"("Wait (F)"=w1353, "error in (no error)"=w1349, "Value"=w1342, "DO Channel"=ICP2-DO_Channel_Names."Recirc Pump On - R2", "IO in"=w1350) -> ("error out"=w1347:errorcluster, "IO out"=w1348:refnum<class "IO.lvclass">)  [unwired: 5 in]
            n436 = call-dynamic "Set ICP2-DO Changed bit.vi"("Wait (F)"=w1353, "error in (no error)"=w1347, "Value"=w1342, "DO Channel"=ICP2-DO_Channel_Names."Meniscus Valve Open - R2", "IO in"=w1348) -> ("error out"=w1345:errorcluster, "IO out"=w1346:refnum<class "IO.lvclass">)  [unwired: 5 in]
            n437 = call-dynamic "Set ICP2-DO Changed bit.vi"("Wait (F)"=w1353, "error in (no error)"=w1345, "Value"=w1342, "DO Channel"=ICP2-DO_Channel_Names."SW_LED - Ink Valve - R2", "IO in"=w1346) -> ("error out"=w1343:errorcluster, "IO out"=w1344:refnum<class "IO.lvclass">)  [unwired: 5 in]
            n438 = call-dynamic "Set ICP1-DO Changed bit.vi"("Wait (F)"=w1353, "error in (no error)"=w1343, "Value"=w1342, "DO Channel"=ICP1-D0_Channel_Names."Meniscus Pressure Reg PWR - R2", "IO in"=w1344) -> ("error out"=w1341:errorcluster)  [unwired: 5 in, 1 out]
          }
          frame Enabled {
            n439 = Unbundle By Name(w1361) -> ("DAQ"=w1392:refnum<class "DAQ.lvclass">)
            n440 = Format Into String(format string="%s", error in=w1362, ICP2-DO_Channel_Names."Ink Flow Valve Open - R2" ("DO Channel")) -> (resulting string=w1393:string, error out=w1389:errorcluster)  [unwired: 1 in]
            n441 = call "Set DO State (automation mode).vi"("error in (no error)"=w1389, "State"=FALSE ("Value"), "DO IOName"=w1393, "DAQ"=w1392) -> ("error out"=w1387:errorcluster, "DAQ"=w1373:refnum<class "DAQ.lvclass">)  [unwired: 6 in]
            n442 = call <userlib>:"Wait (ms)__ogtk.vi"("error in (no error)"=w1387, "milliseconds to wait"=u32 1000) -> ("error out"=w1374:errorcluster)  [unwired: 8 in, 1 out]
            n443 = Format Into String(format string="%s", error in=w1374, ICP2-DO_Channel_Names."Recirc Pump On - R2" ("DO Channel")) -> (resulting string=w1383:string, error out=w1386:errorcluster)  [unwired: 1 in]
            n444 = call "Set DO State (automation mode).vi"("error in (no error)"=w1386, "State"=FALSE ("Value"), "DO IOName"=w1383, "DAQ"=w1373) -> ("error out"=w1372:errorcluster, "DAQ"=w1367:refnum<class "DAQ.lvclass">)  [unwired: 6 in]
            n445 = Format Into String(format string="%s", error in=w1372, ICP2-DO_Channel_Names."Meniscus Valve Open - R2" ("DO Channel")) -> (resulting string=w1382:string, error out=w1379:errorcluster)  [unwired: 1 in]
            n446 = call "Set DO State (automation mode).vi"("error in (no error)"=w1379, "State"=FALSE ("Value"), "DO IOName"=w1382, "DAQ"=w1367) -> ("error out"=w1371:errorcluster, "DAQ"=w1369:refnum<class "DAQ.lvclass">)  [unwired: 6 in]
            n447 = disable-structure shown="Enabled" {
              disable-tunnel: w1371 -> [w1398 w1403]
              disable-tunnel: [w1397 w1403] -> w1370
              disable-tunnel: w1369 -> [w1396 w1404]
              disable-tunnel: [w1395 w1404] -> w1368
              frame Enabled {
                n448 = Format Into String(format string="%s", error in=w1398, ICP2-DO_Channel_Names."SW_LED - Ink Valve - R2" ("DO Channel")) -> (resulting string=w1399:string, error out=w1402:errorcluster)  [unwired: 1 in]
                n449 = call "Set DO State (automation mode).vi"("error in (no error)"=w1402, "State"=FALSE ("Value"), "DO IOName"=w1399, "DAQ"=w1396) -> ("error out"=w1397:errorcluster, "DAQ"=w1395:refnum<class "DAQ.lvclass">)  [unwired: 6 in]
              }
              frame Disabled {
              }
            }
            n450 = Format Into String(format string="%s", error in=w1370, ICP1-D0_Channel_Names."Meniscus Pressure Reg PWR - R2" ("DO Channel")) -> (resulting string=w1378:string, error out=w1375:errorcluster)  [unwired: 1 in]
            n451 = call "Set DO State (automation mode).vi"("error in (no error)"=w1375, "State"=FALSE ("Value"), "DO IOName"=w1378, "DAQ"=w1368) -> ("error out"=w1360:errorcluster)  [unwired: 6 in, 1 out]
          }
        }
        n452 = Format Into String(format string="P,C,P,PH%s_Enable,%s\nP,C,P,HIB%s_Heat,%s\nP,C,P,PH%s_Heat,%s", error in=w1332, w1329, w1328, w1329, w1328, w1329, w1328) -> (resulting string=w1334:string, error out=w1333:errorcluster)  [unwired: 1 in]
        n453 = Build Array(w1334) -> (w1327:string[])
        n454 = Bundle By Name(cluster=w1330, "GIS Commands"=w1327) -> (w1331:T61)
        n455 = call <vilib>:"Add State(s) to Queue__JKI_lib_State_Machine.vi"("State(s) in Front (\"\")"="GIS: Send and Execute Command>>0\nTask: Completed" ("State(s) in Front (\"\")"), "State(s) in (\"\")"=w1338) -> ("States Out"=w1339:string)  [unwired: 13 in]
      }
      frame "API: Disable Ink Ch-3" {
        w1406 = FALSE
        w1407 = PrinterHeads--Enum."3" ("Head")
        n456 = disable-structure shown="Enabled" {
          disable-tunnel: w1409 -> [w1437 w1440]
          disable-tunnel: w1415 -> [w1429 w1439]
          disable-tunnel: [w1419 w1438] -> w1411
          frame Disabled {
            w1420 = FALSE ("Value")
            w1431 = TRUE ("Wait (F)")
            n457 = Unbundle By Name(w1437) -> ("IO"=w1430:refnum<class "IO.lvclass">)
            n458 = call-dynamic "Set ICP2-DO Changed bit.vi"("Wait (F)"=w1431, "error in (no error)"=w1429, "Value"=w1420, "DO Channel"=ICP2-DO_Channel_Names."Ink Flow Valve Open - R3", "IO in"=w1430) -> ("error out"=w1427:errorcluster, "IO out"=w1428:refnum<class "IO.lvclass">)  [unwired: 5 in]
            n459 = call-dynamic "Set ICP2-DO Changed bit.vi"("Wait (F)"=w1431, "error in (no error)"=w1427, "Value"=w1420, "DO Channel"=ICP2-DO_Channel_Names."Recirc Pump On - R3", "IO in"=w1428) -> ("error out"=w1425:errorcluster, "IO out"=w1426:refnum<class "IO.lvclass">)  [unwired: 5 in]
            n460 = call-dynamic "Set ICP2-DO Changed bit.vi"("Wait (F)"=w1431, "error in (no error)"=w1425, "Value"=w1420, "DO Channel"=ICP2-DO_Channel_Names."Meniscus Valve Open - R3", "IO in"=w1426) -> ("error out"=w1423:errorcluster, "IO out"=w1424:refnum<class "IO.lvclass">)  [unwired: 5 in]
            n461 = call-dynamic "Set ICP2-DO Changed bit.vi"("Wait (F)"=w1431, "error in (no error)"=w1423, "Value"=w1420, "DO Channel"=ICP2-DO_Channel_Names."SW_LED - Ink Valve - R3", "IO in"=w1424) -> ("error out"=w1421:errorcluster, "IO out"=w1422:refnum<class "IO.lvclass">)  [unwired: 5 in]
            n462 = call-dynamic "Set ICP1-DO Changed bit.vi"("Wait (F)"=w1431, "error in (no error)"=w1421, "Value"=w1420, "DO Channel"=ICP1-D0_Channel_Names."Meniscus Pressure Reg PWR - R3", "IO in"=w1422) -> ("error out"=w1419:errorcluster)  [unwired: 5 in, 1 out]
          }
          frame Enabled {
            n463 = Unbundle By Name(w1440) -> ("DAQ"=w1470:refnum<class "DAQ.lvclass">)
            n464 = Format Into String(format string="%s", error in=w1439, ICP2-DO_Channel_Names."Ink Flow Valve Open - R3" ("DO Channel")) -> (resulting string=w1471:string, error out=w1467:errorcluster)  [unwired: 1 in]
            n465 = call "Set DO State (automation mode).vi"("error in (no error)"=w1467, "State"=FALSE ("Value"), "DO IOName"=w1471, "DAQ"=w1470) -> ("error out"=w1465:errorcluster, "DAQ"=w1451:refnum<class "DAQ.lvclass">)  [unwired: 6 in]
            n466 = call <userlib>:"Wait (ms)__ogtk.vi"("error in (no error)"=w1465, "milliseconds to wait"=u32 1000) -> ("error out"=w1452:errorcluster)  [unwired: 8 in, 1 out]
            n467 = Format Into String(format string="%s", error in=w1452, ICP2-DO_Channel_Names."Recirc Pump On - R3" ("DO Channel")) -> (resulting string=w1461:string, error out=w1464:errorcluster)  [unwired: 1 in]
            n468 = call "Set DO State (automation mode).vi"("error in (no error)"=w1464, "State"=FALSE ("Value"), "DO IOName"=w1461, "DAQ"=w1451) -> ("error out"=w1450:errorcluster, "DAQ"=w1445:refnum<class "DAQ.lvclass">)  [unwired: 6 in]
            n469 = Format Into String(format string="%s", error in=w1450, ICP2-DO_Channel_Names."Meniscus Valve Open - R3" ("DO Channel")) -> (resulting string=w1460:string, error out=w1457:errorcluster)  [unwired: 1 in]
            n470 = call "Set DO State (automation mode).vi"("error in (no error)"=w1457, "State"=FALSE ("Value"), "DO IOName"=w1460, "DAQ"=w1445) -> ("error out"=w1449:errorcluster, "DAQ"=w1447:refnum<class "DAQ.lvclass">)  [unwired: 6 in]
            n471 = disable-structure shown="Enabled" {
              disable-tunnel: w1449 -> [w1476 w1481]
              disable-tunnel: [w1475 w1481] -> w1448
              disable-tunnel: w1447 -> [w1474 w1482]
              disable-tunnel: [w1473 w1482] -> w1446
              frame Enabled {
                n472 = Format Into String(format string="%s", error in=w1476, ICP2-DO_Channel_Names."SW_LED - Ink Valve - R3" ("DO Channel")) -> (resulting string=w1477:string, error out=w1480:errorcluster)  [unwired: 1 in]
                n473 = call "Set DO State (automation mode).vi"("error in (no error)"=w1480, "State"=FALSE ("Value"), "DO IOName"=w1477, "DAQ"=w1474) -> ("error out"=w1475:errorcluster, "DAQ"=w1473:refnum<class "DAQ.lvclass">)  [unwired: 6 in]
              }
              frame Disabled {
              }
            }
            n474 = Format Into String(format string="%s", error in=w1448, ICP1-D0_Channel_Names."Meniscus Pressure Reg PWR - R3" ("DO Channel")) -> (resulting string=w1456:string, error out=w1453:errorcluster)  [unwired: 1 in]
            n475 = call "Set DO State (automation mode).vi"("error in (no error)"=w1453, "State"=FALSE ("Value"), "DO IOName"=w1456, "DAQ"=w1446) -> ("error out"=w1438:errorcluster)  [unwired: 6 in, 1 out]
          }
        }
        n476 = Format Into String(format string="P,C,P,PH%s_Enable,%s\nP,C,P,HIB%s_Heat,%s\nP,C,P,PH%s_Heat,%s", error in=w1411, w1407, w1406, w1407, w1406, w1407, w1406) -> (resulting string=w1413:string, error out=w1412:errorcluster)  [unwired: 1 in]
        n477 = Build Array(w1413) -> (w1405:string[])
        n478 = Bundle By Name(cluster=w1409, "GIS Commands"=w1405) -> (w1410:T61)
        n479 = call <vilib>:"Add State(s) to Queue__JKI_lib_State_Machine.vi"("State(s) in Front (\"\")"="GIS: Send and Execute Command>>0\nTask: Completed" ("State(s) in Front (\"\")"), "State(s) in (\"\")"=w1416) -> ("States Out"=w1417:string)  [unwired: 13 in]
      }
      frame "API: Disable Ink Ch-4" {
        w1484 = FALSE
        w1485 = PrinterHeads--Enum."4" ("Head")
        n480 = disable-structure shown="Enabled" {
          disable-tunnel: w1488 -> [w1515 w1518]
          disable-tunnel: w1493 -> [w1507 w1517]
          disable-tunnel: [w1497 w1516] -> w1486
          frame Disabled {
            w1498 = FALSE ("Value")
            w1509 = TRUE ("Wait (F)")
            n481 = Unbundle By Name(w1515) -> ("IO"=w1508:refnum<class "IO.lvclass">)
            n482 = call-dynamic "Set ICP2-DO Changed bit.vi"("Wait (F)"=w1509, "error in (no error)"=w1507, "Value"=w1498, "DO Channel"=ICP2-DO_Channel_Names."Ink Flow Valve Open - R4", "IO in"=w1508) -> ("error out"=w1505:errorcluster, "IO out"=w1506:refnum<class "IO.lvclass">)  [unwired: 5 in]
            n483 = call-dynamic "Set ICP2-DO Changed bit.vi"("Wait (F)"=w1509, "error in (no error)"=w1505, "Value"=w1498, "DO Channel"=ICP2-DO_Channel_Names."Recirc Pump On - R4", "IO in"=w1506) -> ("error out"=w1503:errorcluster, "IO out"=w1504:refnum<class "IO.lvclass">)  [unwired: 5 in]
            n484 = call-dynamic "Set ICP2-DO Changed bit.vi"("Wait (F)"=w1509, "error in (no error)"=w1503, "Value"=w1498, "DO Channel"=ICP2-DO_Channel_Names."Meniscus Valve Open - R4", "IO in"=w1504) -> ("error out"=w1501:errorcluster, "IO out"=w1502:refnum<class "IO.lvclass">)  [unwired: 5 in]
            n485 = call-dynamic "Set ICP2-DO Changed bit.vi"("Wait (F)"=w1509, "error in (no error)"=w1501, "Value"=w1498, "DO Channel"=ICP2-DO_Channel_Names."SW_LED - Ink Valve - R4", "IO in"=w1502) -> ("error out"=w1499:errorcluster, "IO out"=w1500:refnum<class "IO.lvclass">)  [unwired: 5 in]
            n486 = call-dynamic "Set ICP1-DO Changed bit.vi"("Wait (F)"=w1509, "error in (no error)"=w1499, "Value"=w1498, "DO Channel"=ICP1-D0_Channel_Names."Meniscus Pressure Reg PWR - R4", "IO in"=w1500) -> ("error out"=w1497:errorcluster)  [unwired: 5 in, 1 out]
          }
          frame Enabled {
            n487 = Unbundle By Name(w1518) -> ("DAQ"=w1548:refnum<class "DAQ.lvclass">)
            n488 = Format Into String(format string="%s", error in=w1517, ICP2-DO_Channel_Names."Ink Flow Valve Open - R4" ("DO Channel")) -> (resulting string=w1549:string, error out=w1545:errorcluster)  [unwired: 1 in]
            n489 = call "Set DO State (automation mode).vi"("error in (no error)"=w1545, "State"=FALSE ("Value"), "DO IOName"=w1549, "DAQ"=w1548) -> ("error out"=w1543:errorcluster, "DAQ"=w1529:refnum<class "DAQ.lvclass">)  [unwired: 6 in]
            n490 = call <userlib>:"Wait (ms)__ogtk.vi"("error in (no error)"=w1543, "milliseconds to wait"=u32 1000) -> ("error out"=w1530:errorcluster)  [unwired: 8 in, 1 out]
            n491 = Format Into String(format string="%s", error in=w1530, ICP2-DO_Channel_Names."Recirc Pump On - R4" ("DO Channel")) -> (resulting string=w1539:string, error out=w1542:errorcluster)  [unwired: 1 in]
            n492 = call "Set DO State (automation mode).vi"("error in (no error)"=w1542, "State"=FALSE ("Value"), "DO IOName"=w1539, "DAQ"=w1529) -> ("error out"=w1528:errorcluster, "DAQ"=w1523:refnum<class "DAQ.lvclass">)  [unwired: 6 in]
            n493 = Format Into String(format string="%s", error in=w1528, ICP2-DO_Channel_Names."Meniscus Valve Open - R4" ("DO Channel")) -> (resulting string=w1538:string, error out=w1535:errorcluster)  [unwired: 1 in]
            n494 = call "Set DO State (automation mode).vi"("error in (no error)"=w1535, "State"=FALSE ("Value"), "DO IOName"=w1538, "DAQ"=w1523) -> ("error out"=w1527:errorcluster, "DAQ"=w1525:refnum<class "DAQ.lvclass">)  [unwired: 6 in]
            n495 = disable-structure shown="Enabled" {
              disable-tunnel: w1527 -> [w1554 w1559]
              disable-tunnel: [w1553 w1559] -> w1526
              disable-tunnel: w1525 -> [w1552 w1560]
              disable-tunnel: [w1551 w1560] -> w1524
              frame Enabled {
                n496 = Format Into String(format string="%s", error in=w1554, ICP2-DO_Channel_Names."SW_LED - Ink Valve - R4" ("DO Channel")) -> (resulting string=w1555:string, error out=w1558:errorcluster)  [unwired: 1 in]
                n497 = call "Set DO State (automation mode).vi"("error in (no error)"=w1558, "State"=FALSE ("Value"), "DO IOName"=w1555, "DAQ"=w1552) -> ("error out"=w1553:errorcluster, "DAQ"=w1551:refnum<class "DAQ.lvclass">)  [unwired: 6 in]
              }
              frame Disabled {
              }
            }
            n498 = Format Into String(format string="%s", error in=w1526, ICP1-D0_Channel_Names."Meniscus Pressure Reg PWR - R4" ("DO Channel")) -> (resulting string=w1534:string, error out=w1531:errorcluster)  [unwired: 1 in]
            n499 = call "Set DO State (automation mode).vi"("error in (no error)"=w1531, "State"=FALSE ("Value"), "DO IOName"=w1534, "DAQ"=w1524) -> ("error out"=w1516:errorcluster)  [unwired: 6 in, 1 out]
          }
        }
        n500 = Format Into String(format string="P,C,P,PH%s_Enable,%s\nP,C,P,HIB%s_Heat,%s\nP,C,P,PH%s_Heat,%s", error in=w1486, w1485, w1484, w1485, w1484, w1485, w1484) -> (resulting string=w1491:string, error out=w1487:errorcluster)  [unwired: 1 in]
        n501 = Build Array(w1491) -> (w1483:string[])
        n502 = Bundle By Name(cluster=w1488, "GIS Commands"=w1483) -> (w1489:T61)
        n503 = call <vilib>:"Add State(s) to Queue__JKI_lib_State_Machine.vi"("State(s) in Front (\"\")"="GIS: Send and Execute Command>>0\nTask: Completed" ("State(s) in Front (\"\")"), "State(s) in (\"\")"=w1494) -> ("States Out"=w1495:string)  [unwired: 13 in]
      }
      frame "API: Disable Ink Ch-5" {
        w1562 = FALSE
        w1563 = PrinterHeads--Enum."5" ("Head")
        n504 = disable-structure shown="Enabled" {
          disable-tunnel: w1566 -> [w1593 w1594]
          disable-tunnel: w1571 -> [w1585 w1595]
          disable-tunnel: [w1575 w1596] -> w1564
          frame Disabled {
            w1576 = FALSE ("Value")
            w1587 = TRUE ("Wait (F)")
            n505 = Unbundle By Name(w1593) -> ("IO"=w1586:refnum<class "IO.lvclass">)
            n506 = call-dynamic "Set ICP2-DO Changed bit.vi"("Wait (F)"=w1587, "error in (no error)"=w1585, "Value"=w1576, "DO Channel"=ICP2-DO_Channel_Names."Ink Flow Valve Open - R5", "IO in"=w1586) -> ("error out"=w1583:errorcluster, "IO out"=w1584:refnum<class "IO.lvclass">)  [unwired: 5 in]
            n507 = call-dynamic "Set ICP2-DO Changed bit.vi"("Wait (F)"=w1587, "error in (no error)"=w1583, "Value"=w1576, "DO Channel"=ICP2-DO_Channel_Names."Recirc Pump On - R5", "IO in"=w1584) -> ("error out"=w1581:errorcluster, "IO out"=w1582:refnum<class "IO.lvclass">)  [unwired: 5 in]
            n508 = call-dynamic "Set ICP2-DO Changed bit.vi"("Wait (F)"=w1587, "error in (no error)"=w1581, "Value"=w1576, "DO Channel"=ICP2-DO_Channel_Names."Meniscus Valve Open - R5", "IO in"=w1582) -> ("error out"=w1579:errorcluster, "IO out"=w1580:refnum<class "IO.lvclass">)  [unwired: 5 in]
            n509 = call-dynamic "Set ICP2-DO Changed bit.vi"("Wait (F)"=w1587, "error in (no error)"=w1579, "Value"=w1576, "DO Channel"=ICP2-DO_Channel_Names."SW_LED - Ink Valve - R5", "IO in"=w1580) -> ("error out"=w1577:errorcluster, "IO out"=w1578:refnum<class "IO.lvclass">)  [unwired: 5 in]
            n510 = call-dynamic "Set ICP1-DO Changed bit.vi"("Wait (F)"=w1587, "error in (no error)"=w1577, "Value"=w1576, "DO Channel"=ICP1-D0_Channel_Names."Meniscus Pressure Reg PWR - R5", "IO in"=w1578) -> ("error out"=w1575:errorcluster)  [unwired: 5 in, 1 out]
          }
          frame Enabled {
            n511 = Unbundle By Name(w1594) -> ("DAQ"=w1626:refnum<class "DAQ.lvclass">)
            n512 = Format Into String(format string="%s", error in=w1595, ICP2-DO_Channel_Names."Ink Flow Valve Open - R5" ("DO Channel")) -> (resulting string=w1627:string, error out=w1623:errorcluster)  [unwired: 1 in]
            n513 = call "Set DO State (automation mode).vi"("error in (no error)"=w1623, "State"=FALSE ("Value"), "DO IOName"=w1627, "DAQ"=w1626) -> ("error out"=w1621:errorcluster, "DAQ"=w1607:refnum<class "DAQ.lvclass">)  [unwired: 6 in]
            n514 = call <userlib>:"Wait (ms)__ogtk.vi"("error in (no error)"=w1621, "milliseconds to wait"=u32 1000) -> ("error out"=w1608:errorcluster)  [unwired: 8 in, 1 out]
            n515 = Format Into String(format string="%s", error in=w1608, ICP2-DO_Channel_Names."Recirc Pump On - R5" ("DO Channel")) -> (resulting string=w1617:string, error out=w1620:errorcluster)  [unwired: 1 in]
            n516 = call "Set DO State (automation mode).vi"("error in (no error)"=w1620, "State"=FALSE ("Value"), "DO IOName"=w1617, "DAQ"=w1607) -> ("error out"=w1606:errorcluster, "DAQ"=w1601:refnum<class "DAQ.lvclass">)  [unwired: 6 in]
            n517 = Format Into String(format string="%s", error in=w1606, ICP2-DO_Channel_Names."Meniscus Valve Open - R5" ("DO Channel")) -> (resulting string=w1616:string, error out=w1613:errorcluster)  [unwired: 1 in]
            n518 = call "Set DO State (automation mode).vi"("error in (no error)"=w1613, "State"=FALSE ("Value"), "DO IOName"=w1616, "DAQ"=w1601) -> ("error out"=w1605:errorcluster, "DAQ"=w1603:refnum<class "DAQ.lvclass">)  [unwired: 6 in]
            n519 = disable-structure shown="Enabled" {
              disable-tunnel: w1605 -> [w1632 w1637]
              disable-tunnel: [w1631 w1637] -> w1604
              disable-tunnel: w1603 -> [w1630 w1638]
              disable-tunnel: [w1629 w1638] -> w1602
              frame Enabled {
                n520 = Format Into String(format string="%s", error in=w1632, ICP2-DO_Channel_Names."SW_LED - Ink Valve - R5" ("DO Channel")) -> (resulting string=w1633:string, error out=w1636:errorcluster)  [unwired: 1 in]
                n521 = call "Set DO State (automation mode).vi"("error in (no error)"=w1636, "State"=FALSE ("Value"), "DO IOName"=w1633, "DAQ"=w1630) -> ("error out"=w1631:errorcluster, "DAQ"=w1629:refnum<class "DAQ.lvclass">)  [unwired: 6 in]
              }
              frame Disabled {
              }
            }
            n522 = Format Into String(format string="%s", error in=w1604, ICP1-D0_Channel_Names."Meniscus Pressure Reg PWR - R5" ("DO Channel")) -> (resulting string=w1612:string, error out=w1609:errorcluster)  [unwired: 1 in]
            n523 = call "Set DO State (automation mode).vi"("error in (no error)"=w1609, "State"=FALSE ("Value"), "DO IOName"=w1612, "DAQ"=w1602) -> ("error out"=w1596:errorcluster)  [unwired: 6 in, 1 out]
          }
        }
        n524 = Format Into String(format string="P,C,P,PH%s_Enable,%s\nP,C,P,HIB%s_Heat,%s\nP,C,P,PH%s_Heat,%s", error in=w1564, w1563, w1562, w1563, w1562, w1563, w1562) -> (resulting string=w1569:string, error out=w1565:errorcluster)  [unwired: 1 in]
        n525 = Build Array(w1569) -> (w1561:string[])
        n526 = Bundle By Name(cluster=w1566, "GIS Commands"=w1561) -> (w1567:T61)
        n527 = call <vilib>:"Add State(s) to Queue__JKI_lib_State_Machine.vi"("State(s) in Front (\"\")"="GIS: Send and Execute Command>>0\nTask: Completed" ("State(s) in Front (\"\")"), "State(s) in (\"\")"=w1572) -> ("States Out"=w1573:string)  [unwired: 13 in]
      }
      frame "API: Disable Ink Ch-6" {
        w1640 = FALSE
        w1641 = PrinterHeads--Enum."6" ("Head")
        n528 = disable-structure shown="Enabled" {
          disable-tunnel: w1644 -> [w1671 w1674]
          disable-tunnel: w1649 -> [w1663 w1673]
          disable-tunnel: [w1653 w1672] -> w1642
          frame Disabled {
            w1654 = FALSE ("Value")
            w1665 = TRUE ("Wait (F)")
            n529 = Unbundle By Name(w1671) -> ("IO"=w1664:refnum<class "IO.lvclass">)
            n530 = call-dynamic "Set ICP2-DO Changed bit.vi"("Wait (F)"=w1665, "error in (no error)"=w1663, "Value"=w1654, "DO Channel"=ICP2-DO_Channel_Names."Ink Flow Valve Open - R6", "IO in"=w1664) -> ("error out"=w1661:errorcluster, "IO out"=w1662:refnum<class "IO.lvclass">)  [unwired: 5 in]
            n531 = call-dynamic "Set ICP2-DO Changed bit.vi"("Wait (F)"=w1665, "error in (no error)"=w1661, "Value"=w1654, "DO Channel"=ICP2-DO_Channel_Names."Recirc Pump On - R6", "IO in"=w1662) -> ("error out"=w1659:errorcluster, "IO out"=w1660:refnum<class "IO.lvclass">)  [unwired: 5 in]
            n532 = call-dynamic "Set ICP2-DO Changed bit.vi"("Wait (F)"=w1665, "error in (no error)"=w1659, "Value"=w1654, "DO Channel"=ICP2-DO_Channel_Names."Meniscus Valve Open - R6", "IO in"=w1660) -> ("error out"=w1657:errorcluster, "IO out"=w1658:refnum<class "IO.lvclass">)  [unwired: 5 in]
            n533 = call-dynamic "Set ICP2-DO Changed bit.vi"("Wait (F)"=w1665, "error in (no error)"=w1657, "Value"=w1654, "DO Channel"=ICP2-DO_Channel_Names."SW_LED - Ink Valve - R6", "IO in"=w1658) -> ("error out"=w1655:errorcluster, "IO out"=w1656:refnum<class "IO.lvclass">)  [unwired: 5 in]
            n534 = call-dynamic "Set ICP1-DO Changed bit.vi"("Wait (F)"=w1665, "error in (no error)"=w1655, "Value"=w1654, "DO Channel"=ICP1-D0_Channel_Names."Meniscus Pressure Reg PWR - R6", "IO in"=w1656) -> ("error out"=w1653:errorcluster)  [unwired: 5 in, 1 out]
          }
          frame Enabled {
            n535 = Unbundle By Name(w1674) -> ("DAQ"=w1704:refnum<class "DAQ.lvclass">)
            n536 = Format Into String(format string="%s", error in=w1673, ICP2-DO_Channel_Names."Ink Flow Valve Open - R6" ("DO Channel")) -> (resulting string=w1705:string, error out=w1701:errorcluster)  [unwired: 1 in]
            n537 = call "Set DO State (automation mode).vi"("error in (no error)"=w1701, "State"=FALSE ("Value"), "DO IOName"=w1705, "DAQ"=w1704) -> ("error out"=w1699:errorcluster, "DAQ"=w1685:refnum<class "DAQ.lvclass">)  [unwired: 6 in]
            n538 = call <userlib>:"Wait (ms)__ogtk.vi"("error in (no error)"=w1699, "milliseconds to wait"=u32 1000) -> ("error out"=w1686:errorcluster)  [unwired: 8 in, 1 out]
            n539 = Format Into String(format string="%s", error in=w1686, ICP2-DO_Channel_Names."Recirc Pump On - R6" ("DO Channel")) -> (resulting string=w1695:string, error out=w1698:errorcluster)  [unwired: 1 in]
            n540 = call "Set DO State (automation mode).vi"("error in (no error)"=w1698, "State"=FALSE ("Value"), "DO IOName"=w1695, "DAQ"=w1685) -> ("error out"=w1684:errorcluster, "DAQ"=w1679:refnum<class "DAQ.lvclass">)  [unwired: 6 in]
            n541 = Format Into String(format string="%s", error in=w1684, ICP2-DO_Channel_Names."Meniscus Valve Open - R6" ("DO Channel")) -> (resulting string=w1694:string, error out=w1691:errorcluster)  [unwired: 1 in]
            n542 = call "Set DO State (automation mode).vi"("error in (no error)"=w1691, "State"=FALSE ("Value"), "DO IOName"=w1694, "DAQ"=w1679) -> ("error out"=w1683:errorcluster, "DAQ"=w1681:refnum<class "DAQ.lvclass">)  [unwired: 6 in]
            n543 = disable-structure shown="Enabled" {
              disable-tunnel: w1683 -> [w1710 w1715]
              disable-tunnel: [w1709 w1715] -> w1682
              disable-tunnel: w1681 -> [w1708 w1716]
              disable-tunnel: [w1707 w1716] -> w1680
              frame Enabled {
                n544 = Format Into String(format string="%s", error in=w1710, ICP2-DO_Channel_Names."SW_LED - Ink Valve - R6" ("DO Channel")) -> (resulting string=w1711:string, error out=w1714:errorcluster)  [unwired: 1 in]
                n545 = call "Set DO State (automation mode).vi"("error in (no error)"=w1714, "State"=FALSE ("Value"), "DO IOName"=w1711, "DAQ"=w1708) -> ("error out"=w1709:errorcluster, "DAQ"=w1707:refnum<class "DAQ.lvclass">)  [unwired: 6 in]
              }
              frame Disabled {
              }
            }
            n546 = Format Into String(format string="%s", error in=w1682, ICP1-D0_Channel_Names."Meniscus Pressure Reg PWR - R6" ("DO Channel")) -> (resulting string=w1690:string, error out=w1687:errorcluster)  [unwired: 1 in]
            n547 = call "Set DO State (automation mode).vi"("error in (no error)"=w1687, "State"=FALSE ("Value"), "DO IOName"=w1690, "DAQ"=w1680) -> ("error out"=w1672:errorcluster)  [unwired: 6 in, 1 out]
          }
        }
        n548 = Format Into String(format string="P,C,P,PH%s_Enable,%s\nP,C,P,HIB%s_Heat,%s\nP,C,P,PH%s_Heat,%s", error in=w1642, w1641, w1640, w1641, w1640, w1641, w1640) -> (resulting string=w1647:string, error out=w1643:errorcluster)  [unwired: 1 in]
        n549 = Build Array(w1647) -> (w1639:string[])
        n550 = Bundle By Name(cluster=w1644, "GIS Commands"=w1639) -> (w1645:T61)
        n551 = call <vilib>:"Add State(s) to Queue__JKI_lib_State_Machine.vi"("State(s) in Front (\"\")"="GIS: Send and Execute Command>>0\nTask: Completed" ("State(s) in Front (\"\")"), "State(s) in (\"\")"=w1650) -> ("States Out"=w1651:string)  [unwired: 13 in]
      }
      frame "---------- Tasks ----------" {
      }
      frame "Task: Completed" {
        n552 = Unbundle By Name(w1728) -> ("API Executed Event"=w1726:refnum<user-event>, "Tasks"=w1725:T15[], "Current Task. Return Value"=w1722:variant, "TopLevel in"=w1721:refnum<class "TopLevel.lvclass">)
        n553 = Empty Array?(array=w1725) -> (empty?=w1727:bool)
        n554 = case shown="False" w1727 {
          tunnel: w1726 -> [w1740 _]
          tunnel: w1725 -> [w1741 _]
          tunnel: w1723 -> [w1731 w1742]
          tunnel: [w1738 w1742] -> w1724
          tunnel: w1722 -> [w1735 _]
          tunnel: w1721 -> [w1733 _]
          frame False {
            n555 = Index Array(array=w1741) -> (element=w1739:T15)  [unwired: 1 in]
            n556 = Bundle By Name(cluster=w1739, "Task.Task State"=API_Task_State."Completed", "Return Value"=w1735) -> (w1737:T15)
            n557 = call-dynamic "SetTopLevel Busy_StatusChangedEvent.vi"("error in (no error)"=w1731, "Status.Busy"=FALSE, "TopLevel in"=w1733) -> ("error out"=w1732:errorcluster)  [unwired: 7 in, 1 out]
            n558 = Generate User Event(user event=w1740, event data cluster=w1737, error in=w1732) -> (error out=w1738:errorcluster)  [unwired: 1 in, 1 out]
          }
          frame True {
          }
        }
      }
      frame "Task: Check Timeout" {
        n559 = Unbundle By Name(w1750) -> ("API Executed Event"=w1748:refnum<user-event>, "Task Start ms"=w1743:u32, "Tasks"=w1745:T15[])
        n560 = Index Array(array=w1745) -> (element=w1744:T15)  [unwired: 1 in]
        n561 = Empty Array?(array=w1745) -> (empty?=w1749:bool)
        n562 = case shown="False" w1749 {
          tunnel: w1748 -> [w1754 _]
          tunnel: w1746 -> [w1760 w1769]
          tunnel: [w1755 w1769] -> w1747
          tunnel: w1744 -> [w1759 _]
          tunnel: w1743 -> [w1763 _]
          frame False {
            n563 = Unbundle By Name(w1759) -> ("Task.Timeout (ms)"=w1761:u32)
            n564 = Tick Count (ms)() -> (millisecond timer value=w1753:u32)
            n565 = Subtract(x=w1753, y=w1763) -> (x-y=w1762:u32)
            n566 = Bundle By Name(cluster=w1759, "Task.Task State"=API_Task_State."Errored") -> (w1757:T15)
            n567 = Greater Or Equal?(x=w1762, y=w1761) -> (x >= y?=w1756:bool)
            n568 = case shown="True" w1756 {
              tunnel: w1760 -> [w1764 w1768]
              tunnel: w1757 -> [_ w1766]
              tunnel: [w1764 w1767] -> w1755
              tunnel: w1754 -> [_ w1765]
              frame False {
              }
              frame True {
                n569 = Generate User Event(user event=w1765, event data cluster=w1766, error in=w1768) -> (error out=w1767:errorcluster)  [unwired: 1 in, 1 out]
              }
            }
          }
          frame True {
          }
        }
      }
      frame "Task: Check Pending" {
        n570 = Unbundle By Name(w1770) -> ("API Executed Event"=w1779:refnum<user-event>, "Task Start ms"=w1776:u32, "Tasks"=w1775:T15[])
        n571 = Empty Array?(array=w1775) -> (empty?=w1780:bool)
        n572 = case shown="False" w1780 {
          tunnel: w1779 -> [_ _]
          tunnel: w1777 -> [w1790 w1799]
          tunnel: [w1788 w1799] -> w1778
          tunnel: w1776 -> [_ _]
          tunnel: w1775 -> [w1797 _]
          tunnel: [w1787 _] -> w1772
          tunnel: w1770 -> [w1786 w1798]
          tunnel: [w1784 w1798] -> w1771
          frame False {
            n573 = Index Array(array=w1797) -> (element=w1792:T15)  [unwired: 1 in]
            n574 = Unbundle By Name(w1792) -> ("Command"=w1791:variant)
            n575 = Variant To Data(error in=w1790, type=T13 {"Command"=enum."Execute Printer Commands", "Arguments"="", "Data"=variant} ("API Command Cluster"), Variant=w1791) -> (data=w1782:T13, error out=w1789:errorcluster)
            n576 = Unbundle By Name(w1782) -> ("Command"=w1794:T14, "Arguments"=w1793:string)
            n577 = Tick Count (ms)() -> (millisecond timer value=w1785:u32)
            n578 = Bundle By Name(cluster=w1786, "TO"=100, "Task Start ms"=w1785, "Current Task"=w1782) -> (w1784:T61)
            n579 = Format Into String(format string="API: %s>>%s", error in=w1789, w1794, w1793) -> (resulting string=w1787:string, error out=w1788:errorcluster)  [unwired: 1 in]
          }
          frame True {
          }
        }
        n580 = call <vilib>:"Add State(s) to Queue__JKI_lib_State_Machine.vi"("State(s) in Front (\"\")"=w1772, "State(s) in (\"\")"=w1773) -> ("States Out"=w1774:string)  [unwired: 13 in]
      }
      frame "Task: Remove on Error" {
        n581 = Unbundle By Name(w1808) -> ("TopLevel in"=w1800:refnum<class "TopLevel.lvclass">, "API Return Event"=w1810:refnum<user-event>, "Tasks"=w1809:T15[])
        n582 = for {
          tunnel: w1810 -> [w1820]
          tunnel: w1809 -> [w1819] mode=indexing
          shift-right: [w1814] -> w1802
          shift-left: w1807 -> [w1815]
          n583 = Get Date/Time In Seconds() -> (seconds since 1Jan1904=w1816:timestamp)
          n584 = Bundle By Name(cluster=w1819, "Task.Task State"=API_Task_State."Errored", "Task.Time Stamp"=w1816) -> (w1818:T15)
          n585 = Generate User Event(user event=w1820, event data cluster=w1818, error in=w1815) -> (error out=w1814:errorcluster)  [unwired: 1 in, 1 out]
        }
        n586 = Bundle By Name(cluster=w1808, "TO"=-1, "Tasks"=T15[] []) -> (w1806:T61)
        n587 = call-dynamic "SetTopLevel Busy_StatusChangedEvent.vi"("error in (no error)"=w1802, "Status.Busy"=FALSE, "TopLevel in"=w1800) -> ("error out"=w1801:errorcluster)  [unwired: 7 in, 1 out]
        n588 = call <vilib>:"Add State(s) to Queue__JKI_lib_State_Machine.vi"("State(s) in (\"\")"=w1811) -> ("States Out"=w1812:string)  [unwired: 14 in]
      }
      frame "-------System----------" {
      }
      frame "System: Shutdown" {
        n589 = Unbundle By Name(w1835) -> ("TopLevel in"=w1834:refnum<class "TopLevel.lvclass">)
        n590 = property class="TopLevel.lvclass"(reference=w1834) -> ("Methods:Accessors:DAQ"=w1833:refnum<class "DAQ.lvclass">, "Methods:Accessors:Motor Controller"=w1831:refnum<class "Motor Controller.lvclass">, "Methods:Accessors:GIS Printer"=w1829:refnum<class "GIS Printer.lvclass">, "Methods:Accessors:DLP2"=w1827:refnum<class "DLP2.lvclass">)  [unwired: 1 in, 2 out]
        n591 = call "Shutdown.vi"("error in (no error)"=w1826, "DLP2 in"=w1827) -> ("error out"=w1825:errorcluster)  [unwired: 8 in, 1 out]
        n592 = call "Shutdown.vi"("error in (no error)"=w1826, "GIS Printer in"=w1829) -> ("error out"=w1828:errorcluster)  [unwired: 8 in, 1 out]
        n593 = call "Shutdown.vi"("error in (no error)"=w1826, "Motor Controller in"=w1831) -> ("error out"=w1830:errorcluster)  [unwired: 8 in, 1 out]
        n594 = call "Shutdown.vi"("error in (no error)"=w1826, "DAQ"=w1833) -> ("error out"=w1832:errorcluster)  [unwired: 8 in, 1 out]
        n595 = flat-sequence {
          tunnel: w1830 -> [_]
          tunnel: w1828 -> [_]
          tunnel: w1825 -> [_]
          frame #0 {
          }
        }
      }
      frame "System: ReturnLaunchState" {
        n596 = case shown="Default" w1838 {
          tunnel: [TD_LaunchState--enum."Stopped" ("LaunchState") TD_LaunchState--enum."Started" ("LaunchState") _] -> w1839
          frame "Stopped" {
          }
          frame "Started" {
          }
          frame Default {
          }
        }
        n597 = Unbundle By Name(w1841) -> ("LaunchData"=w1842:refnum<user-event>)
        n598 = Bundle By Name(cluster=T57 {"Time Stamp"=timestamp(0 s since 1904-01-01), "LaunchState"=enum."Stopped", "Error"={"status"=FALSE, "code"=0, "source"=""}} ("LaunchData"), "LaunchState"=w1839) -> (w1843:T57)
        n599 = Generate User Event(user event=w1842, event data cluster=w1843) -> ()  [unwired: 2 in, 2 out]
      }
      frame "System: Launch Main UI" {
        n600 = Unbundle By Name(w1851) -> ("TopLevel in"=w1850:refnum<class "TopLevel.lvclass">)
        n601 = vi-ref "TopLevel.lvclass:Digilens DLP Gen2 UI .vi"() -> (w1860:refnum<vi>)
        n602 = property class="VI"(reference=w1860) -> ("Name"=w1859:string)  [unwired: 1 in, 2 out]
        n603 = Open VI Reference(type specifier VI Refnum (for type only)=refnum<vi> refnum, vi path=w1859, options=128, error in (no error)=w1852) -> (vi reference=w1856:refnum<vi>, error out=w1855:errorcluster)  [unwired: 2 in]
        n604 = call-by-ref "Start Asynchronous Call"(reference=w1856, error in=w1855, "TopLevel In"=w1850) -> (reference out=w1854:refnum<vi>, error out=w1853:errorcluster)  [unwired: 10 in, 1 out]
        n605 = Close Reference(reference=w1854, error in (no error)=w1853) -> (error out=w1849:errorcluster)
        n606 = call <vilib>:"Clear Errors.vi"("error in (no error)"=w1849) -> ()  [unwired: 5 in, 2 out]
      }
      frame "System: Start" {
        w1879 = refnum<class "DAQ.lvclass"> refnum  # DAQ
        n607 = flat-sequence {
          tunnel: [w1908] -> w1894
          tunnel: w1895 -> [w1908]
          frame #0 {
            n608 = call "TopLevel_Ref_FGV.vi"("Action"=enum16{"Get", "Set", "Init"}."Init") -> ()  [unwired: 10 in, 1 out]
          }
        }
        n609 = call-dynamic "Create.vi"("error in (no error)"=w1894, "TopLevel in"=refnum<class "TopLevel.lvclass"> refnum) -> ("error out"=w1902:errorcluster, "TopLevel out"=w1901:refnum<class "TopLevel.lvclass">)  [unwired: 8 in]
        n610 = call-dynamic "Create.vi"("error in (no error)"=w1902, "Motor Controller in"=refnum<class "Motor Controller.lvclass"> refnum) -> ("error out"=w1898:errorcluster, "Motor Controller out"=w1892:refnum<class "Motor Controller.lvclass">)  [unwired: 8 in]
        n611 = call-dynamic "Create.vi"("error in (no error)"=w1898, "TopLevel in"=refnum<class "IO.lvclass"> refnum) -> ("error out"=w1896:errorcluster, "TopLevel out"=w1899:refnum<class "IO.lvclass">)  [unwired: 8 in]
        n612 = Unbundle By Name(w1891) -> ("Digilens IPLC Config"=w1871:T38, "MasterConfigurationDLPC2"=w1872:T3, "DLP"=w1868:T18)
        n613 = call-dynamic "Create.vi"("error in (no error)"=w1896, "TopLevel in"=refnum<class "GIS Printer.lvclass"> refnum) -> ("error out"=w1884:errorcluster, "TopLevel out"=w1893:refnum<class "GIS Printer.lvclass">)  [unwired: 8 in]
        n614 = call "Startup.vi"("Database in"=refnum<class "Database.lvclass"> refnum ("Database.lvclass")) -> ("Database out"=w1883:refnum<class "Database.lvclass">)  [unwired: 9 in, 1 out]
        n615 = call "Startup.vi"("error in (no error)"=w1884, "Database"=w1883, "DLP2 in"=refnum<class "DLP2.lvclass"> refnum ("DLP2.lvclass")) -> ("error out"=w1875:errorcluster, "DLP2 out"=w1882:refnum<class "DLP2.lvclass">)  [unwired: 7 in]
        n616 = Unbundle By Name(w1871) -> ("DAQ Settings"=w1870:T44)
        n617 = call "Initialize Class.vi"("error in (no error)"=w1875, "DataQueues in"=refnum<class "DataQueues.lvclass"> refnum ("DataQueues.lvclass")) -> ("error out"=w1874:errorcluster, "DataQueues out"=w1873:refnum<class "DataQueues.lvclass">)  [unwired: 8 in]
        n618 = call "Startup.vi"("DataQueues"=w1873, "error in (no error)"=w1874, "DAQ Settings*"=w1870, "DAQ"=w1879) -> ("error out"=w1878:errorcluster, "DAQ"=w1877:refnum<class "DAQ.lvclass">)  [unwired: 6 in]
        n619 = property class="TopLevel.lvclass"(reference=w1901, "Methods:Accessors:Digilens Config"=w1871, "Methods:Accessors:DLP2Config"=w1872, "Methods:Accessors:PrinterInitializationXML"=w1868, "Methods:Accessors:Motor Controller"=w1892, "Methods:Accessors:IO"=w1899, "Methods:Accessors:GIS Printer"=w1893, "Methods:Accessors:Database"=w1883, "Methods:Accessors:DLP2"=w1882, "Methods:Accessors:DAQ"=w1877) -> (reference out=w1867:refnum<class "TopLevel.lvclass">, error out=w1865:errorcluster)  [unwired: 1 in]
        n620 = call "PopulateHeadPropertiesInConfigDict.vi"("error in (no error)"=w1865, "TopLevel in"=w1867) -> ("error out"=w1864:errorcluster, "InkType Directory"=→"InkType Directory":T1[], "TopLevel out"=w1866:refnum<class "TopLevel.lvclass">)  [unwired: 7 in]
        n621 = property class="TopLevel.lvclass"(reference=w1866, error in=w1864) -> (reference out=w1890:refnum<class "TopLevel.lvclass">, "Methods:Accessors:Motor Controller"=w1889:refnum<class "Motor Controller.lvclass">, "Methods:Accessors:IO"=w1888:refnum<class "IO.lvclass">, "Methods:Accessors:GIS Printer"=w1887:refnum<class "GIS Printer.lvclass">, "Methods:Accessors:Database"=w1881:refnum<class "Database.lvclass">, "Methods:Accessors:DLP2"=w1880:refnum<class "DLP2.lvclass">, "Methods:Accessors:DAQ"=w1869:refnum<class "DAQ.lvclass">)  [unwired: 1 out]
        n622 = Bundle By Name(cluster=w1891, "Motor Controller"=w1892, "TopLevel in"=w1890, "Motor Controller"=w1889, "IO"=w1888, "GIS Printer"=w1887, "Database"=w1881, "DLP2"=w1880, "DAQ"=w1869) -> (w1904:T61)
      }
      frame "System: Launch Processes" {
        n623 = Unbundle By Name(w1934) -> ("TopLevel in"=w1911:refnum<class "TopLevel.lvclass">)
        n624 = call "Launch Login Process.vi"("error in (no error)"=w1913, "TopLevel in"=w1911) -> ("error out"=w1912:errorcluster, "TopLevel out"=w1910:refnum<class "TopLevel.lvclass">)  [unwired: 8 in]
        n625 = property class="TopLevel.lvclass"(reference=w1910, error in=w1912) -> (reference out=w1917:refnum<class "TopLevel.lvclass">, error out=w1915:errorcluster, "Methods:Accessors:Motor Controller"=w1933:refnum<class "Motor Controller.lvclass">, "Methods:Accessors:IO"=w1929:refnum<class "IO.lvclass">, "Methods:Accessors:GIS Printer"=w1916:refnum<class "GIS Printer.lvclass">, "Methods:Accessors:Database"=w1925:refnum<class "Database.lvclass">, "Methods:Accessors:DAQ"=w1921:refnum<class "DAQ.lvclass">, "Methods:Accessors:DLP2"=w1919:refnum<class "DLP2.lvclass">)
        n626 = disable-structure shown="Enabled" {
          disable-tunnel: w1917 -> [w1940 _]
          disable-tunnel: w1916 -> [w1939 _]
          disable-tunnel: w1915 -> [w1938 w1941]
          disable-tunnel: [w1937 w1941] -> w1914
          frame Enabled {
            n627 = call "StartupGISErrorMonitor.vi"("error in (no error)"=w1938, "GIS Printer"=w1939, "TopLevel in"=w1940) -> ("error out"=w1937:errorcluster)  [unwired: 8 in]
          }
          frame Disabled {
          }
        }
        n628 = disable-structure shown="Enabled" {
          disable-tunnel: [w1950 w1951] -> w1931
          disable-tunnel: w1929 -> [w1949 _]
          disable-tunnel: w1915 -> [w1948 w1951]
          disable-tunnel: w1917 -> [w1947 _]
          frame Disabled {
            n629 = call "Startup IO.vi"("error in (no error)"=w1948, "Methods:Accessors:IO"=w1949, "TopLevel in"=w1947) -> ("error out"=w1950:errorcluster)  [unwired: 8 in]
          }
          frame Enabled {
          }
        }
        n630 = disable-structure shown="Enabled" {
          disable-tunnel: w1925 -> [w1945 _]
          disable-tunnel: [w1944 w1946] -> w1924
          disable-tunnel: w1915 -> [w1943 w1946]
          disable-tunnel: w1917 -> [w1942 _]
          frame Disabled {
            n631 = call "Launch Process.vi"("error in (no error)"=w1943, "TopLevel"=w1942, "Database in"=w1945) -> ("error out"=w1944:errorcluster)  [unwired: 5 in, 3 out]
          }
          frame Enabled {
          }
        }
        n632 = call "StartupGISPollProcess.vi"("error in (no error)"=w1915, "GIS Printer"=w1916, "TopLevel in"=w1917) -> ("error out"=w1922:errorcluster)  [unwired: 8 in]
        n633 = call "Startup Motor.vi"("error in (no error)"=w1915, "Motor Controller"=w1933, "TopLevel in"=w1917) -> ("error out"=w1932:errorcluster)  [unwired: 8 in]
        n634 = call "StartupGIS.vi"("error in (no error)"=w1915, "GIS Printer"=w1916, "TopLevel in"=w1917) -> ("error out"=w1930:errorcluster)  [unwired: 8 in]
        n635 = call "Launch Process.vi"("error in (no error)"=w1915, "TopLevel"=w1917, "DAQ"=w1921) -> ("error out"=w1923:errorcluster)  [unwired: 7 in, 1 out]
        n636 = call "Launch Monitor Process.vi"("error in (no error)"=w1915, "TopLevel"=w1917, "DAQ"=w1921) -> ("error out"=w1920:errorcluster)  [unwired: 7 in, 1 out]
        n637 = call "Launcher.vi"("error in (no error)"=w1915, "TopLevel"=w1917, "DLP2 in"=w1919) -> ("error out"=w1918:errorcluster)  [unwired: 7 in, 1 out]
        n638 = Merge Errors(w1932, w1931, w1930, w1922, w1914, w1924, w1923, w1920, w1918) -> (w1927:errorcluster)
        n639 = flat-sequence {
          tunnel: w1927 -> [w1953]
          tunnel: w1917 -> [w1952]
          tunnel: [w1953] -> w1928
          tunnel: [w1957] -> w1926
          tunnel: w1928 -> [w1958]
          frame #0 {
            n640 = call "TopLevel_Ref_FGV.vi"("Action"=enum16{"Get", "Set", "Init"}."Set", "TopLevel In"=w1952) -> ()  [unwired: 9 in, 1 out]
          }
          frame #1 {
            n641 = call <vilib>:"Wait at Rendezvous.vi"("error in (no error)"=w1958, "ms timeout (-1)"=20000, "rendezvous"="rendezvous ref") -> ("error out"=w1957:errorcluster)  [unwired: 2 in, 2 out]
          }
        }
      }
      frame "------------GIS------------" {
      }
      frame "WaitAsync" {
        n642 = Unbundle By Name(w1968) -> ("Idle Mode"=w1965:bool, "IdleTimer"=w1967:dbl)
        n643 = case shown="\"Initialize\"" w1975 {
          tunnel: [TRUE ("reset") _] -> w1974
          tunnel: w1967 -> [w1980 w1985]
          tunnel: [w1979 w1984] -> w1966
          frame "Initialize" {
            n644 = Multiply(x=w1980, y=1000.0) -> (x*y=w1981:dbl)
            n645 = To Unsigned Long Integer(number=w1981) -> (unsigned 32bit integer=w1979:u32)
          }
          frame Default {
            n646 = Multiply(x=w1985, y=1000.0) -> (x*y=w1986:dbl)
            n647 = To Unsigned Long Integer(number=w1986) -> (unsigned 32bit integer=w1984:u32)
          }
        }
        n648 = Not(x=w1965) -> (.not. x?=w1963:bool)
        n649 = call <userlib>:"Periodic Trigger__ogtk.vi"("time (ms)"=w1966, "reset"=w1974) -> ("Triggered"=w1973:bool)  [unwired: 11 in, 2 out]
        n650 = Or(x=w1963, y=w1973) -> (x .or. y?=w1964:bool)
        n651 = Select(t="", s=w1964, f="Idle\nWaitAsync>>Count") -> (s? t:f=w1970:string)
        n652 = call <vilib>:"Add State(s) to Queue__JKI_lib_State_Machine.vi"("State(s) in Front (\"\")"=w1970, "State(s) in (\"\")"=w1972) -> ("States Out"=w1976:string)  [unwired: 13 in]
      }
      frame "MoveStage" {
        n653 = Unbundle By Name(w1992) -> ("Motor Controller"=w1991:refnum<class "Motor Controller.lvclass">)
        n654 = case shown="\"Home\"" w1990 {
          tunnel: w1988 -> [w1995 w1997 w2002 w2007]
          tunnel: [w1995 w1998 w2003 w2008] -> w1989
          tunnel: w1991 -> [_ w1999 w2004 w2009]
          frame Default {
          }
          frame "Laminate" {
            n655 = call "Laminate API.vi"("Wait (F)"=TRUE, "error in (no error)"=w1997, "Motor Controller in"=w1999) -> ("error out"=w1998:errorcluster)  [unwired: 6 in, 2 out]
          }
          frame "Home" {
            n656 = call "API_HomeStage.vi"("Timeout (ms)"=u32 600000, "Wait (F)"=TRUE, "error in (no error)"=w2002, "Motor Controller in"=w2004) -> ("error out"=w2003:errorcluster)  [unwired: 5 in, 2 out]
          }
          frame "Load" {
            n657 = call "API_StageMoveToLoadPosition.vi"("Timeout (ms)"=u32 600000, "Wait (F)"=TRUE, "error in (no error)"=w2007, "Motor Controller in"=w2009) -> ("error out"=w2008:errorcluster)  [unwired: 5 in, 2 out]
          }
        }
      }
      frame "GIS: Execute Command" {
        n658 = Unbundle By Name(w2019) -> ("Printer Command File Path"=w2018:path, "GIS Printer"=w2017:refnum<class "GIS Printer.lvclass">, "TopLevel in"=w2014:refnum<class "TopLevel.lvclass">, "PrintScanTrk.CurrentScan"=w2011:i32)
        n659 = call-dynamic "Set PrintCount_StatusChangedEvent.vi"("error in (no error)"=w2012, "Status.PrintNo"=w2011, "TopLevel in"=w2014) -> ("error out"=w2013:errorcluster)  [unwired: 7 in, 1 out]
        n660 = Read from Text File(file (use dialog)=w2018, error in=w2013) -> (text=w2030:string, error out=w2021:errorcluster)  [unwired: 2 in, 2 out]
        n661 = Spreadsheet String To Array(delimiter (Tab)="\n", format string="", spreadsheet string=w2030, array type (2D Dbl)=string[] []) -> (array=w2026:string[])
        n662 = call-poly <userlib>:"Filter 1D Array__ogtk.vi"("items to filter"="", "array"=w2026) -> ("filtered array"=w2025:string[])  [unwired: 4 in, 1 out]
        n663 = call-dynamic "ResetTCPCommands&Responses_GIS Printer.vi"("error in (no error)"=w2021, "GIS Printer In"=w2017) -> ("error out"=w2022:errorcluster, "GIS Printer Out"=w2023:refnum<class "GIS Printer.lvclass">)  [unwired: 8 in]
        n664 = for {
          shift-right: [w2044] -> w2020
          shift-left: w2022 -> [w2043]
          tunnel: w2025 -> [w2042] mode=indexing
          shift-right: [w2040] -> _
          shift-left: w2023 -> [w2041]
          tunnel: [w2037] -> w2016 mode=indexing
          shift-right: [w2038] -> _
          shift-left: bool[] [] -> [w2039]
          tunnel: [w2033] -> w2010 mode=indexing
          i -> [w2033]
          stop <- w2034 stop-if-true
          n665 = call "API_ExecuteCommand.vi"("Timeout (ms)"=u32 10000, "Wait (F)"=TRUE, "error in (no error)"=w2043, "String"=w2042, "GIS Printer in"=w2041) -> ("error out"=w2044:errorcluster, "Aborted"=w2034:bool, "TimedOut"=w2037:bool, "GIS Printer out"=w2040:refnum<class "GIS Printer.lvclass">)  [unwired: 3 in]
          n666 = Build Array (concatenate)(w2039, w2037) -> (w2038:bool[])
          "appended array" <- w2038
        }
        "TO" <- w2016
        n667 = flat-sequence {
          tunnel: w2010 -> [_]
          frame #0 {
          }
        }
      }
      frame "GIS: Send and Execute Command" {
        n668 = Decimal String To Number(string=w2048) -> (number=w2047:i32)  [unwired: 2 in, 1 out]
        n669 = Unbundle By Name(w2057) -> ("GIS Commands"=w2046:string[], "GIS Printer"=w2056:refnum<class "GIS Printer.lvclass">, "TopLevel in"=w2053:refnum<class "TopLevel.lvclass">, "PPScanTrk.CurrentScan"=w2051:i32)
        n670 = call-dynamic "Set PrintCount_StatusChangedEvent.vi"("error in (no error)"=w2052, "Status.PrintNo"=w2051, "TopLevel in"=w2053) -> ("error out"=w2049:errorcluster)  [unwired: 7 in, 1 out]
        n671 = Index Array(array=w2046, index=w2047) -> (element=w2045:string)
        n672 = Spreadsheet String To Array(delimiter (Tab)="\n", format string="", spreadsheet string=w2045, array type (2D Dbl)=string[] []) -> (array=w2063:string[])
        n673 = call-poly <userlib>:"Filter 1D Array__ogtk.vi"("items to filter"="", "array"=w2063) -> ("filtered array"=w2062:string[])  [unwired: 4 in, 1 out]
        n674 = call-dynamic "ResetTCPCommands&Responses_GIS Printer.vi"("error in (no error)"=w2049, "GIS Printer In"=w2056) -> ("error out"=w2059:errorcluster, "GIS Printer Out"=w2060:refnum<class "GIS Printer.lvclass">)  [unwired: 8 in]
        n675 = for {
          shift-right: [w2080] -> w2058
          shift-left: w2059 -> [w2079]
          tunnel: w2062 -> [w2078] mode=indexing
          shift-right: [w2076] -> _
          shift-left: w2060 -> [w2077]
          tunnel: [w2073] -> w2055 mode=indexing
          shift-right: [w2074] -> _
          shift-left: bool[] [] -> [w2075]
          tunnel: [w2069] -> w2050 mode=indexing
          i -> [w2069]
          stop <- w2070 stop-if-true
          n676 = call "API_ExecuteCommand.vi"("Timeout (ms)"=u32 10000, "Wait (F)"=TRUE, "error in (no error)"=w2079, "String"=w2078, "GIS Printer in"=w2077) -> ("error out"=w2080:errorcluster, "Aborted"=w2070:bool, "TimedOut"=w2073:bool, "GIS Printer out"=w2076:refnum<class "GIS Printer.lvclass">)  [unwired: 3 in]
          n677 = Build Array (concatenate)(w2075, w2073) -> (w2074:bool[])
        }
        "TO 2" <- w2055
        n678 = flat-sequence {
          tunnel: w2050 -> [_]
          frame #0 {
          }
        }
      }
      frame "GIS: Execute GIS Command String" {
        n679 = Unbundle By Name(w2090) -> ("GIS Printer"=w2089:refnum<class "GIS Printer.lvclass">, "TopLevel in"=w2086:refnum<class "TopLevel.lvclass">, "PPScanTrk.CurrentScan"=w2084:i32)
        n680 = call-dynamic "Set PrintCount_StatusChangedEvent.vi"("error in (no error)"=w2085, "Status.PrintNo"=w2084, "TopLevel in"=w2086) -> ("error out"=w2082:errorcluster)  [unwired: 7 in, 1 out]
        n681 = Spreadsheet String To Array(delimiter (Tab)="\n", format string="", spreadsheet string=w2081, array type (2D Dbl)=string[] []) -> (array=w2096:string[])
        n682 = call-poly <userlib>:"Filter 1D Array__ogtk.vi"("items to filter"="", "array"=w2096) -> ("filtered array"=w2095:string[])  [unwired: 4 in, 1 out]
        n683 = call-dynamic "ResetTCPCommands&Responses_GIS Printer.vi"("error in (no error)"=w2082, "GIS Printer In"=w2089) -> ("error out"=w2092:errorcluster, "GIS Printer Out"=w2093:refnum<class "GIS Printer.lvclass">)  [unwired: 8 in]
        n684 = for {
          shift-right: [w2113] -> w2091
          shift-left: w2092 -> [w2112]
          tunnel: w2095 -> [w2111] mode=indexing
          shift-right: [w2109] -> _
          shift-left: w2093 -> [w2110]
          tunnel: [w2106] -> w2088 mode=indexing
          shift-right: [w2107] -> _
          shift-left: bool[] [] -> [w2108]
          tunnel: [w2102] -> w2083 mode=indexing
          i -> [w2102]
          stop <- w2103 stop-if-true
          n685 = call "API_ExecuteCommand.vi"("Timeout (ms)"=u32 10000, "Wait (F)"=TRUE, "error in (no error)"=w2112, "String"=w2111, "GIS Printer in"=w2110) -> ("error out"=w2113:errorcluster, "Aborted"=w2103:bool, "TimedOut"=w2106:bool, "GIS Printer out"=w2109:refnum<class "GIS Printer.lvclass">)  [unwired: 3 in]
          n686 = Build Array (concatenate)(w2108, w2106) -> (w2107:bool[])
        }
        "TO 3" <- w2088
        n687 = flat-sequence {
          tunnel: w2083 -> [_]
          frame #0 {
          }
        }
      }
      frame "---------Purge---------" {
      }
      frame "Purge: Send Command" {
        # "This is a part of the prepurge routine. But the purge oeration is called as step 1 before the GIS script is executed next"
        n688 = Unbundle By Name(w2125) -> ("IO"=w2124:refnum<class "IO.lvclass">, "Pre Purge API Data.Purge Channel Name"=w2123:T37, "Pre Purge API Data.PurgeDuration (s)"=w2122:dbl)
        n689 = call-dynamic "Purge PH - API.vi"("Timeout (ms)"=u32 5000, "Wait (F)"=TRUE, "error in (no error)"=w2120, "Duration (s)"=w2122, "ICP1-DO Channel Name"=w2123, "IO in"=w2124) -> ("error out"=w2121:errorcluster)  [unwired: 4 in, 1 out]
      }
      frame "Pre Purge: Wait" {
        n690 = Unbundle By Name(w2131) -> ("Pre Purge API Data.Duration (s)"=w2130:dbl)
        n691 = Multiply(x=w2130, y=u32 1000 ("milliseconds to wait")) -> (x*y=w2128:dbl)
        n692 = call <userlib>:"Wait (ms)__ogtk.vi"("error in (no error)"=w2135, "milliseconds to wait"=w2128) -> ("error out"=w2132:errorcluster)  [unwired: 8 in, 1 out]
      }
      frame "Action: SyncWait" {
        n693 = Fract/Exp String To Number(string=w2137) -> (number=w2136:dbl)  [unwired: 3 in, 1 out]
        n694 = Multiply(x=w2136, y=u32 1000 ("milliseconds to wait")) -> (x*y=w2138:dbl)
        n695 = call <userlib>:"Wait (ms)__ogtk.vi"("error in (no error)"=w2144, "milliseconds to wait"=w2138) -> ("error out"=w2141:errorcluster)  [unwired: 8 in, 1 out]
      }
      frame "Prime: Wait" {
        n696 = Unbundle By Name(w2148) -> ("PrinterModeAPI Data.PurgeDuration (s)"=w2147:dbl)
        n697 = Multiply(x=w2147, y=u32 1000 ("milliseconds to wait")) -> (x*y=w2145:dbl)
        n698 = call <userlib>:"Wait (ms)__ogtk.vi"("error in (no error)"=w2152, "milliseconds to wait"=w2145) -> ("error out"=w2149:errorcluster)  [unwired: 8 in, 1 out]
      }
      frame "-------Action --------" {
      }
      frame "Action: Send Event" {
        n699 = Unbundle By Name(w2160) -> ("TopLevel in"=w2159:refnum<class "TopLevel.lvclass">)
        n700 = call <vilib>:"Parse State Queue__JKI_lib_State_Machine.vi"("State Queue"=w2162) -> ("Current State"=w2163:string, "Arguments"=w2161:string)  [unwired: 12 in, 1 out]
        n701 = case shown="\"CalPrintCount\"" w2163 {
          tunnel: w2161 -> [_ w2170]
          tunnel: w2159 -> [_ w2171]
          tunnel: w2157 -> [w2166 w2168]
          tunnel: [w2166 w2167] -> w2158
          frame Default {
          }
          frame "CalPrintCount" {
            n702 = Decimal String To Number(string=w2170) -> (number=w2169:i32)  [unwired: 2 in, 1 out]
            n703 = call-dynamic "Set CalPrintCount_StatusChangedEvent.vi"("error in (no error)"=w2168, "Status.PrintNo"=w2169, "TopLevel in"=w2171) -> ("error out"=w2167:errorcluster)  [unwired: 7 in, 1 out]
          }
        }
      }
      frame "Action: SendStatusPollEnable" {
        n704 = Scan From String(input string=w2178, default 1=FALSE) -> (output 1=w2176:bool)  [unwired: 3 in, 3 out]
        n705 = Unbundle By Name(w2173) -> ("TopLevel in"=w2172:refnum<class "TopLevel.lvclass">)
        n706 = call "PollStatusEnable.vi"("error in (no error)"=w2174, "PollEnable"=w2176, "TopLevel in"=w2172) -> ("error out"=w2175:errorcluster)  [unwired: 7 in, 1 out]
      }
      frame "Purge: Set DOChannel" {
        n707 = Unbundle By Name(w2193) -> ("DAQ"=w2192:refnum<class "DAQ.lvclass">, "PrinterModeAPI Data.PurgeDuration (s)"=w2188:dbl)
        n708 = call "Set DO State (manual mode).vi"("error in (no error)"=w2190, "State"=TRUE, "DO IOName"=w2181, "DAQ"=w2192) -> ("error out"=w2191:errorcluster, "DAQ"=w2184:refnum<class "DAQ.lvclass">)  [unwired: 6 in]
        n709 = Multiply(x=w2188, y=1000.0) -> (x*y=w2186:dbl)
        n710 = call <userlib>:"Wait (ms)__ogtk.vi"("error in (no error)"=w2191, "milliseconds to wait"=w2186) -> ("error out"=w2183:errorcluster)  [unwired: 8 in, 1 out]
        n711 = call "Set DO State (manual mode).vi"("error in (no error)"=w2183, "State"=FALSE, "DO IOName"=w2181, "DAQ"=w2184) -> ("error out"=w2182:errorcluster)  [unwired: 6 in, 1 out]
      }
      frame "Action: Purge" {
        # "API: Purge PH"
        n712 = Unbundle By Name(w2202) -> ("PrinterModeAPI Data.Head"=w2197:T10, "PrinterModeAPI Data.PurgeDuration (s)"=w2201:dbl, "DAQ"=w2198:refnum<class "DAQ.lvclass">)
        n713 = case shown="\"-1\", Default" w2197 {
          tunnel: [ICP1-D0_Channel_Names."Purge Valve Open - R1" ("ICP1-DO Channel Name") ICP1-D0_Channel_Names."Purge Valve Open - R2" ("ICP1-DO Channel Name") ICP1-D0_Channel_Names."Purge Valve Open - R3" ("ICP1-DO Channel Name") ICP1-D0_Channel_Names."Purge Valve Open - R4" ("ICP1-DO Channel Name") ICP1-D0_Channel_Names."Purge Valve Open - R5" ("ICP1-DO Channel Name") ICP1-D0_Channel_Names."Purge Valve Open - R6" ("ICP1-DO Channel Name") ICP1-D0_Channel_Names."None" ("ICP1-DO Channel Name")] -> w2196
          frame "1" {
          }
          frame "2" {
          }
          frame "3" {
          }
          frame "4" {
          }
          frame "5" {
          }
          frame "6" {
          }
          frame "-1", Default {
          }
        }
        n714 = Format Into String(format string="%s", error in=w2203, w2196) -> (resulting string=w2215:string, error out=w2212:errorcluster)  [unwired: 1 in]
        n715 = Multiply(x=w2201, y=u32 1000 ("milliseconds to wait")) -> (x*y=w2199:dbl)
        n716 = call "Set DO State (manual mode).vi"("error in (no error)"=w2212, "State"=TRUE ("Value"), "DO IOName"=w2215, "DAQ"=w2198) -> ("error out"=w2211:errorcluster, "DAQ"=w2205:refnum<class "DAQ.lvclass">)  [unwired: 6 in]
        n717 = call <userlib>:"Wait (ms)__ogtk.vi"("error in (no error)"=w2211, "milliseconds to wait"=w2199) -> ("error out"=w2206:errorcluster)  [unwired: 8 in, 1 out]
        n718 = Format Into String(format string="%s", error in=w2206, w2196) -> (resulting string=w2207:string, error out=w2210:errorcluster)  [unwired: 1 in]
        n719 = call "Set DO State (manual mode).vi"("error in (no error)"=w2210, "State"=FALSE ("Value"), "DO IOName"=w2207, "DAQ"=w2205) -> ("error out"=w2204:errorcluster)  [unwired: 6 in, 1 out]
      }
      frame "Action: Exit Async Loop" {
        n720 = call <vilib>:"Add State to Queue with vData.vi"("queue in"=w2228, "state in"="Exit", "error in"=w2225) -> ("error out"=w2226:errorcluster)  [unwired: 9 in, 3 out]
      }
    }
  }
  n721 = while {
    tunnel: w12 -> [w2239]
    tunnel: w11 -> [w2238]
    shift-right: [w2234] -> _
    shift-left: T12 {"Initialized"=FALSE, "LogFileFolder"=path "", "LogFile"=path ""} -> [w2235]
    tunnel: [w2232] -> w5
    stop <- w2236 stop-if-true
    n722 = call <vilib>:"Get Next Queued State with vData.vi"("queue in"=w2239, "error in (no error)"=w2238) -> ("queue out"=w2233:refnum<queue>, "Next State"=w2241:string, "queued msg"=w2240:string, "error out"=w2237:errorcluster)  [unwired: 7 in, 3 out]
    n723 = case shown="\"InitializeLog\"" w2241 {
      tunnel: w2240 -> [_ _ _ _ _ _]
      tunnel: w2237 -> [w2246 w2252 w2253 w2255 w2257 w2261]
      tunnel: [_ _ _ _ TRUE _] -> w2236
      tunnel: w2235 -> [w2248 w2251 w2254 w2256 w2258 w2263]
      tunnel: [w2245 w2251 w2254 w2256 w2258 w2263] -> w2234
      tunnel: w2233 -> [_ _ _ _ _ w2262]
      tunnel: [w2242 w2249 w2253 w2255 w2257 w2260] -> w2232
      frame "InitializeLog" {
        n724 = Unbundle By Name(w2248) -> ("LogFileFolder"=w2247:path)
        n725 = call "Create Log File.vi"("error in (no error)"=w2246, "LogFile Folder"=w2247) -> ("error out"=w2242:errorcluster, "new file path"=w2244:path)  [unwired: 8 in]
        n726 = Bundle By Name(cluster=w2248, "LogFile"=w2244, "Initialized"=TRUE) -> (w2245:T12)
      }
      frame "LogData" {
        n727 = Unbundle By Name(w2251) -> ("LogFile"=w2250:path)
        n728 = call "Log Data to File.vi"("error in (no error)"=w2252, "Path"=w2250) -> ("error out"=w2249:errorcluster)  [unwired: 8 in, 1 out]
      }
      frame Default {
      }
      frame "Initialize" {
      }
      frame "Exit" {
      }
      frame "", "Idle" {
        n729 = Unbundle By Name(w2263) -> ("Initialized"=w2264:bool)
        n730 = case shown="False" w2264 {
          tunnel: w2262 -> [_ w2268]
          tunnel: w2261 -> [w2265 w2267]
          tunnel: [w2265 w2266] -> w2260
          frame False {
          }
          frame True {
            n731 = call <vilib>:"Add State to Queue with vData.vi"("queue in"=w2268, "state in"="LogData", "error in"=w2267) -> ("error out"=w2266:errorcluster)  [unwired: 9 in, 3 out]
          }
        }
      }
    }
  }
  n732 = Merge Errors(w6, w5) -> (w4:errorcluster)
  "error out" <- w4
  n733 = flat-sequence {
    tunnel: w7 -> [w2271]
    tunnel: w4 -> [_]
    tunnel: [w2270] -> _
    frame #0 {
      n734 = Unbundle By Name(w2271) -> ("LaunchData"=w2272:refnum<user-event>)
      n735 = Generate User Event(user event=w2272, event data cluster=T57 {"Time Stamp"=timestamp(0 s since 1904-01-01), "LaunchState"=enum."Stopped", "Error"={"status"=FALSE, "code"=0, "source"=""}} ("LaunchData")) -> (error out=w2270:errorcluster)  [unwired: 2 in, 1 out]
    }
  }
  n736 = call "FG - FilePathnames.vi"() -> ("FilePaths out"=w2:T64)  [unwired: 4 in, 1 out]
  n737 = Unbundle By Name(w2) -> ()  [unwired: 1 out]
  "TopLevel out" <- "TopLevel in"
